vi "DetectorTest_MainV10.vi"() -> ()   [LabVIEW 2012]
uses:
  Detector IV/SMU Settings.ctl
  <vilib>/Utility/file.llb/Write To Spreadsheet File (string).vi
  <vilib>/Utility/file.llb/Read From Spreadsheet File (string).vi
  <vilib>/Utility/file.llb/Read From Spreadsheet File (DBL).vi
  <vilib>/Analysis/NI_AALBase.lvlib
panel:
  in  "Current Session":timestamp=timestamp(3388091786.578125 s since 1904-01-01)
  in  "new sesh":bool
  out "RecipeID":string="58"
  in  "Sweep Direction (Keysight)":i32(ring) items=["Up", "Down"]
  in  "Auto Adjust Compliance?":bool
  out "Auto Temp Counter":i32
  out "iteration":i32
  in  "Temp Data":T1={"Ambient Temperature"=20.38176242851337, "Chuck Set Temperature"=35.0} {"Chuck Set Temperature" format="%#.1g"; "Ambient Temperature" format="%#.1g"}
  in  "Wafer Info 3":T2={"Cell Name (Automatic)"="Open_Diode_1000", "Package"="", "Coating"="FOR_AIR", "Comment"="IV test for lot 371", "Flash Setup"="5500_99_03p5", "Hrs under test"=0.0}
  out "TempCounter":i32
  out "WaferCounter":i32
  in  "Profile Z":bool
  in  "Load Wafer":bool
  out "Raw Test Skipped":bool=TRUE
  out "device name w skip":string="Open_Diode_1000(skip)"
  in  "4-wire":bool
  out "Laser Counter":i32
  out "Output Power (mW)":dbl
  out "Counter":i32
  out "NameList":string[](array[string])
  in  "Wafer Info Flash 2":T3={"Cell Name"="5500_130_05", "Package"="", "Coating"="", "LRC?"=enum."J2", "Comment"="", "Hours Under Test"=0.0}
  in  "Parameters Flash 2":T4 {"Voc" format="%#_4g"; "Isc" format="%#_4g"; "FF" format="%#_4g"; "Imax" format="%#_4g"; "Vmax" format="%#_4g"; "Pmax" format="%#_4g"; "Itest" format="%#_4g"}
  in  "Wafer Info Flash":T3={"Cell Name"="Open_Diode_1000", "Package"="", "Coating"="", "LRC?"=enum."J2", "Comment"="", "Hours Under Test"=0.0}
  in  "Parameters Flash":T4={"Voc"=0.0, "Isc"=0.0, "FF"=0.0, "Vtest"=0.0, "Imax"=0.0, "Vmax"=0.0, "Pmax"=0.0, "Itest"=0.0, "Efficiency"=0.0, "Incident Power"=5.674, "Power Density (W/cm^2)"=0.6679328011361159, "Cell Area (cm²)"=849486.6535, "Number of AM1.5D Suns"=0.0, "Input Current (mA)"=40.0, "Equivalent 1 sun Jsc"=0.0} {"Voc" format="%#_4g"; "Isc" format="%#_4g"; "FF" format="%#_4g"; "Imax" format="%#_4g"; "Vmax" format="%#_4g"; "Pmax" format="%#_4g"; "Itest" format="%#_4g"}
  out "RawData file":path=path "C:/Users/Flash/Desktop/Data/Detector test data/SJC_ENG_371_4-GaAs/A-3719-2-A/Raw Data/A-3719-2-A_Open_Diode_1000_20180913075240.csv"
  out "Fine Cell Clusters":T5(array[cluster])=[{"Cell Name"="Open_Diode_1000", "X-coord"=46800.0, "Y-coord"=22950.0, "Area"=849486.6535, "Grid Shadowing"=0.0, "Xdim"=500.0, "Ydim"=500.0, "Mesa Area"=785398.1634}]
  out "Selected Data":cluster{dbl[], dbl[]}={[nan, nan, nan, nan, nan, nan, nan, nan, nan, nan, nan, nan, nan, nan, nan, nan, nan, nan, nan, nan, nan, nan, nan, nan, nan, nan, nan, nan, nan, nan, nan, nan, nan, nan, nan, nan, nan, nan, nan, nan, nan, nan, nan, nan, nan, nan, nan, nan, nan, nan, nan, nan, nan, nan, nan, nan, nan, nan, nan, nan, nan, nan, nan, nan, nan, nan, nan, nan, nan, nan, nan, nan, nan, nan, nan, nan, nan, nan, nan, nan, nan, nan, nan, nan], [nan, nan, nan, nan, nan, nan, nan, nan, nan, nan, nan, nan, nan, nan, nan, nan, nan, nan, nan, nan, nan, nan, nan, nan, nan, nan, nan, nan, nan, nan, nan, nan, nan, nan, nan, nan, nan, nan, nan, nan, nan, nan, nan, nan, nan, nan, nan, nan, nan, nan, nan, nan, nan, nan, nan, nan, nan, nan, nan, nan, nan, nan, nan, nan, nan, nan, nan, nan, nan, nan, nan, nan, nan, nan, nan, nan, nan, nan, nan, nan, nan, nan, nan, nan]}
  in  "Test Results 2":T6
  in  "Session Info 2":T7={"V set"=-1.0, "I compliance"=0.001, "J set"=0.01, "I set"=0.0, "V compliance"=1.0, "Laser Power (mW)"=0.0, "TestID"=0, "Session Time"=timestamp(0 s since 1904-01-01), "Operator"="Radek"} {"V compliance" format="%#_6f"; "I compliance" format="%#_6e"}
  in  "Die Info 2":T8={"Device Name"="", "ActiveArea_um2"=3848.451, "MesaArea_um2"=3848.451, "x"=0.0, "y"=0.0}
  in  "Wafer Info 2":T9
  in  "Test Results":T6={"I meas"=-1.83245e-12, "V meas"=6.01176, "Time"=timestamp(3619695820.3512325 s since 1904-01-01)}
  in  "Session Info":T7={"V set"=-6.0, "I compliance"=0.001, "J set"=0.01, "I set"=1.9634954079999997e-05, "V compliance"=6.0, "Laser Power (mW)"=0.0, "TestID"=1794, "Session Time"=timestamp(3619695160.866512 s since 1904-01-01), "Operator"="sswifter"} {"V compliance" format="%#_6f"; "I compliance" format="%#_6e"}
  in  "Die Info":T8={"Device Name"="Open_Diode_1000", "ActiveArea_um2"=849486.6535, "MesaArea_um2"=785398.1634, "x"=26800.0, "y"=72950.0}
  in  "Wafer Info":T9={"Wafer Name"="A-3719-2-A", "Scribe"="BJ325-089", "Mask"="PH001", "Lot"="SJC_ENG_371_4-GaAs"}
  in  "Name Array":string[](array[string])=["Wafer name", "Scribe", "Mask", "Lot", "Device name", "Active Area", "Mesa Area", "x", "y", "Imeas", "Vmeas", "Time", "Vset", "Icomp", "Jset", "Iset", "Vcomp", "Laser Power", "TestID", "SessionTime", "Operator", "Selected"]
  in  "TestID file":path=path "C:/Users/Flash/Documents/GitHub/labview/Detector IV/rawtest_log.csv"
  in  "update wafer":bool
  in  "Lot":string="SJC_ENG_382_4-GaAs"
  in  "Laser Current (mA)":dbl
  in  "Device Name":string="Open_Diode_3000"
  in  "Scribe":string="BP769-030XT"
  in  "MesaArea_um2":dbl=7068583.471
  out "Status":string="idle"
  out "error out":errorcluster
  in  "error in (no error)":errorcluster
  out "Manaul Plot 1":cluster{"V manual":dbl[], dbl[]}[](array[cluster])=[{"V manual"=[-0.1, -0.089741, -0.07949, -0.06923, -0.05897, -0.04872, -0.03846, -0.02821, -0.017951, -0.00769, 0.00256, 0.012819, 0.02308, 0.03333, 0.043589, 0.05385, 0.0641, 0.074359, 0.084619, 0.09487, 0.10513, 0.115379, 0.125639, 0.135899, 0.14615, 0.156409, 0.16667, 0.176919, 0.187179, 0.19744, 0.207691, 0.217949, 0.22821, 0.23846, 0.248719], [2.22891e-05, 1.84968e-05, 1.52529e-05, 1.24377e-05, 1.00378e-05, 7.9393e-06, 6.043e-06, 4.31347e-06, 2.71019e-06, 1.17492e-06, 3.32763e-07, 1.84722e-06, 3.41691e-06, 5.05009e-06, 6.8287e-06, 8.72018e-06, 1.07805e-05, 1.3036e-05, 1.55303e-05, 1.81749e-05, 2.11963e-05, 2.4467e-05, 2.80104e-05, 3.19022e-05, 3.6041e-05, 4.04887e-05, 4.53187e-05, 5.05479e-05, 5.60681e-05, 6.20483e-05, 6.8299e-05, 7.49314e-05, 8.20298e-05, 8.95166e-05, 9.72544e-05]}, {"V manual"=[-0.1, nan, nan, nan, nan, nan, nan, nan, nan, nan, nan, nan, nan, nan, nan, nan, nan, nan, nan, nan, nan, nan, nan, nan, nan, nan, nan, nan, nan, nan, nan, nan, nan, nan, nan, nan, nan, nan, nan, nan], [2.2117733333333333e-05, nan, nan, nan, nan, nan, nan, nan, nan, nan, nan, nan, nan, nan, nan, nan, nan, nan, nan, nan, nan, nan, nan, nan, nan, nan, nan, nan, nan, nan, nan, nan, nan, nan, nan, nan, nan, nan, nan, nan]}, {"V manual"=[0.23860433333333333, nan, nan, nan, nan, nan, nan, nan, nan, nan, nan, nan, nan, nan, nan, nan, nan, nan, nan, nan, nan, nan, nan, nan, nan, nan, nan, nan, nan, nan, nan, nan, nan, nan, nan, nan, nan, nan, nan, nan], [7.068583470999999e-05, nan, nan, nan, nan, nan, nan, nan, nan, nan, nan, nan, nan, nan, nan, nan, nan, nan, nan, nan, nan, nan, nan, nan, nan, nan, nan, nan, nan, nan, nan, nan, nan, nan, nan, nan, nan, nan, nan, nan]}]
  out "Manual Plot 0":cluster{"V manual":dbl[], "I manual":dbl[]}[](array[cluster])=[{"V manual"=[-0.1, -0.089741, -0.07949, -0.06923, -0.05897, -0.04872, -0.03846, -0.02821, -0.017951, -0.00769, 0.00256, 0.012819, 0.02308, 0.03333, 0.043589, 0.05385, 0.0641, 0.074359, 0.084619, 0.09487, 0.10513, 0.115379, 0.125639, 0.135899, 0.14615, 0.156409, 0.16667, 0.176919, 0.187179, 0.19744, 0.207691, 0.217949, 0.22821, 0.23846, 0.248719], "I manual"=[-2.22891e-05, -1.84968e-05, -1.52529e-05, -1.24377e-05, -1.00378e-05, -7.9393e-06, -6.043e-06, -4.31347e-06, -2.71019e-06, -1.17492e-06, 3.32763e-07, 1.84722e-06, 3.41691e-06, 5.05009e-06, 6.8287e-06, 8.72018e-06, 1.07805e-05, 1.3036e-05, 1.55303e-05, 1.81749e-05, 2.11963e-05, 2.4467e-05, 2.80104e-05, 3.19022e-05, 3.6041e-05, 4.04887e-05, 4.53187e-05, 5.05479e-05, 5.60681e-05, 6.20483e-05, 6.8299e-05, 7.49314e-05, 8.20298e-05, 8.95166e-05, 9.72544e-05]}, {"V manual"=[-0.1, nan, nan, nan, nan, nan, nan, nan, nan, nan, nan, nan, nan, nan, nan, nan, nan, nan, nan, nan, nan, nan, nan, nan, nan, nan, nan, nan, nan, nan, nan, nan, nan, nan, nan, nan, nan, nan, nan, nan], "I manual"=[-2.2117733333333333e-05, nan, nan, nan, nan, nan, nan, nan, nan, nan, nan, nan, nan, nan, nan, nan, nan, nan, nan, nan, nan, nan, nan, nan, nan, nan, nan, nan, nan, nan, nan, nan, nan, nan, nan, nan, nan, nan, nan, nan]}, {"V manual"=[0.23860433333333333, nan, nan, nan, nan, nan, nan, nan, nan, nan, nan, nan, nan, nan, nan, nan, nan, nan, nan, nan, nan, nan, nan, nan, nan, nan, nan, nan, nan, nan, nan, nan, nan, nan, nan, nan, nan, nan, nan, nan], "I manual"=[7.068583470999999e-05, nan, nan, nan, nan, nan, nan, nan, nan, nan, nan, nan, nan, nan, nan, nan, nan, nan, nan, nan, nan, nan, nan, nan, nan, nan, nan, nan, nan, nan, nan, nan, nan, nan, nan, nan, nan, nan, nan, nan]}]
  in  "Reset 1st die":bool
  in  "Sweep Settings":T10={"Channel"=enum."Channel A", "Vstart"=-0.1, "Vend"=0.3, "# of points"=40, "NPLC"=1.0, "I compliance"=0.0001, "Delay ms"=100.0}
  in  "Reset xy":bool
  out "current y":i32
  out "current x":i32=10000
  in  "sweep delay ms":dbl=100.0
  in  "I compliance sweep":dbl=0.0001
  in  "points":u16=80
  in  "V end":dbl=1.0
  in  "V start":dbl=-5.0
  in  "Repeat Vf":u32=3
  out "I set":dbl=7.068583470999999e-05
  in  "V compliance":dbl=0.5 format="%#_6f"
  in  "Vf delay ms":dbl=100.0
  in  "J set A/cm2":dbl=0.001
  in  "Repeat Id":u32=5
  in  "I compliance":dbl=0.001 format="%#_6e"
  in  "Id delay ms":dbl=500.0
  in  "V set":dbl=-0.1
  out "Vmeas Settings":T11={"Channel"=enum."Channel A", "Vset"=7.068583470999999e-05, "NPLC"=1.0, "I compliance"=0.3, "Repeat time"=1, "Delay ms"=100.0, "4-wire"=FALSE}
  out "Imeas Settings":T11={"Channel"=enum."Channel A", "Vset"=-0.1, "NPLC"=1.0, "I compliance"=0.001, "Repeat time"=5, "Delay ms"=500.0, "4-wire"=FALSE}
  out "Array of Cell Data Clusters":T12(array[cluster])=[{"Cell Name"="Open_Diode_3000", "X-coord"=0.0, "Y-coord"=0.0, "Area"=7258335.667, "Grid Shadowing"=0.0, "Ydim"=1500.0, "Xdim"=1500.0, "Meas Area"=7068583.471}, {"Cell Name"="Open_Diode_3000", "X-coord"=10000.0, "Y-coord"=0.0, "Area"=7258335.667, "Grid Shadowing"=0.0, "Ydim"=1500.0, "Xdim"=1500.0, "Meas Area"=7068583.471}, {"Cell Name"="Open_Diode_3000", "X-coord"=20000.0, "Y-coord"=0.0, "Area"=7258335.667, "Grid Shadowing"=0.0, "Ydim"=1500.0, "Xdim"=1500.0, "Meas Area"=7068583.471}, {"Cell Name"="Open_Diode_3000", "X-coord"=30000.0, "Y-coord"=0.0, "Area"=7258335.667, "Grid Shadowing"=0.0, "Ydim"=1500.0, "Xdim"=1500.0, "Meas Area"=7068583.471}, {"Cell Name"="Open_Diode_3000", "X-coord"=-10000.0, "Y-coord"=10000.0, "Area"=7258335.667, "Grid Shadowing"=0.0, "Ydim"=1500.0, "Xdim"=1500.0, "Meas Area"=7068583.471}, {"Cell Name"="Open_Diode_3000", "X-coord"=0.0, "Y-coord"=10000.0, "Area"=7258335.667, "Grid Shadowing"=0.0, "Ydim"=1500.0, "Xdim"=1500.0, "Meas Area"=7068583.471}, {"Cell Name"="Open_Diode_3000", "X-coord"=10000.0, "Y-coord"=10000.0, "Area"=7258335.667, "Grid Shadowing"=0.0, "Ydim"=1500.0, "Xdim"=1500.0, "Meas Area"=7068583.471}, {"Cell Name"="Open_Diode_3000", "X-coord"=40000.0, "Y-coord"=10000.0, "Area"=7258335.667, "Grid Shadowing"=0.0, "Ydim"=1500.0, "Xdim"=1500.0, "Meas Area"=7068583.471}, {"Cell Name"="Open_Diode_3000", "X-coord"=-20000.0, "Y-coord"=20000.0, "Area"=7258335.667, "Grid Shadowing"=0.0, "Ydim"=1500.0, "Xdim"=1500.0, "Meas Area"=7068583.471}, {"Cell Name"="Open_Diode_3000", "X-coord"=-10000.0, "Y-coord"=20000.0, "Area"=7258335.667, "Grid Shadowing"=0.0, "Ydim"=1500.0, "Xdim"=1500.0, "Meas Area"=7068583.471}, {"Cell Name"="Open_Diode_3000", "X-coord"=10000.0, "Y-coord"=20000.0, "Area"=7258335.667, "Grid Shadowing"=0.0, "Ydim"=1500.0, "Xdim"=1500.0, "Meas Area"=7068583.471}, {"Cell Name"="Open_Diode_3000", "X-coord"=20000.0, "Y-coord"=20000.0, "Area"=7258335.667, "Grid Shadowing"=0.0, "Ydim"=1500.0, "Xdim"=1500.0, "Meas Area"=7068583.471}, {"Cell Name"="Open_Diode_3000", "X-coord"=40000.0, "Y-coord"=20000.0, "Area"=7258335.667, "Grid Shadowing"=0.0, "Ydim"=1500.0, "Xdim"=1500.0, "Meas Area"=7068583.471}, {"Cell Name"="Open_Diode_3000", "X-coord"=50000.0, "Y-coord"=20000.0, "Area"=7258335.667, "Grid Shadowing"=0.0, "Ydim"=1500.0, "Xdim"=1500.0, "Meas Area"=7068583.471}, {"Cell Name"="Open_Diode_3000", "X-coord"=-20000.0, "Y-coord"=30000.0, "Area"=7258335.667, "Grid Shadowing"=0.0, "Ydim"=1500.0, "Xdim"=1500.0, "Meas Area"=7068583.471}, {"Cell Name"="Open_Diode_3000", "X-coord"=-10000.0, "Y-coord"=30000.0, "Area"=7258335.667, "Grid Shadowing"=0.0, "Ydim"=1500.0, "Xdim"=1500.0, "Meas Area"=7068583.471}, {"Cell Name"="Open_Diode_3000", "X-coord"=20000.0, "Y-coord"=30000.0, "Area"=7258335.667, "Grid Shadowing"=0.0, "Ydim"=1500.0, "Xdim"=1500.0, "Meas Area"=7068583.471}, {"Cell Name"="Open_Diode_3000", "X-coord"=30000.0, "Y-coord"=30000.0, "Area"=7258335.667, "Grid Shadowing"=0.0, "Ydim"=1500.0, "Xdim"=1500.0, "Meas Area"=7068583.471}, {"Cell Name"="Open_Diode_3000", "X-coord"=40000.0, "Y-coord"=30000.0, "Area"=7258335.667, "Grid Shadowing"=0.0, "Ydim"=1500.0, "Xdim"=1500.0, "Meas Area"=7068583.471}, {"Cell Name"="Open_Diode_3000", "X-coord"=50000.0, "Y-coord"=30000.0, "Area"=7258335.667, "Grid Shadowing"=0.0, "Ydim"=1500.0, "Xdim"=1500.0, "Meas Area"=7068583.471}, {"Cell Name"="Open_Diode_3000", "X-coord"=-20000.0, "Y-coord"=40000.0, "Area"=7258335.667, "Grid Shadowing"=0.0, "Ydim"=1500.0, "Xdim"=1500.0, "Meas Area"=7068583.471}, {"Cell Name"="Open_Diode_3000", "X-coord"=-10000.0, "Y-coord"=40000.0, "Area"=7258335.667, "Grid Shadowing"=0.0, "Ydim"=1500.0, "Xdim"=1500.0, "Meas Area"=7068583.471}, {"Cell Name"="Open_Diode_3000", "X-coord"=0.0, "Y-coord"=40000.0, "Area"=7258335.667, "Grid Shadowing"=0.0, "Ydim"=1500.0, "Xdim"=1500.0, "Meas Area"=7068583.471}, {"Cell Name"="Open_Diode_3000", "X-coord"=10000.0, "Y-coord"=40000.0, "Area"=7258335.667, "Grid Shadowing"=0.0, "Ydim"=1500.0, "Xdim"=1500.0, "Meas Area"=7068583.471}, {"Cell Name"="Open_Diode_3000", "X-coord"=40000.0, "Y-coord"=40000.0, "Area"=7258335.667, "Grid Shadowing"=0.0, "Ydim"=1500.0, "Xdim"=1500.0, "Meas Area"=7068583.471}, {"Cell Name"="Open_Diode_3000", "X-coord"=50000.0, "Y-coord"=40000.0, "Area"=7258335.667, "Grid Shadowing"=0.0, "Ydim"=1500.0, "Xdim"=1500.0, "Meas Area"=7068583.471}, {"Cell Name"="Open_Diode_3000", "X-coord"=-20000.0, "Y-coord"=50000.0, "Area"=7258335.667, "Grid Shadowing"=0.0, "Ydim"=1500.0, "Xdim"=1500.0, "Meas Area"=7068583.471}, {"Cell Name"="Open_Diode_3000", "X-coord"=-10000.0, "Y-coord"=50000.0, "Area"=7258335.667, "Grid Shadowing"=0.0, "Ydim"=1500.0, "Xdim"=1500.0, "Meas Area"=7068583.471}, {"Cell Name"="Open_Diode_3000", "X-coord"=10000.0, "Y-coord"=50000.0, "Area"=7258335.667, "Grid Shadowing"=0.0, "Ydim"=1500.0, "Xdim"=1500.0, "Meas Area"=7068583.471}, {"Cell Name"="Open_Diode_3000", "X-coord"=20000.0, "Y-coord"=50000.0, "Area"=7258335.667, "Grid Shadowing"=0.0, "Ydim"=1500.0, "Xdim"=1500.0, "Meas Area"=7068583.471}, {"Cell Name"="Open_Diode_3000", "X-coord"=40000.0, "Y-coord"=50000.0, "Area"=7258335.667, "Grid Shadowing"=0.0, "Ydim"=1500.0, "Xdim"=1500.0, "Meas Area"=7068583.471}, {"Cell Name"="Open_Diode_3000", "X-coord"=50000.0, "Y-coord"=50000.0, "Area"=7258335.667, "Grid Shadowing"=0.0, "Ydim"=1500.0, "Xdim"=1500.0, "Meas Area"=7068583.471}, {"Cell Name"="Open_Diode_3000", "X-coord"=-10000.0, "Y-coord"=60000.0, "Area"=7258335.667, "Grid Shadowing"=0.0, "Ydim"=1500.0, "Xdim"=1500.0, "Meas Area"=7068583.471}, {"Cell Name"="Open_Diode_3000", "X-coord"=20000.0, "Y-coord"=60000.0, "Area"=7258335.667, "Grid Shadowing"=0.0, "Ydim"=1500.0, "Xdim"=1500.0, "Meas Area"=7068583.471}, {"Cell Name"="Open_Diode_3000", "X-coord"=30000.0, "Y-coord"=60000.0, "Area"=7258335.667, "Grid Shadowing"=0.0, "Ydim"=1500.0, "Xdim"=1500.0, "Meas Area"=7068583.471}, {"Cell Name"="Open_Diode_3000", "X-coord"=40000.0, "Y-coord"=60000.0, "Area"=7258335.667, "Grid Shadowing"=0.0, "Ydim"=1500.0, "Xdim"=1500.0, "Meas Area"=7068583.471}, {"Cell Name"="Open_Diode_3000", "X-coord"=0.0, "Y-coord"=70000.0, "Area"=7258335.667, "Grid Shadowing"=0.0, "Ydim"=1500.0, "Xdim"=1500.0, "Meas Area"=7068583.471}, {"Cell Name"="Open_Diode_3000", "X-coord"=10000.0, "Y-coord"=70000.0, "Area"=7258335.667, "Grid Shadowing"=0.0, "Ydim"=1500.0, "Xdim"=1500.0, "Meas Area"=7068583.471}, {"Cell Name"="Open_Diode_3000", "X-coord"=20000.0, "Y-coord"=70000.0, "Area"=7258335.667, "Grid Shadowing"=0.0, "Ydim"=1500.0, "Xdim"=1500.0, "Meas Area"=7068583.471}, {"Cell Name"="Open_Diode_3000", "X-coord"=30000.0, "Y-coord"=70000.0, "Area"=7258335.667, "Grid Shadowing"=0.0, "Ydim"=1500.0, "Xdim"=1500.0, "Meas Area"=7068583.471}]
  in  "stop":bool
  in  "ActiveArea_um2":dbl=7258335.667
  in  "NPLC":dbl=1.0
  in  "Operator":string(combo)="tbilir"
  in  "Mask":string="PH001"
  in  "Wafer Name":string="A-3820-3-A"
  in  "Tab Control":T13(tab)
  in  "First Wafer Loaded?":bool
  in  "begin lot test":bool
  in  "Desired Wafer Name":string
  in  "Wafer List":i32(listbox)=-1
  in  "Add to wafer list":bool
  in  "Remove from wafer list":bool
  in  "Clear wafer list":bool
  in  "Generate Report":bool
  in  "Only Raw Test":bool
  in  "Clear Laser List":bool
  in  "Remove from Laser List":bool
  in  "Add to Laser":bool
  in  "Desired Current (mA)":dbl=40.0
  in  "Laser List":i32(listbox)=-1
  in  "Start auto":bool
  in  "Clear List":bool
  in  "Refresh Device":bool
  in  "Mask Name":string
  in  "Remove from List":bool
  in  "Add to list":bool
  in  "Available Device Name":string(combo)="Open_Diode_1000"
  in  "Test List":i32(listbox)=-1
  in  "Mask File all":path=path "C:/Users/Flash/Desktop/Mask Files/PH001 Detector GSG/PH001_Detector Aligner mask map file _ full top_open top 10_open top 5 diodes.csv"
  in  "Skip Raw Test?":bool
  in  "Test description":string="IV test for lot 371"
  in  "Clear temp list Auto":bool
  in  "Remove from Temp Auto":bool
  in  "Add to Temp Auto":bool
  in  "Auto Temp Set":dbl=25.0
  in  "Auto Temperature List":i32(listbox)=-1
  in  "Manual_Test":bool
  in  "Manual IV Plot settting":enum32{"Linear plot", "Log plot"}(radio)
  out "Vmeas manual":dbl=0.23860433333333333
  out "Imeas manual":dbl=-2.2117733333333333e-05
  out "Iarray manual":dbl[](array[numeric])=[-2.22891e-05, -1.84968e-05, -1.52529e-05, -1.24377e-05, -1.00378e-05, -7.9393e-06, -6.043e-06, -4.31347e-06, -2.71019e-06, -1.17492e-06, 3.32763e-07, 1.84722e-06, 3.41691e-06, 5.05009e-06, 6.8287e-06, 8.72018e-06, 1.07805e-05, 1.3036e-05, 1.55303e-05, 1.81749e-05, 2.11963e-05, 2.4467e-05, 2.80104e-05, 3.19022e-05, 3.6041e-05, 4.04887e-05, 4.53187e-05, 5.05479e-05, 5.60681e-05, 6.20483e-05, 6.8299e-05, 7.49314e-05, 8.20298e-05, 8.95166e-05, 9.72544e-05]
  out "Varray manual":dbl[](array[numeric])=[-0.1, -0.089741, -0.07949, -0.06923, -0.05897, -0.04872, -0.03846, -0.02821, -0.017951, -0.00769, 0.00256, 0.012819, 0.02308, 0.03333, 0.043589, 0.05385, 0.0641, 0.074359, 0.084619, 0.09487, 0.10513, 0.115379, 0.125639, 0.135899, 0.14615, 0.156409, 0.16667, 0.176919, 0.187179, 0.19744, 0.207691, 0.217949, 0.22821, 0.23846, 0.248719]
  out "y target":i32
  out "x target":i32=10000
  in  "Die Number":u16(ring)=1 items=["0", "1", "2", "3", "4", "5", "6", "7", "8", "9", "10", "11", "12", "13", "14", "15", "16", "17", "18", "19", "20", "21", "22", "23", "24", "25", "26", "27", "28", "29", "30", "31", "32", "33", "34", "35", "36", "37", "38", "39", "40", "41", "42", "43", "44", "45", "46", "47", "48", "49", "50", "51", "52", "53", "54", "55", "56", "57", "58", "59", "60", "61", "62", "63", "64", "65", "66", "67", "68", "69", "70", "71", "72", "73", "74", "75", "76", "77", "78", "79", "80", "81", "82", "83", "84", "85"]
  in  "load file":bool
  in  "Move to":bool
  in  "Mask File Manual":path=path "C:/Users/Flash/Desktop/Mask Files/PH001 Detector GSG/PH001_Detector Aligner mask map file _ full top_open top 10_open top 5 diodes_Open_Diode_3000.csv"
  out "Manual IV":cluster{"V manual":dbl[], "I manual":dbl[]}[](graph)=[{"V manual"=[-0.1, -0.089741, -0.07949, -0.06923, -0.05897, -0.04872, -0.03846, -0.02821, -0.017951, -0.00769, 0.00256, 0.012819, 0.02308, 0.03333, 0.043589, 0.05385, 0.0641, 0.074359, 0.084619, 0.09487, 0.10513, 0.115379, 0.125639, 0.135899, 0.14615, 0.156409, 0.16667, 0.176919, 0.187179, 0.19744, 0.207691, 0.217949, 0.22821, 0.23846, 0.248719], "I manual"=[-2.22891e-05, -1.84968e-05, -1.52529e-05, -1.24377e-05, -1.00378e-05, -7.9393e-06, -6.043e-06, -4.31347e-06, -2.71019e-06, -1.17492e-06, 3.32763e-07, 1.84722e-06, 3.41691e-06, 5.05009e-06, 6.8287e-06, 8.72018e-06, 1.07805e-05, 1.3036e-05, 1.55303e-05, 1.81749e-05, 2.11963e-05, 2.4467e-05, 2.80104e-05, 3.19022e-05, 3.6041e-05, 4.04887e-05, 4.53187e-05, 5.05479e-05, 5.60681e-05, 6.20483e-05, 6.8299e-05, 7.49314e-05, 8.20298e-05, 8.95166e-05, 9.72544e-05]}, {"V manual"=[-0.1, nan, nan, nan, nan, nan, nan, nan, nan, nan, nan, nan, nan, nan, nan, nan, nan, nan, nan, nan, nan, nan, nan, nan, nan, nan, nan, nan, nan, nan, nan, nan, nan, nan, nan, nan, nan, nan, nan, nan], "I manual"=[-2.2117733333333333e-05, nan, nan, nan, nan, nan, nan, nan, nan, nan, nan, nan, nan, nan, nan, nan, nan, nan, nan, nan, nan, nan, nan, nan, nan, nan, nan, nan, nan, nan, nan, nan, nan, nan, nan, nan, nan, nan, nan, nan]}, {"V manual"=[0.23860433333333333, nan, nan, nan, nan, nan, nan, nan, nan, nan, nan, nan, nan, nan, nan, nan, nan, nan, nan, nan, nan, nan, nan, nan, nan, nan, nan, nan, nan, nan, nan, nan, nan, nan, nan, nan, nan, nan, nan, nan], "I manual"=[7.068583470999999e-05, nan, nan, nan, nan, nan, nan, nan, nan, nan, nan, nan, nan, nan, nan, nan, nan, nan, nan, nan, nan, nan, nan, nan, nan, nan, nan, nan, nan, nan, nan, nan, nan, nan, nan, nan, nan, nan, nan, nan]}]
  in  "Measure 2 Point?":bool=TRUE
  in  "Manual Test Comments":string="IV test for lot 371"
  in  "Load raw":bool
  in  "Select":bool
  in  "Number Select":u16=10
  in  "Vmax":dbl=0.285
  in  "Vmin":dbl=0.05
  out "Test FileName":string="A-3719-2-A_Open_Diode_1000_20180913075240.csv"
  out "RawTest ID":u32=2029
  out "Progress":u8(slide)=99 scale=0.0..100.0
  out "Current Device":u32=84
  out "Total Device":u32=84
  out "V meas":dbl[](array[numeric])=[6.01142, 6.01054, 6.01089, 0.000137925, 6.01222, 6.01216, 6.01145, 6.01193, 6.0103, 6.01103, 6.01162, 6.01132, 6.01127, 6.01137, 6.01132, 6.01125, 6.01108, 6.01134, 6.01154, 6.01135, 6.01146, 6.01204, 6.01111, 6.01101, 6.01053, 6.01143, 6.01152, 6.01128, 6.00993, 6.00994, 6.01042, 3.58707, 6.01175, 6.01164, 6.01056, 6.01166, 6.01073, 6.01098, 6.01142, 6.01026, 6.01071, 6.01116, 6.01174, 6.01214, 6.01026, 6.01093, 5.99486, 6.01138, 6.01091, 6.01133, 6.01086, 6.01094, 6.01192, 6.01232, 6.01069, 6.01162, 6.01233, 6.01184, 6.0022, 5.17964, 6.01156, 6.01223, 6.01107, 6.0102, 6.0108, 6.01164, 5.75188, 5.06441, 6.01144, 6.01129, 6.01161, 6.01159, 6.01096, 5.61419, 5.16536, 6.01197, 6.01142, 6.01186, 6.01133, 6.01132, 6.01119, 6.01113, 5.83632, 6.01176]
  out "I meas":dbl[](array[numeric])=[-3.868033999999999e-11, -1.2052780000000002e-09, -6.028065999999999e-11, -0.0009999796, -3.0170019999999996e-11, -4.752688e-11, -4.8625459999999994e-11, -3.7159980000000005e-11, -1.7203160000000002e-07, -2.00883e-08, -7.974548e-11, -3.897576e-11, -3.555112e-11, -2.188194e-08, -5.2771619999999994e-11, -2.9935519999999994e-11, -3.295828e-11, -5.707007999999999e-08, -4.796104e-07, -2.002028e-08, -7.080146e-08, -4.18e-11, -2.108774e-11, -4.09959e-11, -4.424556e-11, -3.3264100000000003e-09, -2.0351338000000002e-10, -6.144901999999999e-09, -4.3002719999999993e-11, -3.898936e-09, -2.0389360000000002e-11, -2.049748e-08, -6.527374000000001e-10, -1.0336196000000001e-10, -2.697004e-11, -3.376518e-08, -6.171924e-11, -2.02069e-10, -1.200538e-09, -2.8179300000000003e-11, -6.537938e-10, -5.153115999999999e-11, -2.8508420000000003e-09, -7.534774e-07, -2.636916e-07, -1.446754e-09, -9.464432000000001e-11, -1.0602588000000001e-10, -4.217728e-11, -7.227086e-08, -3.990094e-11, -2.7389038000000002e-11, -1.90881e-07, -2.2892700000000004e-12, -4.745506e-08, -4.579318e-11, -4.5842860000000003e-11, -5.953868e-11, -3.758154e-11, -4.4363539999999995e-09, -7.143562e-11, -1.397812e-10, -7.11463e-11, -5.56664e-11, -2.6296820000000003e-08, -1.1582659999999999e-07, -2.317642e-11, -5.807276000000001e-11, -2.17813e-12, -5.7970201999999995e-11, -6.71486e-11, -8.667722000000001e-12, 3.2483739999999993e-12, -6.306573999999999e-11, -8.307524e-11, -2.4324079999999998e-12, -2.795726e-12, -2.185576e-12, -2.0225460000000002e-12, -2.122472e-12, -1.6340760000000001e-06, -2.5727129999999997e-06, -3.269066e-11, -1.83245e-12]
  in  "RawData Save Path":path=path "C:/Users/Flash/Desktop/Data/Detector test data"
  in  "StartRaw":bool
  out "Vforward hist":T14(graph)={"X Values"=[0.30074752875, 0.90196673625, 1.5031859437500001, 2.10440515125, 2.70562435875, 3.3068435662500004, 3.90806277375, 4.50928198125, 5.110501188750001, 5.7117203962500005], "Histogram: h(x)"=[1, 0, 0, 0, 0, 1, 0, 0, 3, 79]}
  out "Idark hist":T14(graph)={"X Values"=[-0.0009499806198375813, -0.0008499826595127439, -0.0007499846991879066, -0.0006499867388630691, -0.0005499887785382317, -0.0004499908182133943, -0.0003499928578885569, -0.0002499948975637195, -0.0001499969372388821, -4.99989769140447e-05], "Histogram: h(x)"=[1, 0, 0, 0, 0, 0, 0, 0, 0, 83]}
  in  "Mask File Raw":path=path "C:/Users/Flash/Desktop/Mask Files/PH001 Detector GSG/PH001_Detector Aligner mask map file _ full top_open top 10_open top 5 diodes_Open_Diode_3000.csv"
  out "Spec Plot":cluster{"V meas":dbl[], "I meas":dbl[]}[](graph)=[{"V meas"=[6.01142, 6.01054, 6.01089, 0.000137925, 6.01222, 6.01216, 6.01145, 6.01193, 6.0103, 6.01103, 6.01162, 6.01132, 6.01127, 6.01137, 6.01132, 6.01125, 6.01108, 6.01134, 6.01154, 6.01135, 6.01146, 6.01204, 6.01111, 6.01101, 6.01053, 6.01143, 6.01152, 6.01128, 6.00993, 6.00994, 6.01042, 3.58707, 6.01175, 6.01164, 6.01056, 6.01166, 6.01073, 6.01098, 6.01142, 6.01026, 6.01071, 6.01116, 6.01174, 6.01214, 6.01026, 6.01093, 5.99486, 6.01138, 6.01091, 6.01133, 6.01086, 6.01094, 6.01192, 6.01232, 6.01069, 6.01162, 6.01233, 6.01184, 6.0022, 5.17964, 6.01156, 6.01223, 6.01107, 6.0102, 6.0108, 6.01164, 5.75188, 5.06441, 6.01144, 6.01129, 6.01161, 6.01159, 6.01096, 5.61419, 5.16536, 6.01197, 6.01142, 6.01186, 6.01133, 6.01132, 6.01119, 6.01113, 5.83632, 6.01176], "I meas"=[-3.868033999999999e-11, -1.2052780000000002e-09, -6.028065999999999e-11, -0.0009999796, -3.0170019999999996e-11, -4.752688e-11, -4.8625459999999994e-11, -3.7159980000000005e-11, -1.7203160000000002e-07, -2.00883e-08, -7.974548e-11, -3.897576e-11, -3.555112e-11, -2.188194e-08, -5.2771619999999994e-11, -2.9935519999999994e-11, -3.295828e-11, -5.707007999999999e-08, -4.796104e-07, -2.002028e-08, -7.080146e-08, -4.18e-11, -2.108774e-11, -4.09959e-11, -4.424556e-11, -3.3264100000000003e-09, -2.0351338000000002e-10, -6.144901999999999e-09, -4.3002719999999993e-11, -3.898936e-09, -2.0389360000000002e-11, -2.049748e-08, -6.527374000000001e-10, -1.0336196000000001e-10, -2.697004e-11, -3.376518e-08, -6.171924e-11, -2.02069e-10, -1.200538e-09, -2.8179300000000003e-11, -6.537938e-10, -5.153115999999999e-11, -2.8508420000000003e-09, -7.534774e-07, -2.636916e-07, -1.446754e-09, -9.464432000000001e-11, -1.0602588000000001e-10, -4.217728e-11, -7.227086e-08, -3.990094e-11, -2.7389038000000002e-11, -1.90881e-07, -2.2892700000000004e-12, -4.745506e-08, -4.579318e-11, -4.5842860000000003e-11, -5.953868e-11, -3.758154e-11, -4.4363539999999995e-09, -7.143562e-11, -1.397812e-10, -7.11463e-11, -5.56664e-11, -2.6296820000000003e-08, -1.1582659999999999e-07, -2.317642e-11, -5.807276000000001e-11, -2.17813e-12, -5.7970201999999995e-11, -6.71486e-11, -8.667722000000001e-12, 3.2483739999999993e-12, -6.306573999999999e-11, -8.307524e-11, -2.4324079999999998e-12, -2.795726e-12, -2.185576e-12, -2.0225460000000002e-12, -2.122472e-12, -1.6340760000000001e-06, -2.5727129999999997e-06, -3.269066e-11, -1.83245e-12]}, {"V meas"=[3.58707, nan, nan, nan, nan, nan, nan, nan, nan, nan, nan, nan, nan, nan, nan, nan, nan, nan, nan, nan, nan, nan, nan, nan, nan, nan, nan, nan, nan, nan, nan, nan, nan, nan, nan, nan, nan, nan, nan, nan, nan, nan, nan, nan, nan, nan, nan, nan, nan, nan, nan, nan, nan, nan, nan, nan, nan, nan, nan, nan, nan, nan, nan, nan, nan, nan, nan, nan, nan, nan, nan, nan, nan, nan, nan, nan, nan, nan, nan, nan, nan, nan, nan, nan], "I meas"=[-2.049748e-08, nan, nan, nan, nan, nan, nan, nan, nan, nan, nan, nan, nan, nan, nan, nan, nan, nan, nan, nan, nan, nan, nan, nan, nan, nan, nan, nan, nan, nan, nan, nan, nan, nan, nan, nan, nan, nan, nan, nan, nan, nan, nan, nan, nan, nan, nan, nan, nan, nan, nan, nan, nan, nan, nan, nan, nan, nan, nan, nan, nan, nan, nan, nan, nan, nan, nan, nan, nan, nan, nan, nan, nan, nan, nan, nan, nan, nan, nan, nan, nan, nan, nan, nan]}]
  in  "Explore Data":bool
  out "no file":bool
  in  "Comments":string="IV test for lot 371"
  in  "FineTest save path":path=path "C:/Users/Flash/Desktop/Data/Detector test data"
  out "I fine":dbl[](array[numeric])=[-2.70504e-08, -2.32087e-08, -1.94015e-08, -1.62001e-08, -1.3396e-08, -1.06144e-08, -8.14274e-09, -5.83125e-09, -3.66964e-09, -2.05099e-09, -1.05505e-09, -6.56038e-10, -4.43558e-10, -3.24538e-10, -2.3071e-10, -1.84326e-10, -1.50747e-10, -1.31042e-10, -1.1589e-10, -1.0217e-10, -9.29752e-11, -8.22993e-11, -7.74358e-11, -6.84813e-11, -6.19634e-11, -5.51294e-11, -4.86827e-11, -4.15262e-11, -3.40749e-11, -2.82174e-11, -2.14966e-11, -1.33787e-11, -7.37435e-12, -5.50663e-12, 4.69868e-12, 1.38179e-11, 4.52471e-11, 2.99241e-10, 1.96981e-09, 2.81104e-08]
  out "V fine":dbl[](array[numeric])=[-6.0, -5.82051, -5.64103, -5.46154, -5.28205, -5.10256, -4.92308, -4.74359, -4.5641, -4.38461, -4.20513, -4.02564, -3.84615, -3.66667, -3.48718, -3.30769, -3.1282, -2.94872, -2.76923, -2.58974, -2.41026, -2.23077, -2.05128, -1.87179, -1.69231, -1.51282, -1.33333, -1.15384, -0.974358, -0.79487, -0.615383, -0.435896, -0.256409, -0.0769218, 0.102565, 0.282053, 0.46154, 0.641027, 0.820514, 1.0]
  out "Current Device":u32=1
  out "Total Device":u32=1
  out "IV fine log":cluster{dbl[], dbl[]}[](graph)=[{[-6.0, -5.82051, -5.64103, -5.46154, -5.28205, -5.10256, -4.92308, -4.74359, -4.5641, -4.38461, -4.20513, -4.02564, -3.84615, -3.66667, -3.48718, -3.30769, -3.1282, -2.94872, -2.76923, -2.58974, -2.41026, -2.23077, -2.05128, -1.87179, -1.69231, -1.51282, -1.33333, -1.15384, -0.974358, -0.79487, -0.615383, -0.435896, -0.256409, -0.0769218, 0.102565, 0.282053, 0.46154, 0.641027, 0.820514, 1.0], [2.70504e-08, 2.32087e-08, 1.94015e-08, 1.62001e-08, 1.3396e-08, 1.06144e-08, 8.14274e-09, 5.83125e-09, 3.66964e-09, 2.05099e-09, 1.05505e-09, 6.56038e-10, 4.43558e-10, 3.24538e-10, 2.3071e-10, 1.84326e-10, 1.50747e-10, 1.31042e-10, 1.1589e-10, 1.0217e-10, 9.29752e-11, 8.22993e-11, 7.74358e-11, 6.84813e-11, 6.19634e-11, 5.51294e-11, 4.86827e-11, 4.15262e-11, 3.40749e-11, 2.82174e-11, 2.14966e-11, 1.33787e-11, 7.37435e-12, 5.50663e-12, 4.69868e-12, 1.38179e-11, 4.52471e-11, 2.99241e-10, 1.96981e-09, 2.81104e-08]}]
  out "Progress 2":u8(slide)=100 scale=0.0..100.0
  in  "StartFine":bool
  out "IV fine linear":cluster{dbl[], dbl[]}[](graph)=[{[-6.0, -5.82051, -5.64103, -5.46154, -5.28205, -5.10256, -4.92308, -4.74359, -4.5641, -4.38461, -4.20513, -4.02564, -3.84615, -3.66667, -3.48718, -3.30769, -3.1282, -2.94872, -2.76923, -2.58974, -2.41026, -2.23077, -2.05128, -1.87179, -1.69231, -1.51282, -1.33333, -1.15384, -0.974358, -0.79487, -0.615383, -0.435896, -0.256409, -0.0769218, 0.102565, 0.282053, 0.46154, 0.641027, 0.820514, 1.0], [-2.70504e-08, -2.32087e-08, -1.94015e-08, -1.62001e-08, -1.3396e-08, -1.06144e-08, -8.14274e-09, -5.83125e-09, -3.66964e-09, -2.05099e-09, -1.05505e-09, -6.56038e-10, -4.43558e-10, -3.24538e-10, -2.3071e-10, -1.84326e-10, -1.50747e-10, -1.31042e-10, -1.1589e-10, -1.0217e-10, -9.29752e-11, -8.22993e-11, -7.74358e-11, -6.84813e-11, -6.19634e-11, -5.51294e-11, -4.86827e-11, -4.15262e-11, -3.40749e-11, -2.82174e-11, -2.14966e-11, -1.33787e-11, -7.37435e-12, -5.50663e-12, 4.69868e-12, 1.38179e-11, 4.52471e-11, 2.99241e-10, 1.96981e-09, 2.81104e-08]}]
  in  "Mask File Fine":path=path "C:/Users/Flash/Desktop/Data/Detector test data/SJC_ENG_371_4-GaAs/A-3719-2-A/Raw Data/PH001_Detector Aligner mask map file _ full top_open top 10_open top 5 diodes_Open_Diode_1000_A-3719-2-A_091318_080341.5AM.csv"
  out "Y":dbl
  out "X":dbl
  in  "move prober 2":bool
  in  "load file for temp series":bool
  in  "Mask File Temperature":path=path "C:/Users/Flash/Desktop/Data/Detector test data/PH001 Detector Aligner mask map file _ full top_open top 10_open top 5 diodes_Open_Diode_5_300_A-3605-1-A_052518_113739.0AM.csv"
  out "IV temp linear":cluster{dbl[], dbl[]}[](graph)
  in  "Start temp":bool
  out "IV temp log":cluster{dbl[], dbl[]}[](graph)
  out "V fine temp":dbl[](array[numeric])=[-1.5, -1.45128, -1.40256, -1.35385, -1.30513, -1.25641, -1.20769, -1.15897, -1.11026, -1.06154, -1.01282, -0.964102, -0.915384, -0.866666, -0.817948, -0.76923, -0.720512, -0.671794, -0.623076, -0.574358, -0.52564, -0.476923, -0.428205, -0.379487, -0.330769, -0.282051, -0.233333, -0.184615, -0.135897, -0.087179, -0.038461, 0.0102569, 0.0589749, 0.107693, 0.156411, 0.205129, 0.253847, 0.302565, 0.351283, 0.400001]
  out "I fine temp":dbl[](array[numeric])=[-1.28772e-07, -1.20805e-07, -1.15592e-07, -1.10987e-07, -1.06412e-07, -1.02022e-07, -4.62038e-08, -9.34188e-08, -8.97462e-08, -8.60003e-08, -8.23237e-08, -7.87101e-08, -7.52945e-08, -7.18306e-08, -6.85145e-08, -6.5287e-08, -6.2088e-08, -5.90038e-08, -5.59938e-08, -5.29941e-08, -5.00661e-08, -4.71812e-08, -4.43421e-08, -4.15389e-08, -3.87298e-08, -3.5945e-08, -3.31511e-08, -3.027e-08, -2.71168e-08, -2.30654e-08, -1.54139e-08, 7.82768e-09, 2.30625e-07, 5.07951e-07, 2.21662e-06, 9.15235e-06, 3.37902e-05, 9.47719e-05, 0.000202989, 0.000357986]
  in  "Temperature Series save path":path=path "C:/Users/Flash/Desktop/Data/Detector test data"
  in  "Comments Temp":string
  in  "Single Device Temperature List":i32(listbox)=-1
  in  "Desired Temperature":dbl=25.0
  in  "Add to Temp":bool
  in  "Remove from Temp":bool
  in  "Clear temp list":bool
  in  "Desired Device":u16(ring)=50 items=["0", "1", "2", "3", "4", "5", "6", "7", "8", "9"]
  in  "Channel Keysight":dbl
  in  "Keysight SMU":refnum<visa-resource-name>="GPIB0::23::INSTR"
  in  "update temp":bool
  out "Current Temp":string="0\r"
  in  "Temp Setpoint":string="25"
  in  "Temptronics VISA":refnum<visa-resource-name>="GPIB0::9::INSTR"
  in  "Prober GPIB":string="0:1"
  in  "Keithley SMU":refnum<visa-resource-name>="GPIB0::26::INSTR"
  in  "Channel":enum32{"Channel A", "Channel B"}(ring)
  out "Calibration":cluster{"Y":dbl[], "Y":dbl[]}[](graph)=[{"Y"=[0.1, 0.2, 0.3, 0.4, 0.5, 0.6, 0.7, 0.8, 0.9, 1.0, 1.1, 1.2, 1.3, 1.4, 1.5, 1.6, 1.7, 1.8, 1.9, 2.0, 2.1, 2.2, 2.3, 2.4, 2.5, 2.6, 2.7, 2.8, 2.9, 3.0, 3.1, 3.2, 3.3, 3.4, 3.5, 3.6, 3.7, 3.8, 3.9, 4.0, 4.1, 4.2, 4.3, 4.4, 4.5, 4.6, 4.7, 4.8, 4.9, 5.0, 5.1, 5.2, 5.3, 5.4, 5.5, 5.6, 5.7, 5.8, 5.9, 6.0, 6.1, 6.2, 6.3, 6.4, 6.5, 6.6, 6.7, 6.8, 6.9, 7.0, 7.1, 7.2, 7.3, 7.4, 7.5, 7.6, 7.7, 7.8, 7.9, 8.0, 8.1, 8.2, 8.3, 8.4, 8.5, 8.6, 8.7, 8.8, 8.9, 9.0, 9.1, 9.2, 9.3, 9.4, 9.5, 9.6, 9.7, 9.8, 9.9, 10.0, 10.1, 10.2, 10.3, 10.4, 10.5, 10.6, 10.7, 10.8, 10.9, 11.0, 11.1, 11.2, 11.3, 11.4, 11.5, 11.6, 11.7, 11.8, 11.9, 12.0, 12.1, 12.2, 12.3, 12.4, 12.5, 12.6, 12.7, 12.8, 12.9, 13.0, 13.1, 13.2, 13.3, 13.4, 13.5, 13.6, 13.7, 13.8, 13.9, 14.0, 14.1, 14.2, 14.3, 14.4, 14.5, 14.6, 14.7, 14.8, 14.9, 15.0, 15.1, 15.2, 15.3, 15.4, 15.5, 15.6, 15.7, 15.8, 15.9, 16.0, 16.1, 16.2, 16.3, 16.4, 16.5, 16.6, 16.7, 16.8, 16.9, 17.0, 17.1, 17.2, 17.3, 17.4, 17.5, 17.6, 17.7, 17.8, 17.9, 18.0, 18.1, 18.2, 18.3, 18.4, 18.5, 18.6, 18.7, 18.8, 18.9, 19.0, 19.1, 19.2, 19.3, 19.4, 19.5, 19.6, 19.7, 19.8, 19.9, 20.0, 20.1, 20.2, 20.3, 20.4, 20.5, 20.6, 20.7, 20.8, 20.9, 21.0, 21.1, 21.2, 21.3, 21.4, 21.5, 21.6, 21.7, 21.8, 21.9, 22.0, 22.1, 22.2, 22.3, 22.4, 22.5, 22.6, 22.7, 22.8, 22.9, 23.0, 23.1, 23.2, 23.3, 23.4, 23.5, 23.6, 23.7, 23.8, 23.9, 24.0, 24.1, 24.2, 24.3, 24.4, 24.5, 24.6, 24.7, 24.8, 24.9, 25.0, 25.1, 25.2, 25.3, 25.4, 25.5, 25.6, 25.7, 25.8, 25.9, 26.0, 26.1, 26.2, 26.3, 26.4, 26.5, 26.6, 26.7, 26.8, 26.9, 27.0, 27.1, 27.2, 27.3, 27.4, 27.5, 27.6, 27.7, 27.8, 27.9, 28.0, 28.1, 28.2, 28.3, 28.4, 28.5, 28.6, 28.7, 28.8, 28.9, 29.0, 29.1, 29.2, 29.3, 29.4, 29.5, 29.6, 29.7, 29.8, 29.9, 30.0, 30.1, 30.2, 30.3, 30.4, 30.5, 30.6, 30.7, 30.8, 30.9, 31.0, 31.1, 31.2, 31.3, 31.4, 31.5, 31.6, 31.7, 31.8, 31.9, 32.0, 32.1, 32.2, 32.3, 32.4, 32.5, 32.6, 32.7, 32.8, 32.9, 33.0, 33.1, 33.2, 33.3, 33.4, 33.5, 33.6, 33.7, 33.8, 33.9, 34.0, 34.1, 34.2, 34.3, 34.4, 34.5, 34.6, 34.7, 34.8, 34.9, 35.0, 35.1, 35.2, 35.3, 35.4, 35.5, 35.6, 35.7, 35.8, 35.9, 36.0, 36.1, 36.2, 36.3, 36.4, 36.5, 36.6, 36.7, 36.8, 36.9, 37.0, 37.1, 37.2, 37.3, 37.4, 37.5, 37.6, 37.7, 37.8, 37.9, 38.0, 38.1, 38.2, 38.3, 38.4, 38.5, 38.6, 38.7, 38.8, 38.9, 39.0, 39.1, 39.2, 39.3, 39.4, 39.5, 39.6, 39.7, 39.8, 39.9, 40.0], "Y"=[0.0, 0.0, 0.0, 0.0, 0.0, 0.0, 0.0, 0.0, 0.0, 0.0, 0.0, 0.0, 0.0, 0.0, 0.0, 0.0, 0.0, 0.001, 0.001, 0.001, 0.001, 0.001, 0.001, 0.001, 0.001, 0.001, 0.001, 0.001, 0.001, 0.001, 0.001, 0.001, 0.001, 0.002, 0.002, 0.002, 0.002, 0.002, 0.002, 0.002, 0.002, 0.002, 0.002, 0.003, 0.003, 0.003, 0.003, 0.003, 0.003, 0.004, 0.004, 0.004, 0.004, 0.004, 0.005, 0.005, 0.005, 0.005, 0.006, 0.006, 0.006, 0.007, 0.007, 0.007, 0.008, 0.008, 0.008, 0.009, 0.009, 0.01, 0.01, 0.011, 0.011, 0.012, 0.012, 0.013, 0.013, 0.014, 0.015, 0.016, 0.017, 0.019, 0.023, 0.037, 0.058, 0.075, 0.091, 0.109, 0.127, 0.149, 0.168, 0.185, 0.202, 0.22, 0.243, 0.261, 0.279, 0.297, 0.314, 0.332, 0.354, 0.372, 0.391, 0.409, 0.427, 0.449, 0.466, 0.485, 0.503, 0.522, 0.544, 0.561, 0.579, 0.597, 0.615, 0.633, 0.658, 0.674, 0.692, 0.71, 0.728, 0.751, 0.768, 0.787, 0.807, 0.824, 0.845, 0.862, 0.88, 0.899, 0.918, 0.933, 0.957, 0.976, 0.993, 1.012, 1.029, 1.051, 1.07, 1.089, 1.103, 1.124, 1.145, 1.165, 1.183, 1.202, 1.217, 1.239, 1.256, 1.276, 1.294, 1.315, 1.333, 1.356, 1.376, 1.389, 1.405, 1.43, 1.45, 1.467, 1.485, 1.508, 1.524, 1.546, 1.56, 1.579, 1.598, 1.614, 1.631, 1.656, 1.679, 1.695, 1.715, 1.731, 1.75, 1.769, 1.791, 1.801, 1.824, 1.84, 1.865, 1.881, 1.897, 1.912, 1.93, 1.953, 1.974, 1.993, 2.006, 2.028, 2.052, 2.073, 2.087, 2.105, 2.125, 2.146, 2.164, 2.186, 2.203, 2.213, 2.243, 2.258, 2.276, 2.296, 2.311, 2.328, 2.35, 2.366, 2.389, 2.412, 2.426, 2.45, 2.459, 2.476, 2.502, 2.522, 2.53, 2.561, 2.571, 2.593, 2.609, 2.626, 2.652, 2.666, 2.691, 2.704, 2.729, 2.74, 2.764, 2.782, 2.807, 2.817, 2.837, 2.854, 2.869, 2.886, 2.908, 2.937, 2.947, 2.979, 2.988, 3.002, 3.033, 3.043, 3.064, 3.075, 3.1, 3.111, 3.145, 3.156, 3.181, 3.196, 3.212, 3.232, 3.246, 3.273, 3.289, 3.299, 3.327, 3.35, 3.371, 3.374, 3.4, 3.418, 3.45, 3.462, 3.483, 3.499, 3.516, 3.531, 3.55, 3.564, 3.592, 3.608, 3.629, 3.662, 3.674, 3.693, 3.717, 3.727, 3.752, 3.772, 3.78, 3.804, 3.82, 3.838, 3.87, 3.871, 3.889, 3.91, 3.938, 3.945, 3.97, 3.981, 4.008, 4.023, 4.048, 4.058, 4.076, 4.113, 4.131, 4.144, 4.172, 4.183, 4.199, 4.227, 4.24, 4.258, 4.285, 4.301, 4.32, 4.316, 4.347, 4.38, 4.395, 4.4, 4.426, 4.449, 4.458, 4.471, 4.488, 4.507, 4.529, 4.555, 4.571, 4.584, 4.624, 4.629, 4.654, 4.684, 4.686, 4.715, 4.731, 4.733, 4.756, 4.781, 4.791, 4.815, 4.82, 4.847, 4.864, 4.89, 4.907, 4.923, 4.935, 4.976, 4.983, 5.002, 5.022, 5.05, 5.065, 5.074, 5.082, 5.1, 5.123, 5.154, 5.154, 5.187, 5.22, 5.239, 5.253, 5.261, 5.278, 5.285, 5.316, 5.333, 5.363, 5.375, 5.388, 5.405, 5.426, 5.432, 5.455, 5.493, 5.508, 5.516, 5.539, 5.54, 5.569, 5.584, 5.594, 5.623, 5.639, 5.678, 5.667, 5.689, 5.724, 5.742, 5.738, 5.771, 5.806, 5.814, 5.826, 5.847, 5.852, 5.877, 5.906, 5.912, 5.934, 5.958]}]
  out "Laser Error":errorcluster caption="error out" {"code" format="%.0x"}
  in  "Load Calibration File":path=path "C:/Users/Flash/Desktop/Laser Calibration Files/Calib7_23_18.csv"
  in  "TL4000 In":refnum<visa-resource-name>="USB0::0x1313::0x804F::M00445403::INSTR" caption="resource name"
  in  "Enable Laser":bool=TRUE
  out "Raw Test Filename":path=path "C:/Users/Flash/Desktop/Data/Detector test data/SJC_ENG_371_4-GaAs/A-3719-2-A/Raw Data/A-3719-2-A_Open_Diode_1000_20180913075240.csv"
  out "new raw data save path":path=path "C:/Users/Flash/Desktop/Data/Detector test data/SJC_ENG_371_4-GaAs/A-3719-2-A/Raw Data"
  out "Error Out":errorcluster
  in  "Wait after load":u32
  in  "Keysight":bool
  out "Temp Controller Found":bool
  out "Keithley SMU Found":bool
  out "Keysight SMU Found":bool=TRUE
  out "Thorlabs Laser Found":bool=TRUE
  out "EG Prober Found":bool=TRUE
  out "Test Type":string="Auto Test"
  in  "Update viewer":bool
  in  "Logview":i32(listbox)=-1
  in  "Add Comments":string
  in  "Save Comment":bool
  out "Last Measurement":T15={"result string"="9_13_2018", "time string"="11:39 AM", "Wafer Name"="A-3719-2-A", "Operator"="sswifter", "Test description"="IV test for lot 371", "Test Type"="Auto Test"}
  in  "Measurement Log Path":path=path "C:/Users/Flash/Desktop/Data/Detector test data/MeasurementLog.csv"
  # "0 is for dark IV!"
  # "Sweep Settings"
  # "Forward Voltage"
  # "Dark/Light Current"
  # "Check settings before click start!"
  # "Make sure current x and y are same as prober before click Start!"
  # "TEC Control"
  # "TL4000 Settings"
  # "Keithley"
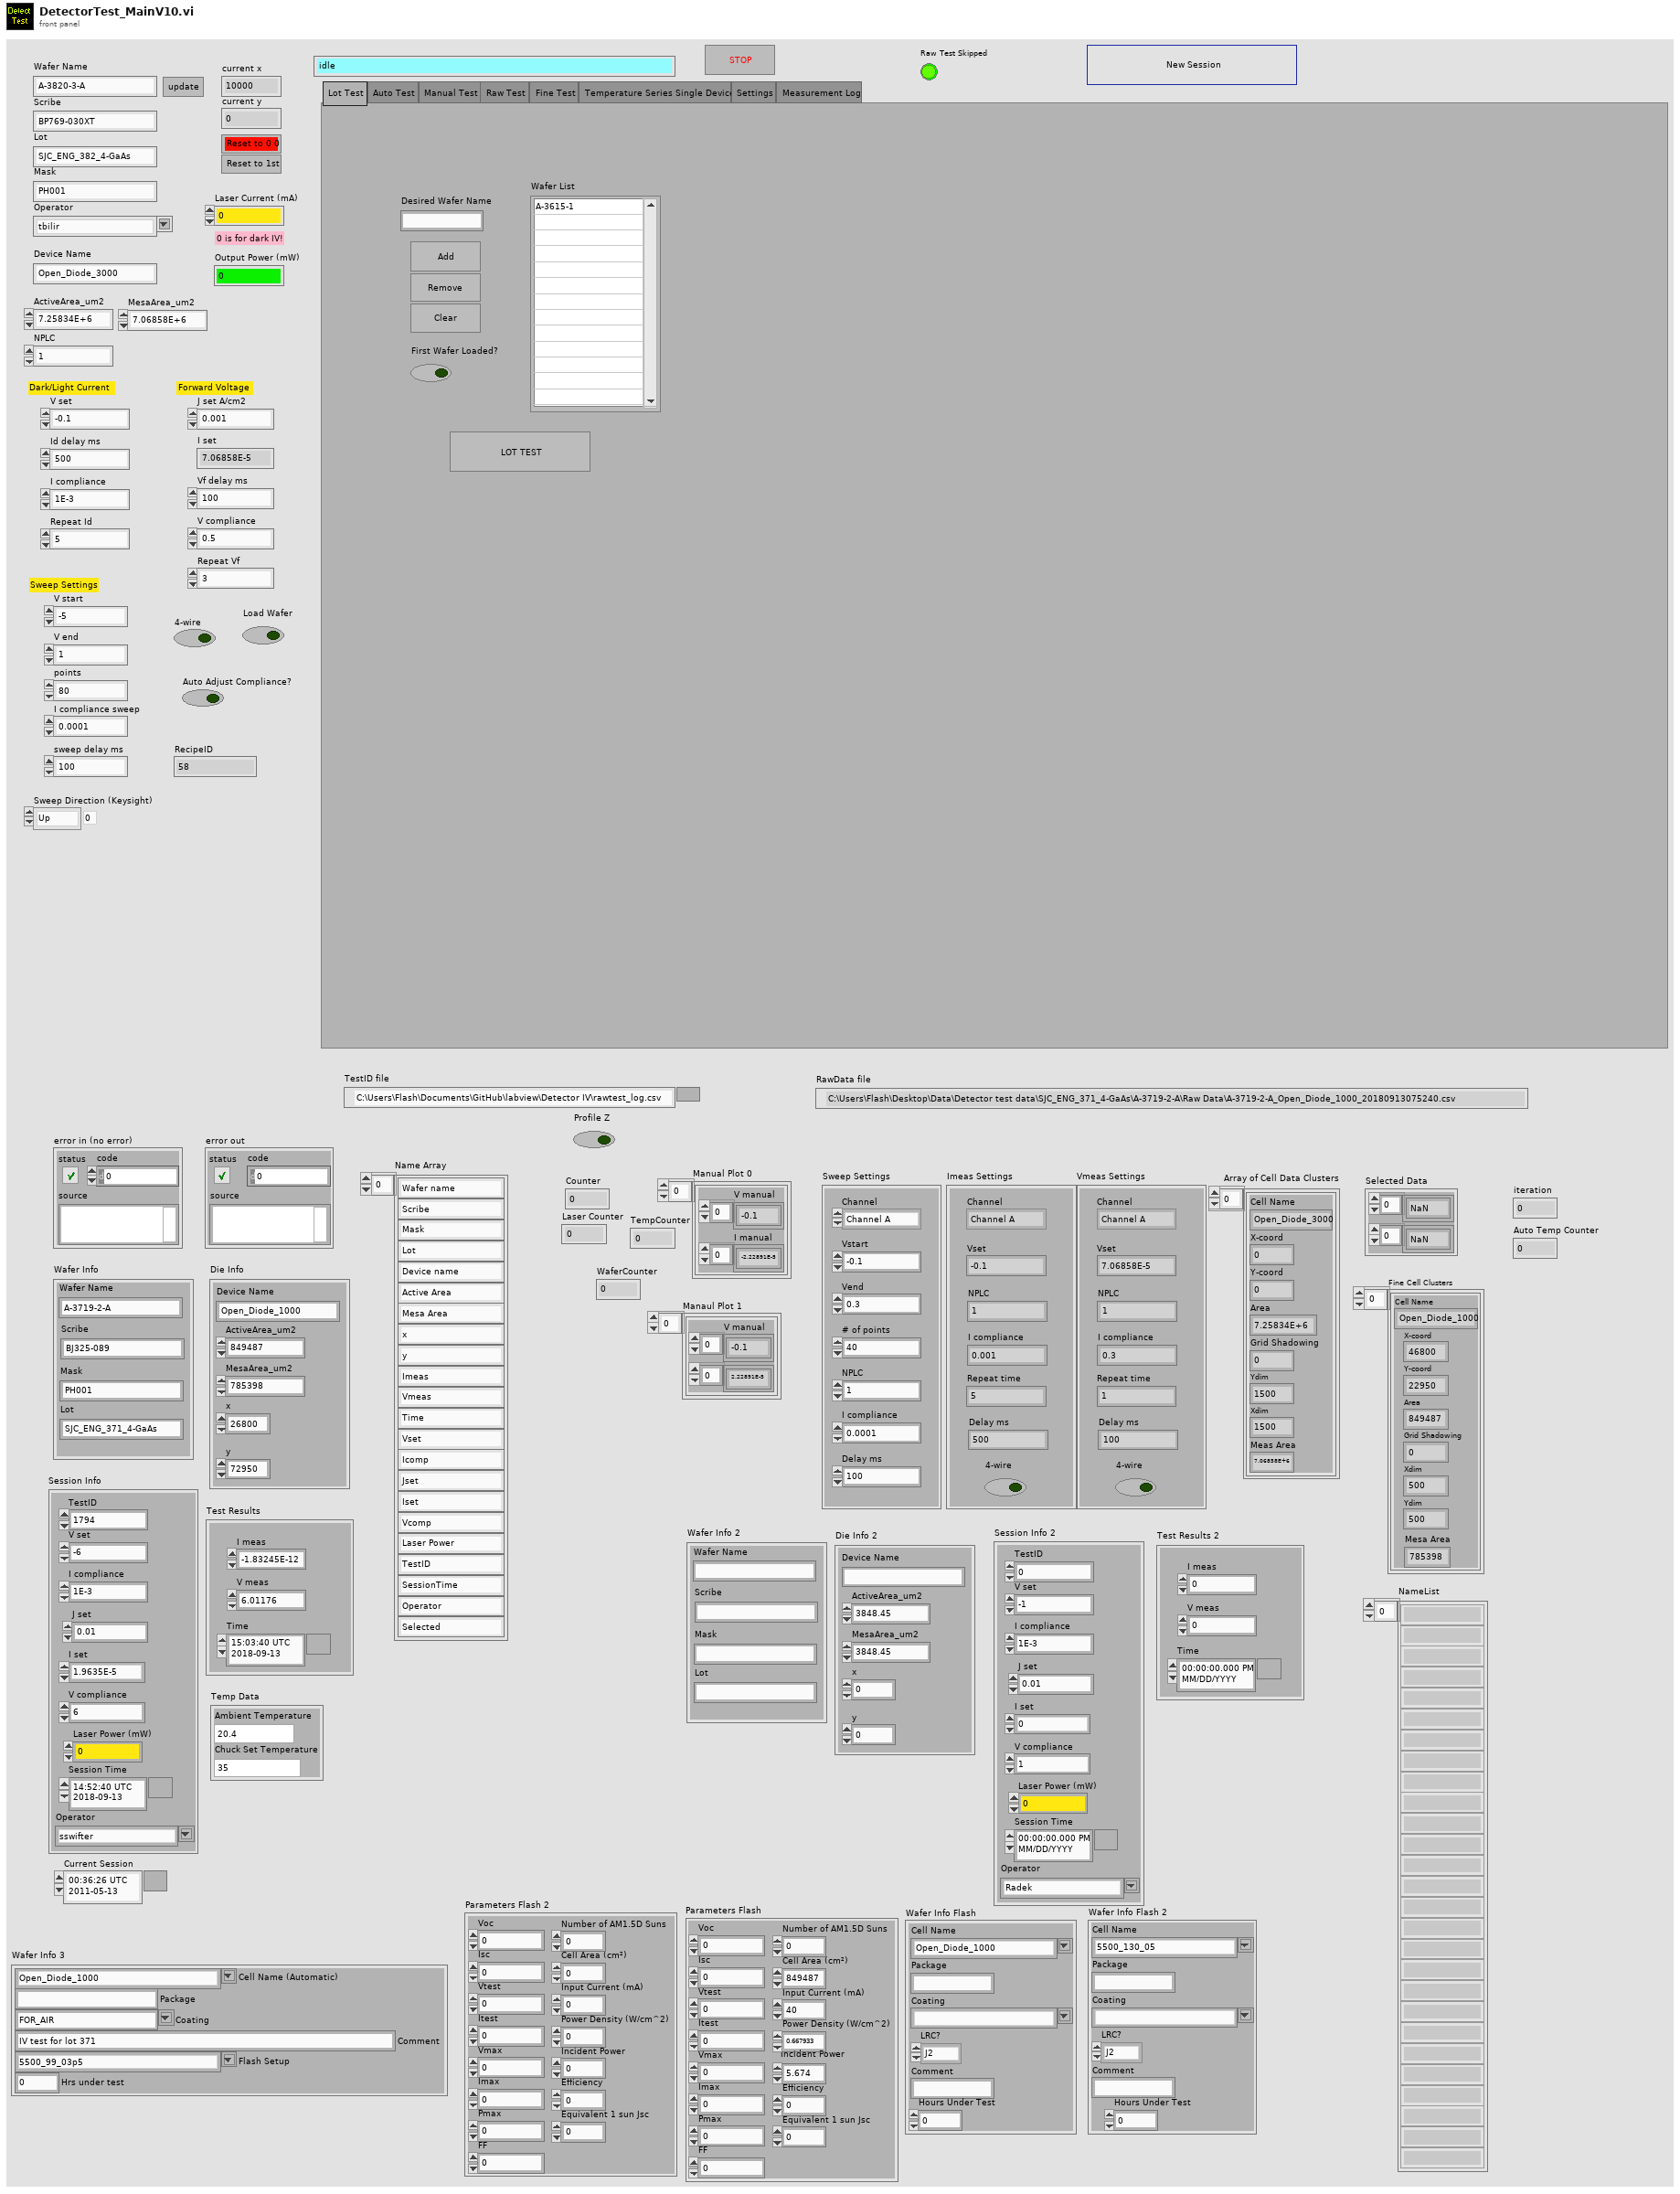
[diagram p1: front panel]
types:
  T1 = cluster{"Ambient Temperature":dbl, "Chuck Set Temperature":dbl}
  T2 = cluster{"Cell Name (Automatic)":string, "Package":string, "Coating":string, "Comment":string, "Flash Setup":string, "Hrs under test":dbl}
  T3 = cluster{"Cell Name":string, "Package":string, "Coating":string, "LRC?":enum16{"J1", "J2", "LRC"}, "Comment":string, "Hours Under Test":dbl}
  T4 = cluster{"Voc":dbl, "Isc":dbl, "FF":dbl, "Vtest":dbl, "Imax":dbl, "Vmax":dbl, "Pmax":dbl, "Itest":dbl, "Efficiency":dbl, "Incident Power":dbl, "Power Density (W/cm^2)":dbl, "Cell Area (cm²)":dbl, "Number of AM1.5D Suns":dbl, "Input Current (mA)":dbl, "Equivalent 1 sun Jsc":dbl}
  T5 = cluster{"Cell Name":string, "X-coord":dbl, "Y-coord":dbl, "Area":dbl, "Grid Shadowing":dbl, "Xdim":dbl, "Ydim":dbl, "Mesa Area":dbl}[]
  T6 = cluster{"I meas":dbl, "V meas":dbl, "Time":timestamp}
  T7 = cluster{"V set":dbl, "I compliance":dbl, "J set":dbl, "I set":dbl, "V compliance":dbl, "Laser Power (mW)":dbl, "TestID":u32, "Session Time":timestamp, "Operator":string}
  T8 = cluster{"Device Name":string, "ActiveArea_um2":dbl, "MesaArea_um2":dbl, "x":dbl, "y":dbl}
  T9 = cluster{"Wafer Name":string, "Scribe":string, "Mask":string, "Lot":string}
  T10 = cluster{"Channel":enum32{"Channel A", "Channel B"}, "Vstart":dbl, "Vend":dbl, "# of points":u16, "NPLC":dbl, "I compliance":dbl, "Delay ms":dbl}
  T11 = typedef "SMU Settings.ctl" = cluster{"Channel":enum32{"Channel A", "Channel B"}, "Vset":dbl, "NPLC":dbl, "I compliance":dbl, "Repeat time":u16, "Delay ms":dbl, "4-wire":bool}
  T12 = cluster{"Cell Name":string, "X-coord":dbl, "Y-coord":dbl, "Area":dbl, "Grid Shadowing":dbl, "Ydim":dbl, "Xdim":dbl, "Meas Area":dbl}[]
  T13 = enum32{"Lot Test", "Auto Test", "Manual Test", "Raw Test", "Fine Test", "Temperature Series Single Device", "Settings", "Measurement Log"}
  T14 = cluster{"X Values":dbl[], "Histogram: h(x)":i32[]}
  T15 = cluster{"result string":string, "time string":string, "Wafer Name":string, "Operator":string, "Test description":string, "Test Type":string}
  T16 = enum32{"Lot Test", "Auto Test", "Manual Test", "Raw Test", "Fine Test", "Temperature Series Single Device", "Settings"}
  T17 = cluster{"Cell Name":string, "X-coord":dbl, "Y-coord":dbl, "Area":dbl, "Grid Shadowing":dbl, "Ydim":dbl, "Xdim":dbl, "Meas Area":dbl}
  T18 = cluster{"Varray manual":dbl[], "Iarray manual":dbl[]}[]
  T19 = cluster{"WaferName":string, "Scribe":string, "Structure":string, "Lot":string, "Mask":string}
  T20 = cluster{"V set":dbl, "I compliance":dbl, "J set":dbl, "I set":dbl, "V compliance":dbl, "Laser Power (mW)":dbl, "TestID":u32, "Operator":string}
  T21 = cluster{"Device Name":string, "ActiveArea_um2":dbl, "MesaArea_um2":dbl}
  T22 = cluster{"Cell Name":string, "X-coord":dbl, "Y-coord":dbl, "Area":dbl, "Grid Shadowing":dbl, "Xdim":dbl, "Ydim":dbl, "Mesa Area":dbl}
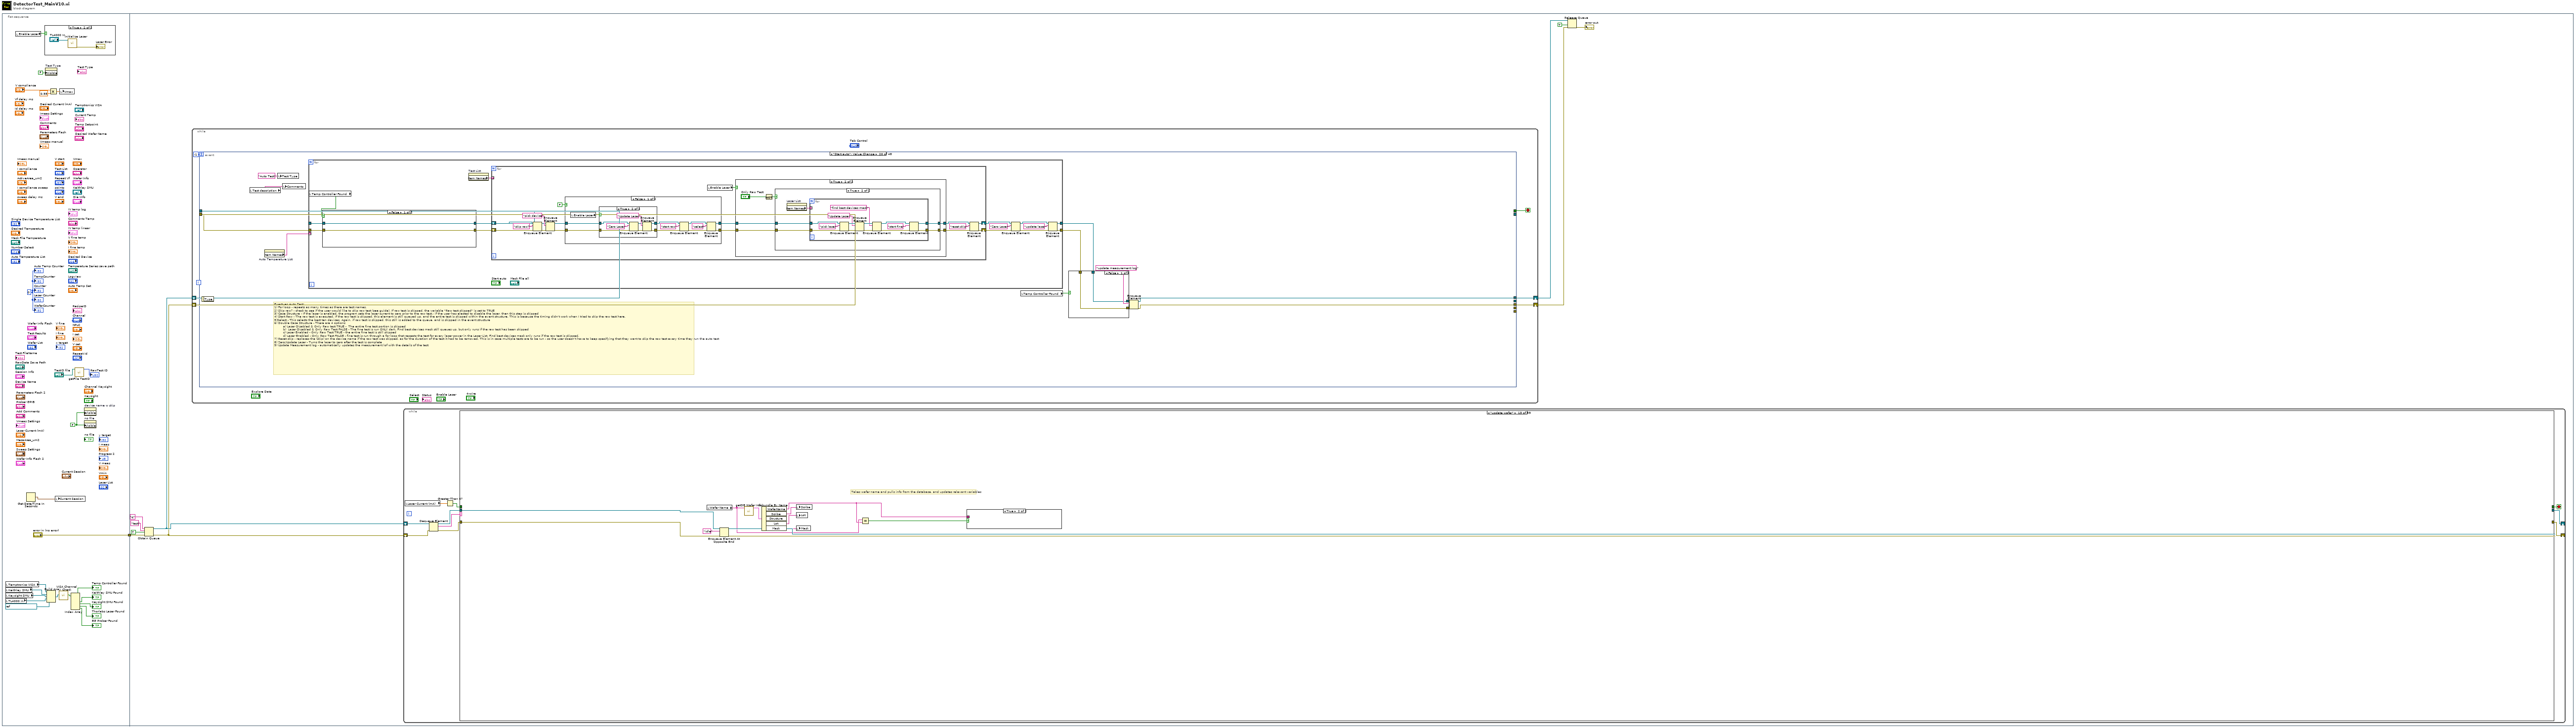
[diagram p0: block diagram]
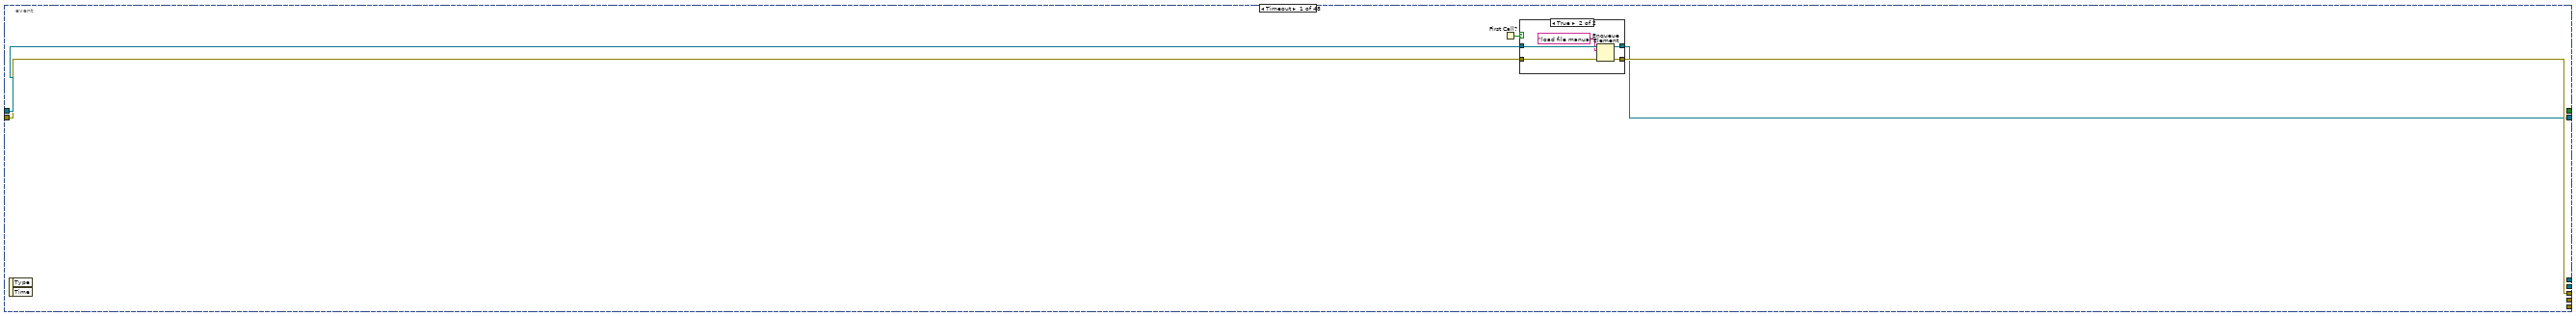
[diagram p3: hidden frame]
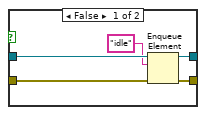
[diagram p4: hidden frame]
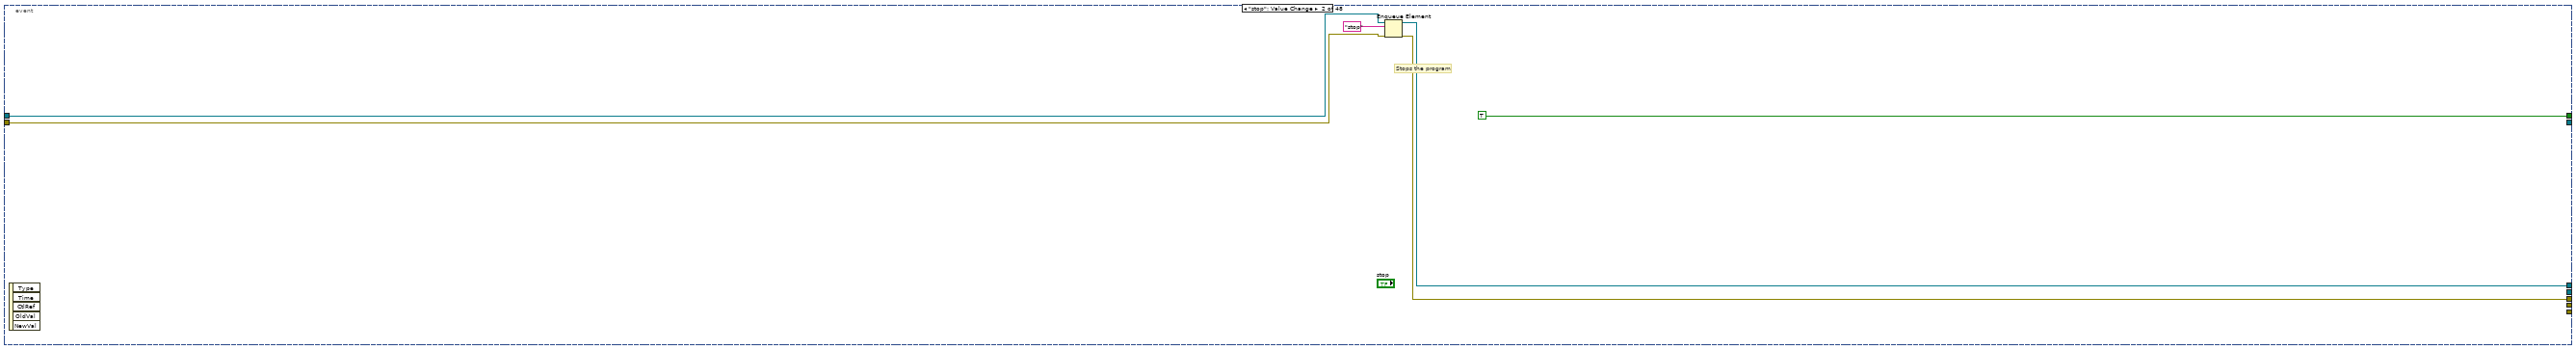
[diagram p5: hidden frame]
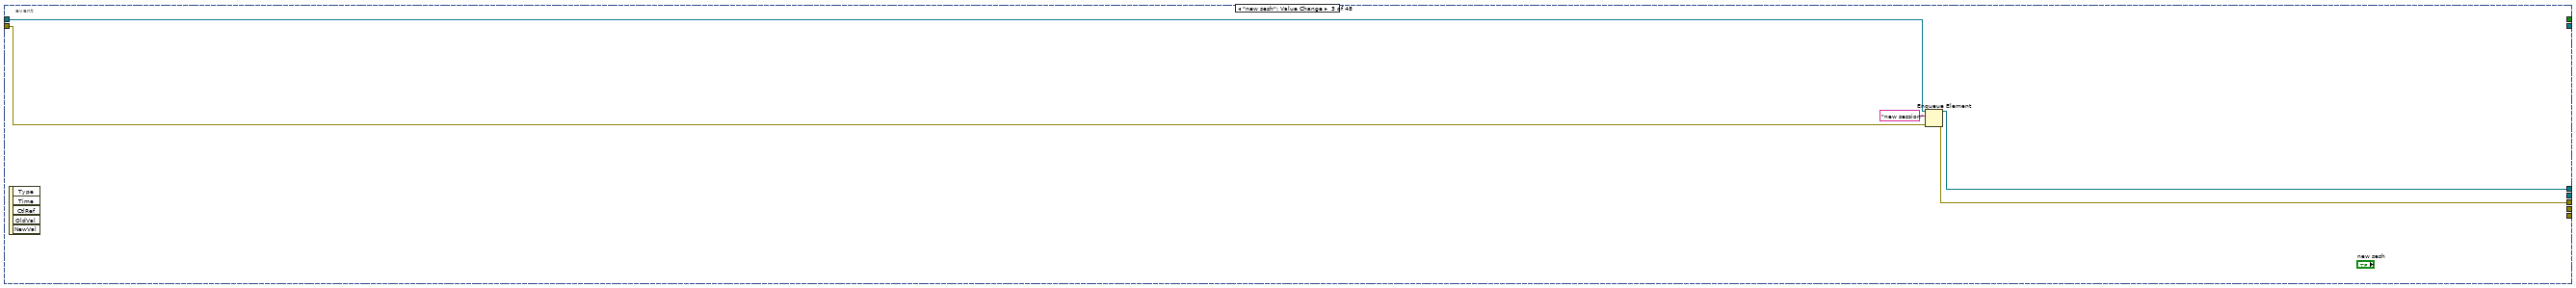
[diagram p6: hidden frame]
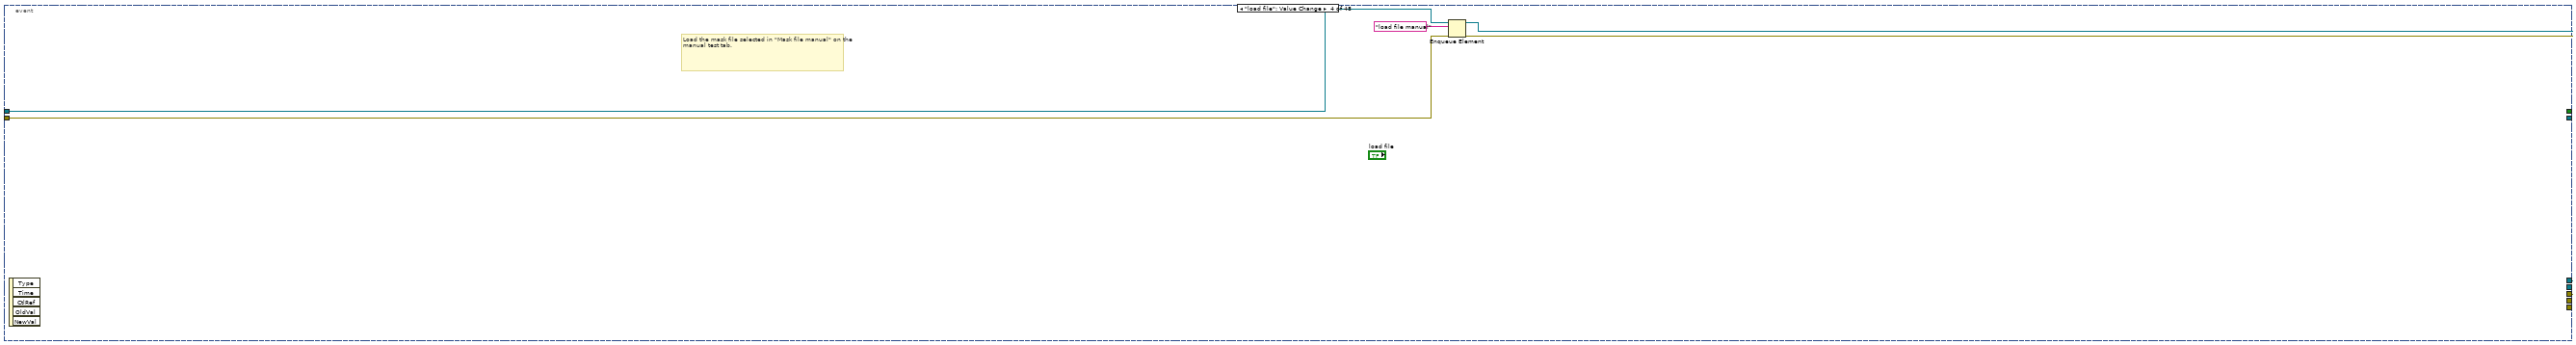
[diagram p7: hidden frame]
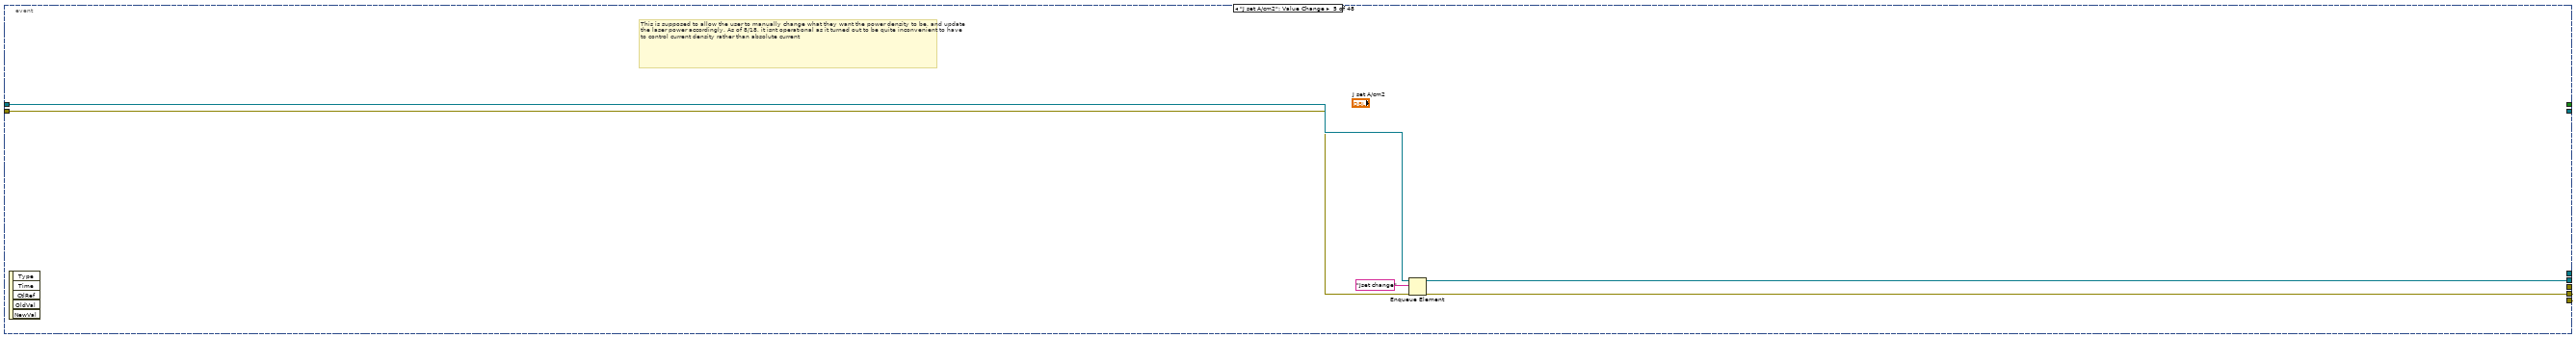
[diagram p8: hidden frame]
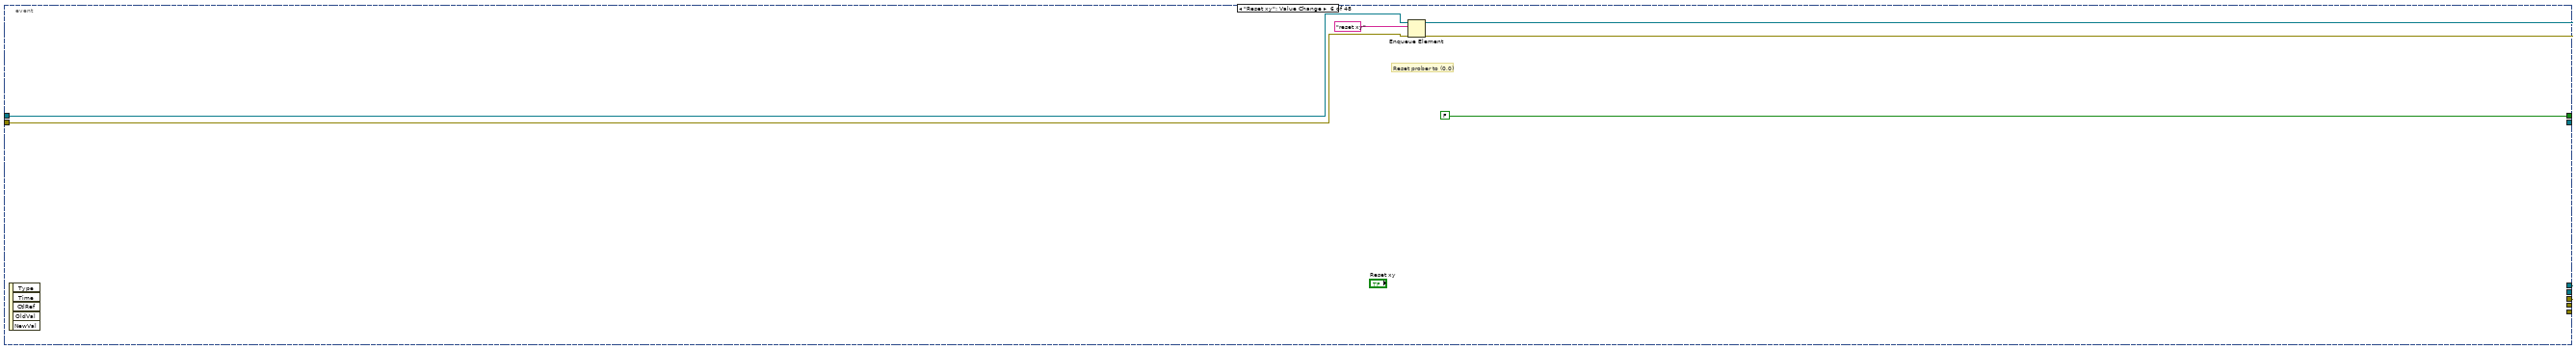
[diagram p9: hidden frame]
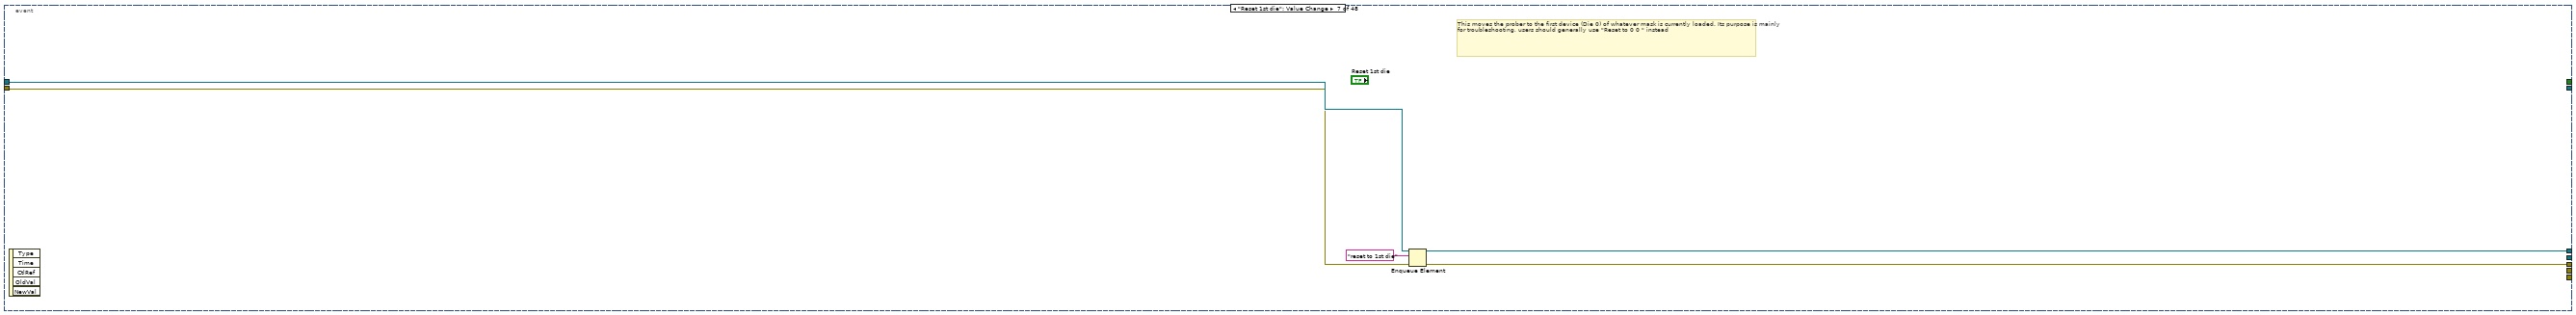
[diagram p10: hidden frame]
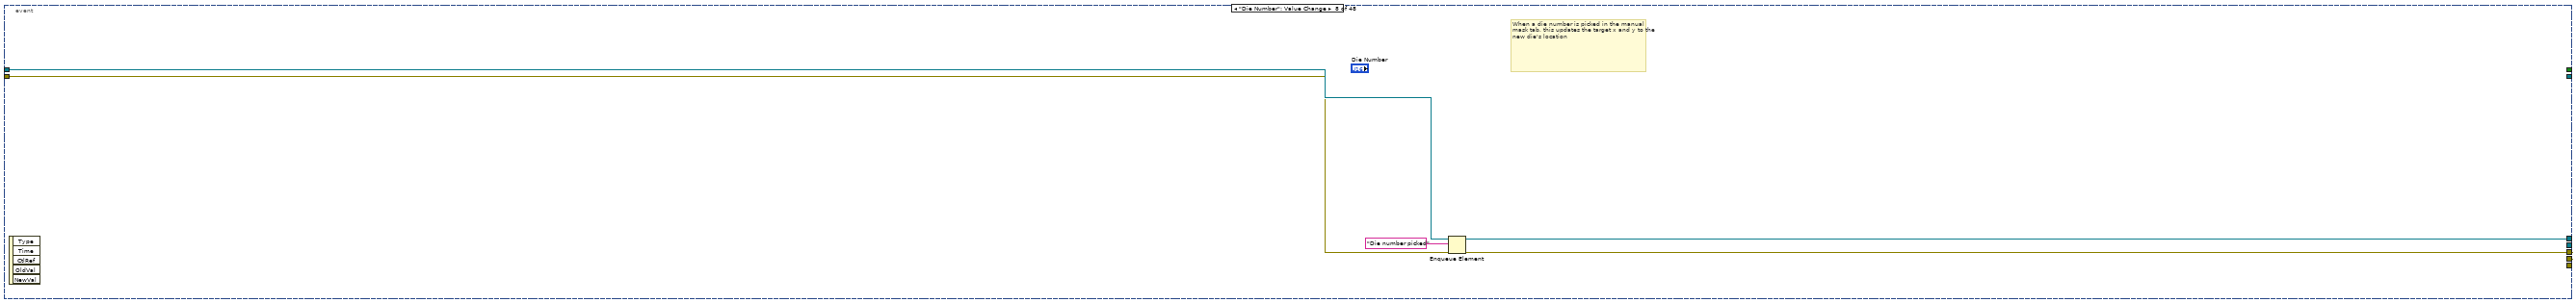
[diagram p11: hidden frame]
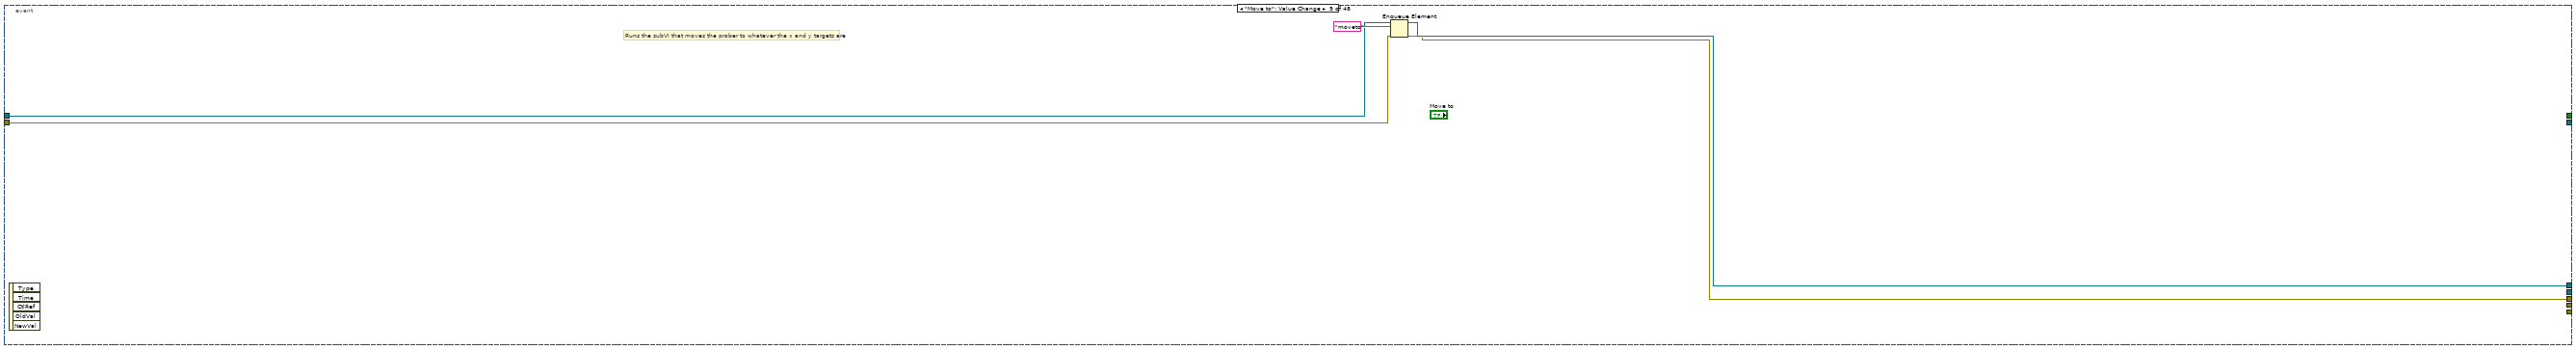
[diagram p12: hidden frame]
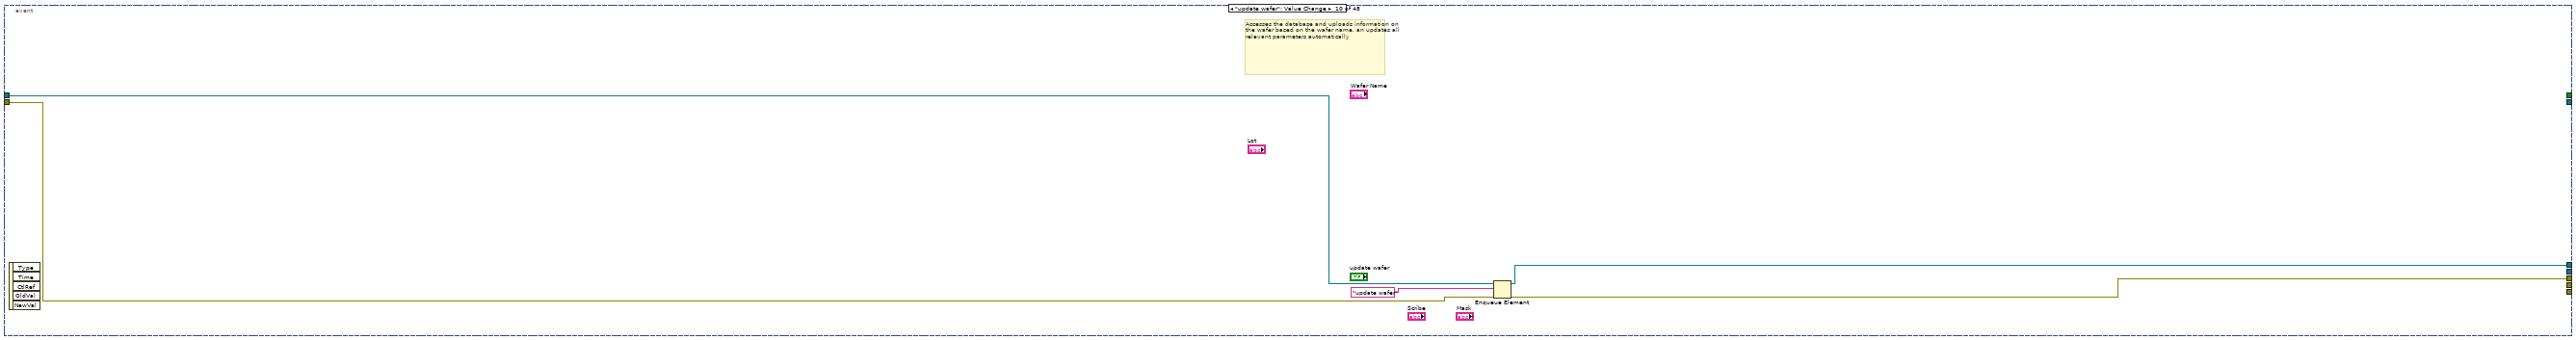
[diagram p13: hidden frame]
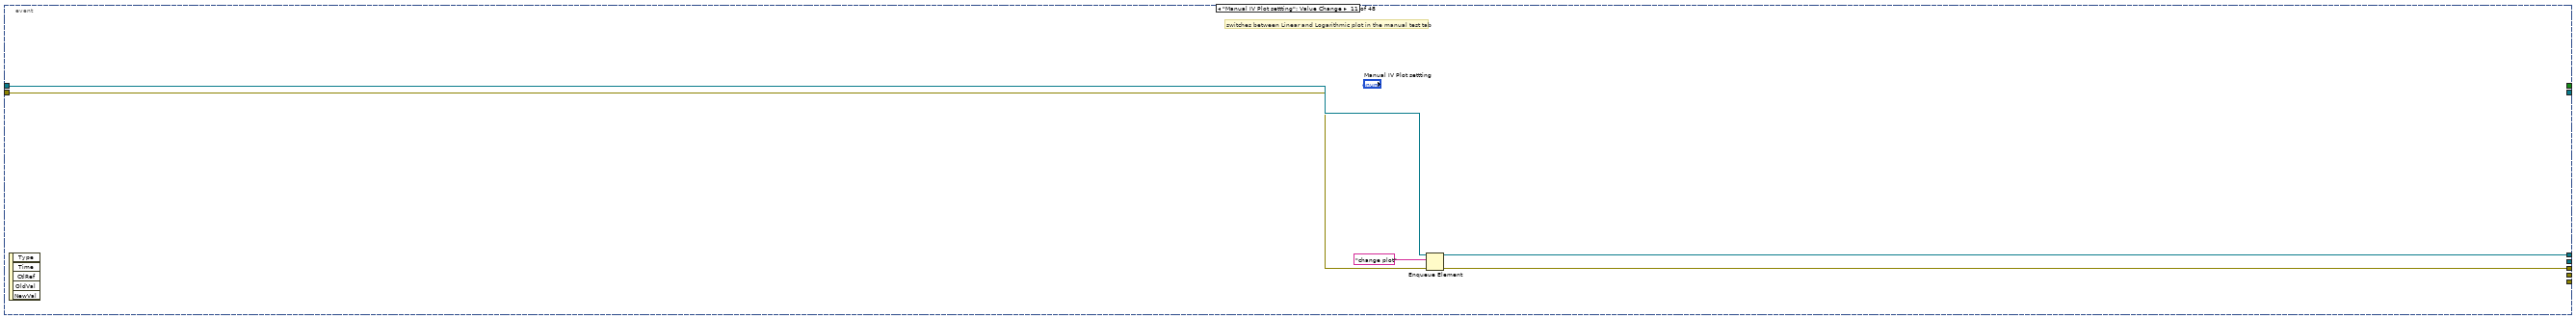
[diagram p14: hidden frame]
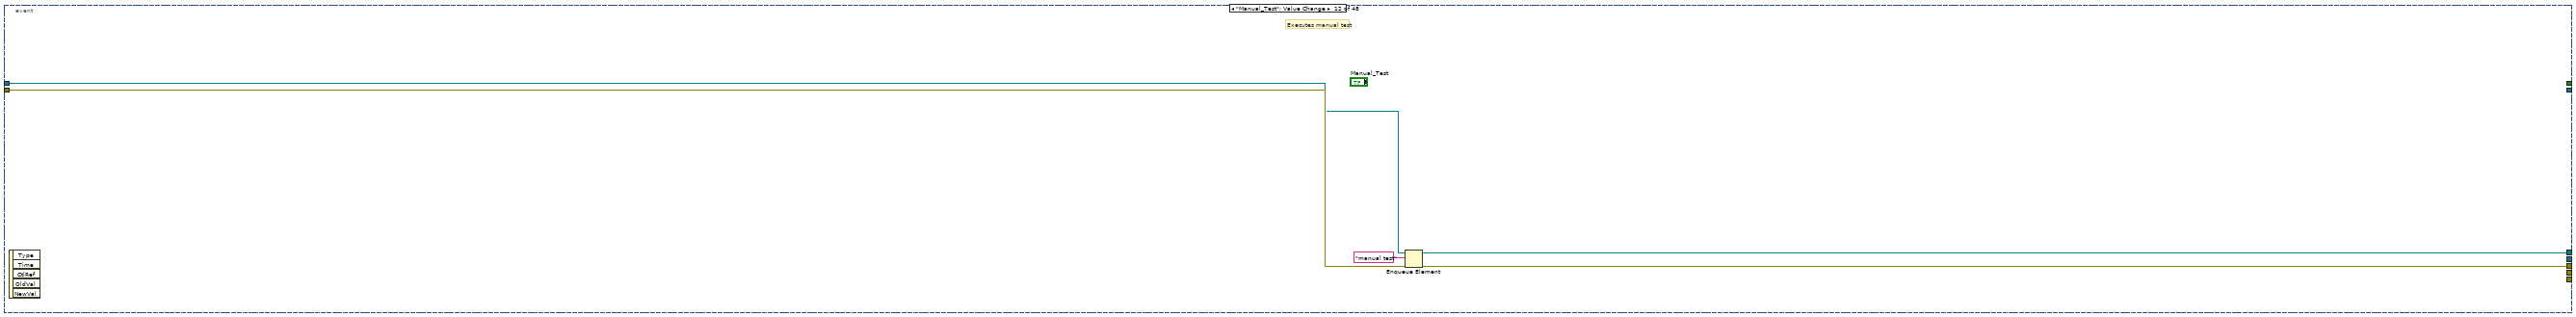
[diagram p15: hidden frame]
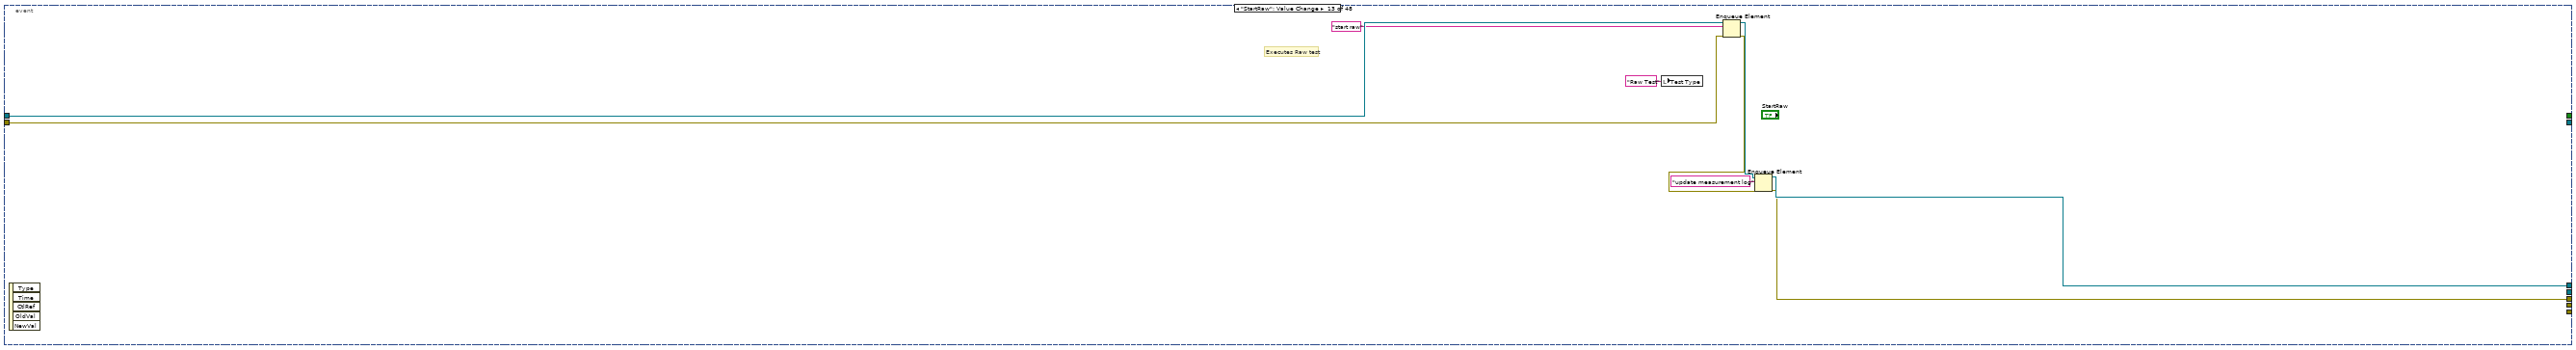
[diagram p16: hidden frame]
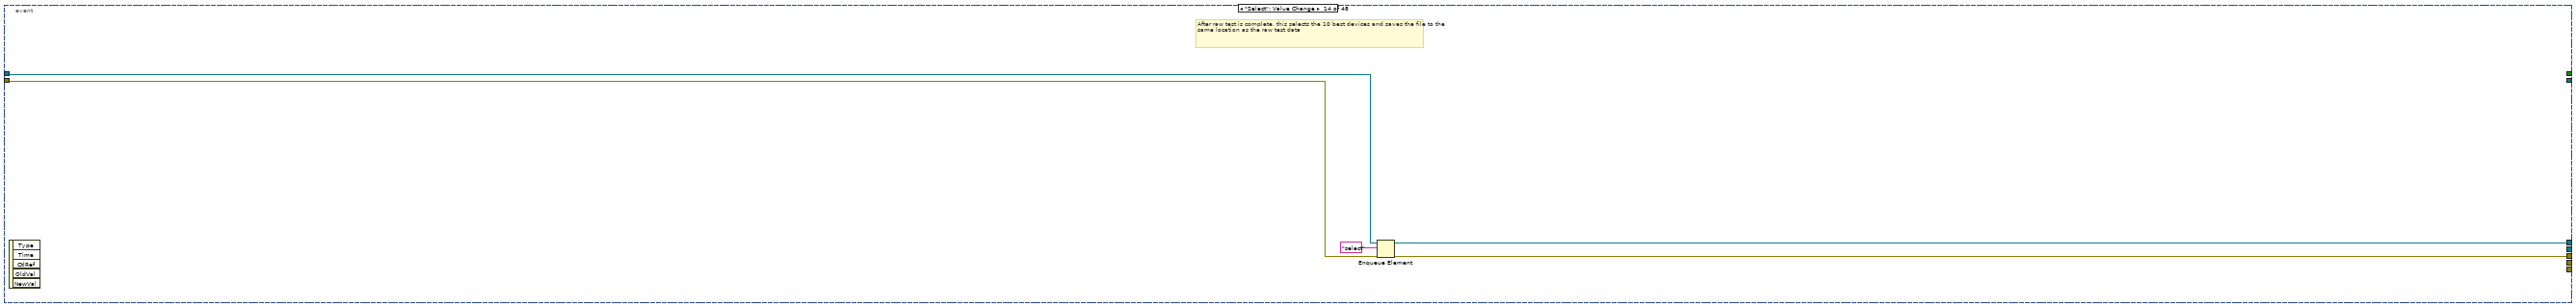
[diagram p17: hidden frame]
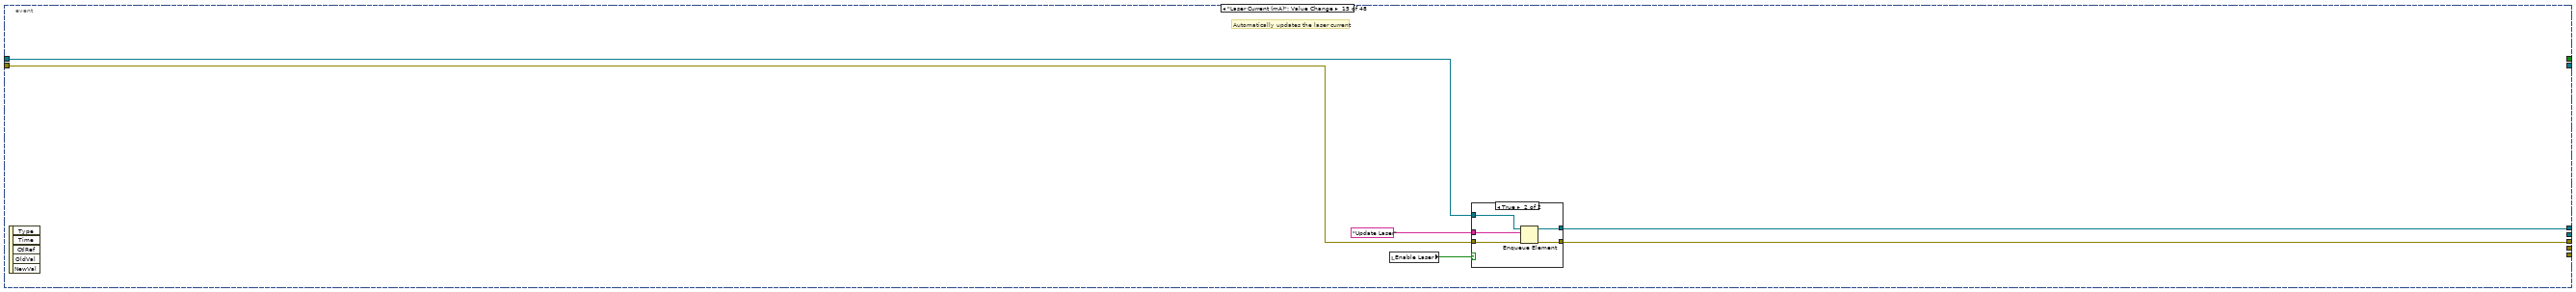
[diagram p18: hidden frame]
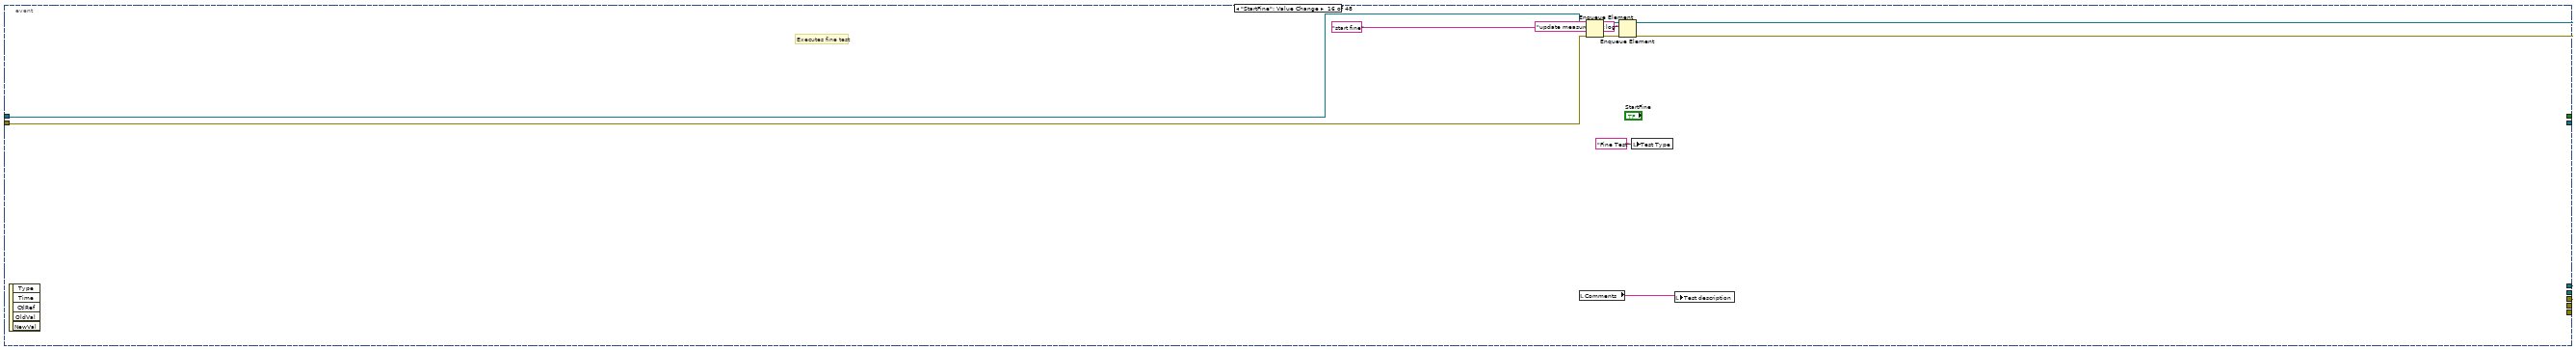
[diagram p20: hidden frame]
diagram:
  n1 = flat-sequence {
    tunnel: ["error in (no error)"] -> w1
    tunnel: w1 -> [w33]
    frame #0 {
      w18 = FALSE ("Visible")
      w16 = u32 0 ("Counter")
      n2 = local read "Temptronics VISA"() -> (w14:refnum<visa-resource-name>)
      n3 = local read "Keithley SMU"() -> (w13:refnum<visa-resource-name>)
      n4 = local read "Keysight SMU"() -> (w12:refnum<visa-resource-name>)
      n5 = local read "TL4000 In"() -> (w11:refnum<visa-resource-name>)
      n6 = local read "Enable Laser"() -> (w17:bool)
      n7 = Get Date/Time In Seconds() -> (seconds since 1Jan1904=w2:timestamp)
      n8 = case shown="True" w17 {
        frame False {
        }
        frame True {
          n9 = call "Initialize Laser.vi"("VISA Refnum in"="TL4000 In") -> ("error out"=→"Laser Error":errorcluster)  [unwired: 10 in]
        }
      }
      n10 = property on="Test Type" class="Str"("Visible"=FALSE) -> ()  [unwired: 2 in, 2 out]
      n11 = Build Array(w14, w13, w12, w11, refnum<visa-resource-name> "GPIB0::1::INSTR" ("Temptronics VISA")) -> (w9:refnum<visa-resource-name>[])
      n12 = Multiply(x="V compliance", y=0.95) -> (x*y=w20:dbl)
      n13 = local write "Current Session"(w2) -> ()
      n14 = call "VISA Channel Check.vi"("VISA Channel Array"=w9) -> ("Array"=w8:bool[])  [unwired: 10 in]
      n15 = local write "Vmax"(w20) -> ()
      n16 = Index Array(array=w8) -> (element #1=→"Temp Controller Found":bool, element #2=→"Keithley SMU Found":bool, element #3=→"Keysight SMU Found":bool, element #4=→"Thorlabs Laser Found":bool, element #5=→"EG Prober Found":bool)  [unwired: 5 in]
      n17 = call "getFile TestID.vi"("Path"="TestID file") -> ("TestID"=→"RawTest ID":u32)  [unwired: 9 in, 1 out]
      n18 = property on="device name w skip" class="Str"("Visible"=w18) -> ()  [unwired: 2 in, 2 out]
      n19 = property on="no file" class="Bool (strict)"("Visible"=w18) -> ()  [unwired: 2 in, 2 out]
      "Counter" <- w16
      "Laser Counter" <- w16
      "WaferCounter" <- w16
      "TempCounter" <- w16
      "Auto Temp Counter" <- w16
    }
    frame #1 {
      n20 = Obtain Queue(name (unnamed)="q", element data type="test" ("name (unnamed)"), create if not found? (T)=TRUE, error in (no error)=w33) -> (queue out=w35:refnum<queue>, error out=w34:errorcluster)  [unwired: 1 in, 1 out]
      n21 = while {
        shift-right: [w40] -> w36
        shift-left: w35 -> [w41]
        shift-right: [w38] -> w27
        shift-left: w34 -> [w39]
        stop <- w42 stop-if-true
        n22 = event shown="[19] \"Start auto\": Value Change" {
          selector: _ -> [_ _ _ _ _ _ _ _ _ _ _ _ _ _ _ _ _ _ _ _ _ _ _ _ _ _ _ _ _ _ _ _ _ _ _ _ _ _ _ _ _ _ _ _ _ _ _ _]
          dyn-events: _ -> [_ _ _ _ _ _ _ _ _ _ _ _ _ _ _ _ _ _ _ _ _ _ _ _ _ _ _ _ _ _ _ _ _ _ _ _ _ _ _ _ _ _ _ _ _ _ _ _]
          timeout: -1 -> [_ _ _ _ _ _ _ _ _ _ _ _ _ _ _ _ _ _ _ _ _ _ _ _ _ _ _ _ _ _ _ _ _ _ _ _ _ _ _ _ _ _ _ _ _ _ _ _]
          tunnel: [_ TRUE _ _ _ FALSE _ _ _ _ _ _ _ _ _ _ _ _ _ _ _ _ _ _ _ _ _ _ _ _ _ _ _ _ _ _ _ _ _ _ _ _ _ _ _ _ _ _] -> w42
          tunnel: w41 -> [w46 w58 w67 w73 w78 w84 w89 w94 w98 w104 w109 w112 w123 w128 w133 w151 w156 w161 w166 w179 w302 w308 w313 w319 w322 w476 w481 w486 w491 w495 w500 w506 w515 w521 w526 w531 w536 w550 w555 w559 w564 w569 w575 w579 w584 w590 w598 w602]
          tunnel: [_ w62 w65 w72 _ w83 w88 w93 w96 w102 w108 w111 w118 w126 w132 w145 w154 w159 w164 w177 w301 w306 w311 w317 w325 w474 w479 w484 w489 w493 w498 w504 w510 w519 w524 w530 w534 w545 w554 w556 w561 w568 w572 w577 w582 w588 w594 w600] -> w40
          tunnel: w39 -> [w45 w61 w66 w71 w77 w81 w87 w92 w97 w103 w107 w113 w122 w127 w131 w150 w155 w160 w165 w178 w304 w307 w312 w318 w321 w475 w480 w485 w490 w494 w501 w505 w514 w520 w525 w529 w535 w549 w553 w558 w563 w567 w574 w578 w583 w589 w597 w601]
          tunnel: [w44 w60 w64 w70 _ w82 w86 _ w95 w101 w106 w110 w117 w125 w130 w144 w153 w158 w163 w176 w303 w305 w310 w316 w324 w473 w478 w483 w488 w492 w499 w503 w509 w518 w523 w528 w533 w543 w552 w557 w562 w566 w571 w576 w581 w587 w592 w599] -> w38
          tunnel: [_ _ _ _ w76 _ _ _ _ _ _ _ _ _ _ _ _ _ _ _ _ _ _ _ _ _ _ _ _ _ _ _ _ _ _ _ _ _ _ _ _ _ _ _ _ _ _ _] -> _
          tunnel: [_ _ _ _ w75 _ _ _ _ _ _ _ _ _ _ _ _ _ _ _ _ _ _ _ _ _ _ _ _ _ _ _ _ _ _ _ _ _ _ _ _ _ _ _ _ _ _ _] -> _
          tunnel: [w43 _ _ _ _ _ _ _ _ _ _ _ _ _ _ _ _ _ _ _ _ _ _ _ _ _ _ _ _ _ _ _ _ _ _ _ _ _ _ _ _ _ _ _ _ _ _ _] -> _
          tunnel: [_ _ _ _ _ _ _ w91 _ _ _ _ _ _ _ _ _ _ _ _ _ _ _ _ _ _ _ _ _ _ _ _ _ _ _ _ _ _ _ _ _ _ _ _ _ _ _ _] -> _
          event Timeout {
            n23 = event-data() -> ()  [unwired: 1 in, 2 out]
            n24 = First Call?() -> (First Call?: T/F=w47:bool)
            n25 = case shown="True" w47 {
              tunnel: w45 -> [w50 w56]
              tunnel: w46 -> [w52 w57]
              tunnel: [w49 w55] -> w44
              tunnel: [w51 w54] -> w43
              frame False {
                n26 = Enqueue Element(queue=w52, element="idle", error in (no error)=w50) -> (queue out=w51:refnum<queue>, error out=w49:errorcluster)  [unwired: 1 in, 1 out]
              }
              frame True {
                n27 = Enqueue Element(queue=w57, element="load file manual", error in (no error)=w56) -> (queue out=w54:refnum<queue>, error out=w55:errorcluster)  [unwired: 1 in, 1 out]
              }
            }
          }
          event "stop": Value Change {
            # "Stops the program"
            n28 = event-data() -> ()  [unwired: 1 in, 5 out]
            n29 = Enqueue Element(queue=w58, element="stop", error in (no error)=w61) -> (queue out=w62:refnum<queue>, error out=w60:errorcluster)  [unwired: 1 in, 1 out]
          }
          event "new sesh": Value Change {
            n30 = event-data() -> ()  [unwired: 1 in, 5 out]
            n31 = Enqueue Element(queue=w67, element="new session", error in (no error)=w66) -> (queue out=w65:refnum<queue>, error out=w64:errorcluster)  [unwired: 1 in, 1 out]
          }
          event "load file": Value Change {
            # "Load the mask file selected in \"Mask file manual\" on the manual test tab."
            n32 = event-data() -> ()  [unwired: 1 in, 5 out]
            n33 = Enqueue Element(queue=w73, element="load file manual", error in (no error)=w71) -> (queue out=w72:refnum<queue>, error out=w70:errorcluster)  [unwired: 1 in, 1 out]
          }
          event "J set A/cm2": Value Change {
            # "This is supposed to allow the user to manually change what they want the power density to be, and update the laser power accordingly. As of 8/18, it isnt operational as it turned out to be quite inconvenient to have to control current density rather than absolute current"
            n34 = event-data() -> ()  [unwired: 1 in, 5 out]
            n35 = Enqueue Element(queue=w78, element="Jset change", error in (no error)=w77) -> (queue out=w76:refnum<queue>, error out=w75:errorcluster)  [unwired: 1 in, 1 out]
          }
          event "Reset xy": Value Change {
            # "Reset prober to (0,0)"
            n36 = event-data() -> ()  [unwired: 1 in, 5 out]
            n37 = Enqueue Element(queue=w84, element="reset xy", error in (no error)=w81) -> (queue out=w83:refnum<queue>, error out=w82:errorcluster)  [unwired: 1 in, 1 out]
          }
          event "Reset 1st die": Value Change {
            # "This moves the prober to the first device (Die 0) of whatever mask is currently loaded. Its purpose is mainly for troubleshooting, users should generally use \"Reset to 0 0 \" instead"
            n38 = event-data() -> ()  [unwired: 1 in, 5 out]
            n39 = Enqueue Element(queue=w89, element="reset to 1st die", error in (no error)=w87) -> (queue out=w88:refnum<queue>, error out=w86:errorcluster)  [unwired: 1 in, 1 out]
          }
          event "Die Number": Value Change {
            # "When a die number is picked in the manual mask tab, this updates the target x and y to the new die's location"
            n40 = event-data() -> ()  [unwired: 1 in, 5 out]
            n41 = Enqueue Element(queue=w94, element="Die number picked", error in (no error)=w92) -> (queue out=w93:refnum<queue>, error out=w91:errorcluster)  [unwired: 1 in, 1 out]
          }
          event "Move to": Value Change {
            # "Runs the subVI that moves the prober to whatever the x and y targets are"
            n42 = event-data() -> ()  [unwired: 1 in, 5 out]
            n43 = Enqueue Element(queue=w98, element="moveto", error in (no error)=w97) -> (queue out=w96:refnum<queue>, error out=w95:errorcluster)  [unwired: 1 in, 1 out]
          }
          event "update wafer": Value Change {
            # "Accesses the database and uploads information on the wafer based on the wafer name, an updates all relevant parameters automatically"
            n44 = event-data() -> ()  [unwired: 1 in, 5 out]
            n45 = Enqueue Element(queue=w104, element="update wafer", error in (no error)=w103) -> (queue out=w102:refnum<queue>, error out=w101:errorcluster)  [unwired: 1 in, 1 out]
          }
          event "Manual IV Plot settting": Value Change {
            # "switches between Linear and Logarithmic plot in the manual test tab"
            n46 = event-data() -> ()  [unwired: 1 in, 5 out]
            n47 = Enqueue Element(queue=w109, element="change plot", error in (no error)=w107) -> (queue out=w108:refnum<queue>, error out=w106:errorcluster)  [unwired: 1 in, 1 out]
          }
          event "Manual_Test": Value Change {
            # "Executes manual test"
            n48 = event-data() -> ()  [unwired: 1 in, 5 out]
            n49 = Enqueue Element(queue=w112, element="manual test", error in (no error)=w113) -> (queue out=w111:refnum<queue>, error out=w110:errorcluster)  [unwired: 1 in, 1 out]
          }
          event "StartRaw": Value Change {
            # "Executes Raw test"
            n50 = event-data() -> ()  [unwired: 1 in, 5 out]
            n51 = local write "Test Type"("Raw Test" ("Test Type")) -> ()
            n52 = Enqueue Element(queue=w123, element="start raw", error in (no error)=w122) -> (queue out=w119:refnum<queue>, error out=w116:errorcluster)  [unwired: 1 in, 1 out]
            n53 = Enqueue Element(queue=w119, element="update measurement log", error in (no error)=w116) -> (queue out=w118:refnum<queue>, error out=w117:errorcluster)  [unwired: 1 in, 1 out]
          }
          event "Select": Value Change {
            # "After raw test is complete, this selects the 10 best devices and saves the file to the same location as the raw test data"
            n54 = event-data() -> ()  [unwired: 1 in, 5 out]
            n55 = Enqueue Element(queue=w128, element="select", error in (no error)=w127) -> (queue out=w126:refnum<queue>, error out=w125:errorcluster)  [unwired: 1 in, 1 out]
          }
          event "Laser Current (mA)": Value Change {
            # "Automatically updates the laser current"
            n56 = event-data() -> ()  [unwired: 1 in, 5 out]
            n57 = local read "Enable Laser"() -> (w129:bool)
            n58 = case shown="True" w129 {
              tunnel: "Update Laser" ("element") -> [_ w141]
              tunnel: w133 -> [w136 w140]
              tunnel: [w136 w139] -> w132
              tunnel: w131 -> [w135 w138]
              tunnel: [w135 w137] -> w130
              frame False {
              }
              frame True {
                n59 = Enqueue Element(queue=w140, element=w141, error in (no error)=w138) -> (queue out=w139:refnum<queue>, error out=w137:errorcluster)  [unwired: 1 in, 1 out]
              }
            }
          }
          event "StartFine": Value Change {
            # "Executes fine test"
            n60 = event-data() -> ()  [unwired: 1 in, 5 out]
            n61 = local read "Comments"() -> (w142:string)
            n62 = Enqueue Element(queue=w151, element="start fine", error in (no error)=w150) -> (queue out=w147:refnum<queue>, error out=w146:errorcluster)  [unwired: 1 in, 1 out]
            n63 = Enqueue Element(queue=w147, element="update measurement log", error in (no error)=w146) -> (queue out=w145:refnum<queue>, error out=w144:errorcluster)  [unwired: 1 in, 1 out]
            n64 = local write "Test Type"("Fine Test" ("Test Type")) -> ()
            n65 = local write "Test description"(w142) -> ()
          }
          event "Mask File Raw": Value Change {
            # "When raw mask is updated, it asks if you want to update the manual test mask as well"
            n66 = event-data() -> ()  [unwired: 1 in, 5 out]
            n67 = Enqueue Element(queue=w156, element="raw mask updated", error in (no error)=w155) -> (queue out=w154:refnum<queue>, error out=w153:errorcluster)  [unwired: 1 in, 1 out]
          }
          event "Mask File Manual": Value Change {
            # "When manual mask is updated, it asks if the user would want to update the raw test as well"
            n68 = event-data() -> ()  [unwired: 1 in, 5 out]
            n69 = Enqueue Element(queue=w161, element="mask manual update", error in (no error)=w160) -> (queue out=w159:refnum<queue>, error out=w158:errorcluster)  [unwired: 1 in, 1 out]
          }
          event "Load raw": Value Change {
            # "Gives the user the option to pick a raw data file, and then displays that on the graphical display on the raw test tab"
            n70 = event-data() -> ()  [unwired: 1 in, 5 out]
            n71 = Enqueue Element(queue=w166, element="load raw data", error in (no error)=w165) -> (queue out=w164:refnum<queue>, error out=w163:errorcluster)  [unwired: 1 in, 1 out]
          }
          event "Start auto": Value Change {
            # "Exectues Auto Test:\n1) For loop - repeats as many times as there are test names.\n2) Skip raw? - check to see if the user would like to skip raw test (see guide). If raw test is skipped, the variable \"Raw test skipped\" is set to TRUE\n3) Case Structure - If the laser is enabled, the program sets the laser current to zero prior to the raw test.; if the user has elected to disable the laser, then this step is skipped\n4) Start Raw - The raw test is executed. If the raw test is skipped, this element is still queued up, and the entire test is skipped within the event structure. This is because the timing didn't work when I tried to skip the raw test here.\n5)Select - This selects the best ten devices. Again, if raw test is skipped, this still is added to the queue, and is skipped in the event structure\n6) Double Case Structure - There are 4 options\n         a) Laser Disabled & Only Raw test TRUE -  The entire fine test portion is skipped\n         b)  Laser Disabled & Only Raw Test FALSE - The fine test is run ONLY dark. Find best devices mask still queues up, but only runs if the raw test has been skipped\n         c) Laser Enabled - Only Raw Test TRUE - the entire fine test is still skipped\n         d) Laser Enabled - Only Raw Test FALSE - fine test is run through a for loop that repeats the test for every laser power in the Laser List. Find best devices mask only runs if the raw test is skipped.\n7) Reset skip - replaces the (skip) on the device name if the raw test was skipped, as for the duration of the test it had to be removed. This is in case multiple tests are to be run - so the user doesn't have to keep specifying that they want to skip the raw test every time they run the auto test\n8) Zero/Update Laser - Turns the laser to zero after the test is complete\n9) Update Measurement log - automatically updates the measurement lof with the details of the test"
            n72 = event-data() -> ()  [unwired: 1 in, 1 out]
            n73 = local read "Test description"() -> (w174:string)
            n74 = property on="Auto Temperature List" class="LstBox (strict)"() -> ("Item Names"=w172:string[])  [unwired: 2 in, 2 out]
            n75 = local write "Test Type"("Auto Test" ("Test Type")) -> ()
            n76 = local write "Comments"(w174) -> ()
            n77 = for {
              tunnel: w179 -> [w194]
              tunnel: w178 -> [w193]
              tunnel: [w197] -> w171
              tunnel: [w196] -> w169
              tunnel: w172 -> [_] mode=indexing
              n78 = local read "Temp Controller Found"() -> (w190:bool)
              n79 = case shown="False" w190 {
                tunnel: w194 -> [w205 w216]
                tunnel: w193 -> [w204 w215]
                tunnel: [w205 w214] -> w192
                tunnel: [w204 w213] -> w191
                frame False {
                }
                frame True {
                  n80 = Enqueue Element(queue=w216, element="select temperature", error in (no error)=w215) -> (queue out=w210:refnum<queue>, error out=w208:errorcluster)  [unwired: 1 in, 1 out]
                  n81 = Enqueue Element(queue=w210, element="update temperature", error in (no error)=w208) -> (queue out=w209:refnum<queue>, error out=w207:errorcluster)  [unwired: 1 in, 1 out]
                  n82 = Enqueue Element(queue=w209, element="wait for temperature", error in (no error)=w207) -> (queue out=w214:refnum<queue>, error out=w213:errorcluster)  [unwired: 1 in, 1 out]
                }
              }
              n83 = property on="Test List" class="LstBox (strict)"() -> ("Item Names"=w203:string[])  [unwired: 2 in, 2 out]
              n84 = for {
                shift-right: [w217] -> w200
                shift-left: w191 -> [w225]
                shift-right: [w220] -> w201
                shift-left: w192 -> [w226]
                tunnel: w203 -> [_] mode=indexing
                n85 = Enqueue Element(queue=w226, element="skip raw?", error in (no error)=w225) -> (queue out=w224:refnum<queue>, error out=w223:errorcluster)  [unwired: 1 in, 1 out]
                n86 = Enqueue Element(queue=w224, element="pick device", error in (no error)=w223) -> (queue out=w232:refnum<queue>, error out=w231:errorcluster)  [unwired: 1 in, 1 out]
                n87 = case shown="False" FALSE {
                  tunnel: w232 -> [w285 w298]
                  tunnel: w231 -> [w284 w299]
                  tunnel: [w282 w298] -> w230
                  tunnel: [w281 w299] -> w229
                  frame False {
                    n88 = local read "Enable Laser"() -> (w283:bool)
                    n89 = case shown="True" w283 {
                      tunnel: [w289 w297] -> w287
                      tunnel: [w288 w296] -> w286
                      tunnel: w285 -> [w289 w294]
                      tunnel: w284 -> [w288 w292]
                      frame False {
                      }
                      frame True {
                        n90 = Enqueue Element(queue=w294, element="Zero Laser", error in (no error)=w292) -> (queue out=w293:refnum<queue>, error out=w291:errorcluster)  [unwired: 1 in, 1 out]
                        n91 = Enqueue Element(queue=w293, element="Update Laser", error in (no error)=w291) -> (queue out=w297:refnum<queue>, error out=w296:errorcluster)  [unwired: 1 in, 1 out]
                      }
                    }
                    n92 = Enqueue Element(queue=w287, element="start raw", error in (no error)=w286) -> (queue out=w278:refnum<queue>, error out=w277:errorcluster)  [unwired: 1 in, 1 out]
                    n93 = Enqueue Element(queue=w278, element="select", error in (no error)=w277) -> (queue out=w282:refnum<queue>, error out=w281:errorcluster)  [unwired: 1 in, 1 out]
                  }
                  frame True {
                  }
                }
                n94 = local read "Enable Laser"() -> (w227:bool)
                n95 = case shown="True" w227 {
                  tunnel: [w239 w255] -> w221
                  tunnel: [w238 w254] -> w218
                  tunnel: w230 -> [w237 w253]
                  tunnel: w229 -> [w236 w252]
                  frame False {
                    n96 = local read "Only Raw Test"() -> (w234:bool)
                    n97 = Not(x=w234) -> (.not. x?=w235:bool)
                    n98 = case shown="False" w235 {
                      tunnel: [w241 w249] -> w239
                      tunnel: [w240 w248] -> w238
                      tunnel: w237 -> [w241 w247]
                      tunnel: w236 -> [w240 w245]
                      frame False {
                      }
                      frame True {
                        n99 = Enqueue Element(queue=w247, element="find best devices mask", error in (no error)=w245) -> (queue out=w246:refnum<queue>, error out=w244:errorcluster)  [unwired: 1 in, 1 out]
                        n100 = Enqueue Element(queue=w246, element="start fine", error in (no error)=w244) -> (queue out=w249:refnum<queue>, error out=w248:errorcluster)  [unwired: 1 in, 1 out]
                      }
                    }
                  }
                  frame True {
                    n101 = Not(x="Only Raw Test") -> (.not. x?=w250:bool)
                    n102 = case shown="True" w250 {
                      tunnel: [w257 w262] -> w255
                      tunnel: [w256 w261] -> w254
                      tunnel: w253 -> [w257 w260]
                      tunnel: w252 -> [w256 w259]
                      frame False {
                      }
                      frame True {
                        n103 = property on="Laser List" class="LstBox (strict)"() -> ("Item Names"=w258:string[])  [unwired: 2 in, 2 out]
                        n104 = for {
                          tunnel: [w276] -> w262
                          tunnel: [w275] -> w261
                          tunnel: w260 -> [w271]
                          tunnel: w259 -> [w274]
                          tunnel: w258 -> [_] mode=indexing
                          n105 = Enqueue Element(queue=w271, element="pick laser", error in (no error)=w274) -> (queue out=w270:refnum<queue>, error out=w272:errorcluster)  [unwired: 1 in, 1 out]
                          n106 = Enqueue Element(queue=w270, element="Update Laser", error in (no error)=w272) -> (queue out=w265:refnum<queue>, error out=w268:errorcluster)  [unwired: 1 in, 1 out]
                          n107 = Enqueue Element(queue=w265, element="find best devices mask", error in (no error)=w268) -> (queue out=w266:refnum<queue>, error out=w267:errorcluster)  [unwired: 1 in, 1 out]
                          n108 = Enqueue Element(queue=w266, element="start fine", error in (no error)=w267) -> (queue out=w276:refnum<queue>, error out=w275:errorcluster)  [unwired: 1 in, 1 out]
                        }
                      }
                    }
                  }
                }
                n109 = Enqueue Element(queue=w221, element="reset skip", error in (no error)=w218) -> (queue out=w220:refnum<queue>, error out=w217:errorcluster)  [unwired: 1 in, 1 out]
              }
              n110 = Enqueue Element(queue=w201, element="Zero Laser", error in (no error)=w200) -> (queue out=w199:refnum<queue>, error out=w198:errorcluster)  [unwired: 1 in, 1 out]
              n111 = Enqueue Element(queue=w199, element="update laser", error in (no error)=w198) -> (queue out=w197:refnum<queue>, error out=w196:errorcluster)  [unwired: 1 in, 1 out]
            }
            n112 = local read "Temp Controller Found"() -> (w167:bool)
            n113 = case shown="False" w167 {
              tunnel: w171 -> [w181 w189]
              tunnel: [w181 w187] -> w170
              tunnel: w169 -> [w180 w186]
              tunnel: [w180 w184] -> w168
              frame False {
              }
              frame True {
                n114 = Enqueue Element(queue=w189, element="temp to 25", error in (no error)=w186) -> (queue out=w188:refnum<queue>, error out=w185:errorcluster)  [unwired: 1 in, 1 out]
                n115 = Enqueue Element(queue=w188, element="update temperature", error in (no error)=w185) -> (queue out=w187:refnum<queue>, error out=w184:errorcluster)  [unwired: 1 in, 1 out]
              }
            }
            n116 = Enqueue Element(queue=w170, element="update measurement log", error in (no error)=w168) -> (queue out=w177:refnum<queue>, error out=w176:errorcluster)  [unwired: 1 in, 1 out]
          }
          event "Generate Report": Value Change {
            n117 = event-data() -> ()  [unwired: 1 in, 5 out]
            n118 = Enqueue Element(queue=w302, element="generate prelim report", error in (no error)=w304) -> (queue out=w301:refnum<queue>, error out=w303:errorcluster)  [unwired: 1 in, 1 out]
          }
          event "Add to Temp Auto": Value Change {
            n119 = event-data() -> ()  [unwired: 1 in, 5 out]
            n120 = Enqueue Element(queue=w308, element="add temp auto", error in (no error)=w307) -> (queue out=w306:refnum<queue>, error out=w305:errorcluster)  [unwired: 1 in, 1 out]
          }
          event "Remove from Temp Auto": Value Change {
            n121 = event-data() -> ()  [unwired: 1 in, 5 out]
            n122 = Enqueue Element(queue=w313, element="remove temp auto", error in (no error)=w312) -> (queue out=w311:refnum<queue>, error out=w310:errorcluster)  [unwired: 1 in, 1 out]
          }
          event "Clear temp list Auto": Value Change {
            n123 = event-data() -> ()  [unwired: 1 in, 5 out]
            n124 = Enqueue Element(queue=w319, element="clear temp auto", error in (no error)=w318) -> (queue out=w317:refnum<queue>, error out=w316:errorcluster)  [unwired: 1 in, 1 out]
          }
          event "begin lot test": Value Change {
            n125 = event-data() -> ()  [unwired: 1 in, 5 out]
            n126 = local write "Test Type"("Lot Test" ("Test Type")) -> ()
            n127 = property on="Wafer List" class="LstBox (strict)"() -> ("Item Names"=w323:string[])  [unwired: 2 in, 2 out]
            n128 = for {
              tunnel: w323 -> [_] mode=indexing
              shift-right: [w333] -> w325
              shift-left: w322 -> [w352]
              shift-right: [w332] -> w324
              shift-left: w321 -> [w351]
              i -> [w350]
              n129 = Equal?(x=w350, y=0) -> (x = y?=w348:bool)
              n130 = And(x="First Wafer Loaded?", y=w348) -> (x .and. y?=w346:bool)
              n131 = case shown="False" w346 {
                tunnel: w352 -> [w459 w471]
                tunnel: w351 -> [w458 w470]
                tunnel: [w457 w471] -> w345
                tunnel: [w456 w470] -> w340
                frame False {
                  n132 = Enqueue Element(queue=w459, element="load wafer", error in (no error)=w458) -> (queue out=w464:refnum<queue>, error out=w463:errorcluster)  [unwired: 1 in, 1 out]
                  n133 = Enqueue Element(queue=w464, element="wait", error in (no error)=w463) -> (queue out=w462:refnum<queue>, error out=w461:errorcluster)  [unwired: 1 in, 1 out]
                  n134 = Enqueue Element(queue=w462, element="profile z", error in (no error)=w461) -> (queue out=w467:refnum<queue>, error out=w466:errorcluster)  [unwired: 1 in, 1 out]
                  n135 = Enqueue Element(queue=w467, element="auto align", error in (no error)=w466) -> (queue out=w457:refnum<queue>, error out=w456:errorcluster)  [unwired: 1 in, 1 out]
                }
                frame True {
                }
              }
              n136 = Enqueue Element(queue=w345, element="desired wafer to current wafer", error in (no error)=w340) -> (queue out=w344:refnum<queue>, error out=w341:errorcluster)  [unwired: 1 in, 1 out]
              n137 = Enqueue Element(queue=w344, element="update wafer", error in (no error)=w341) -> (queue out=w343:refnum<queue>, error out=w342:errorcluster)  [unwired: 1 in, 1 out]
              n138 = property on="Auto Temperature List" class="LstBox (strict)"() -> ("Item Names"=w326:string[])  [unwired: 2 in, 2 out]
              n139 = for {
                tunnel: [w365] -> w336
                tunnel: [w364] -> w329
                tunnel: w343 -> [w363]
                tunnel: w342 -> [w362]
                tunnel: w326 -> [_] mode=indexing
                n140 = Enqueue Element(queue=w363, element="select temperature", error in (no error)=w362) -> (queue out=w361:refnum<queue>, error out=w360:errorcluster)  [unwired: 1 in, 1 out]
                n141 = Enqueue Element(queue=w361, element="update temperature", error in (no error)=w360) -> (queue out=w359:refnum<queue>, error out=w358:errorcluster)  [unwired: 1 in, 1 out]
                n142 = property on="Test List" class="LstBox (strict)"() -> ("Item Names"=w371:string[])  [unwired: 2 in, 2 out]
                n143 = Enqueue Element(queue=w359, element="wait for temperature", error in (no error)=w358) -> (queue out=w357:refnum<queue>, error out=w356:errorcluster)  [unwired: 1 in, 1 out]
                n144 = for {
                  shift-right: [w376] -> w366
                  shift-left: w356 -> [w381]
                  shift-right: [w377] -> w367
                  shift-left: w357 -> [w382]
                  tunnel: w371 -> [_] mode=indexing
                  # "Executes Lot Test\n1) First Wafer Loaded? - If the first wafer in the lot is already on the chuck, the user selects this and the loading wafer steps are skipped for the first iteration of the the for loop.\n2) Load wafer - loads the wafer from the cassette to the chuck\n3)wait - waits ten seconds  - if the profile command comes while the cwafer is still being loaded the probe station gives an error\n4) Profile z and autoalign - completes the rest of the loading procedure\n5) desired wafer to current wafer - changes wafer name to the next on on the \"Wafer List\"\n6) update wafer - update wafer info\n7) Runs auto test (see auto test tab)"
                  n145 = Enqueue Element(queue=w382, element="skip raw?", error in (no error)=w381) -> (queue out=w380:refnum<queue>, error out=w379:errorcluster)  [unwired: 1 in, 1 out]
                  n146 = Enqueue Element(queue=w380, element="pick device", error in (no error)=w379) -> (queue out=w388:refnum<queue>, error out=w387:errorcluster)  [unwired: 1 in, 1 out]
                  n147 = case shown="False" FALSE {
                    tunnel: w388 -> [w441 w454]
                    tunnel: w387 -> [w440 w455]
                    tunnel: [w438 w454] -> w386
                    tunnel: [w437 w455] -> w385
                    frame False {
                      n148 = local read "Enable Laser"() -> (w439:bool)
                      n149 = case shown="True" w439 {
                        tunnel: [w445 w453] -> w443
                        tunnel: [w444 w452] -> w442
                        tunnel: w441 -> [w445 w450]
                        tunnel: w440 -> [w444 w448]
                        frame False {
                        }
                        frame True {
                          n150 = Enqueue Element(queue=w450, element="Zero Laser", error in (no error)=w448) -> (queue out=w449:refnum<queue>, error out=w447:errorcluster)  [unwired: 1 in, 1 out]
                          n151 = Enqueue Element(queue=w449, element="Update Laser", error in (no error)=w447) -> (queue out=w453:refnum<queue>, error out=w452:errorcluster)  [unwired: 1 in, 1 out]
                        }
                      }
                      n152 = Enqueue Element(queue=w443, element="start raw", error in (no error)=w442) -> (queue out=w434:refnum<queue>, error out=w433:errorcluster)  [unwired: 1 in, 1 out]
                      n153 = Enqueue Element(queue=w434, element="select", error in (no error)=w433) -> (queue out=w438:refnum<queue>, error out=w437:errorcluster)  [unwired: 1 in, 1 out]
                    }
                    frame True {
                    }
                  }
                  n154 = local read "Enable Laser"() -> (w383:bool)
                  n155 = case shown="True" w383 {
                    tunnel: [w395 w411] -> w374
                    tunnel: [w394 w410] -> w375
                    tunnel: w386 -> [w393 w409]
                    tunnel: w385 -> [w392 w408]
                    frame False {
                      n156 = local read "Only Raw Test"() -> (w390:bool)
                      n157 = Not(x=w390) -> (.not. x?=w391:bool)
                      n158 = case shown="False" w391 {
                        tunnel: [w397 w405] -> w395
                        tunnel: [w396 w404] -> w394
                        tunnel: w393 -> [w397 w403]
                        tunnel: w392 -> [w396 w401]
                        frame False {
                        }
                        frame True {
                          n159 = Enqueue Element(queue=w403, element="find best devices mask", error in (no error)=w401) -> (queue out=w402:refnum<queue>, error out=w400:errorcluster)  [unwired: 1 in, 1 out]
                          n160 = Enqueue Element(queue=w402, element="start fine", error in (no error)=w400) -> (queue out=w405:refnum<queue>, error out=w404:errorcluster)  [unwired: 1 in, 1 out]
                        }
                      }
                    }
                    frame True {
                      n161 = local read "Only Raw Test"() -> (w406:bool)
                      n162 = Not(x=w406) -> (.not. x?=w407:bool)
                      n163 = case shown="True" w407 {
                        tunnel: [w413 w418] -> w411
                        tunnel: [w412 w417] -> w410
                        tunnel: w409 -> [w413 w416]
                        tunnel: w408 -> [w412 w415]
                        frame False {
                        }
                        frame True {
                          n164 = property on="Laser List" class="LstBox (strict)"() -> ("Item Names"=w414:string[])  [unwired: 2 in, 2 out]
                          n165 = for {
                            tunnel: [w432] -> w418
                            tunnel: [w431] -> w417
                            tunnel: w416 -> [w427]
                            tunnel: w415 -> [w430]
                            tunnel: w414 -> [_] mode=indexing
                            n166 = Enqueue Element(queue=w427, element="pick laser", error in (no error)=w430) -> (queue out=w426:refnum<queue>, error out=w428:errorcluster)  [unwired: 1 in, 1 out]
                            n167 = Enqueue Element(queue=w426, element="Update Laser", error in (no error)=w428) -> (queue out=w421:refnum<queue>, error out=w424:errorcluster)  [unwired: 1 in, 1 out]
                            n168 = Enqueue Element(queue=w421, element="find best devices mask", error in (no error)=w424) -> (queue out=w422:refnum<queue>, error out=w423:errorcluster)  [unwired: 1 in, 1 out]
                            n169 = Enqueue Element(queue=w422, element="start fine", error in (no error)=w423) -> (queue out=w432:refnum<queue>, error out=w431:errorcluster)  [unwired: 1 in, 1 out]
                          }
                        }
                      }
                    }
                  }
                  n170 = Enqueue Element(queue=w374, element="reset skip", error in (no error)=w375) -> (queue out=w377:refnum<queue>, error out=w376:errorcluster)  [unwired: 1 in, 1 out]
                }
                n171 = Enqueue Element(queue=w367, element="Zero Laser", error in (no error)=w366) -> (queue out=w370:refnum<queue>, error out=w369:errorcluster)  [unwired: 1 in, 1 out]
                n172 = Enqueue Element(queue=w370, element="update laser", error in (no error)=w369) -> (queue out=w365:refnum<queue>, error out=w364:errorcluster)  [unwired: 1 in, 1 out]
              }
              n173 = Enqueue Element(queue=w336, element="temp to 25", error in (no error)=w329) -> (queue out=w335:refnum<queue>, error out=w330:errorcluster)  [unwired: 1 in, 1 out]
              n174 = Enqueue Element(queue=w335, element="update temperature", error in (no error)=w330) -> (queue out=w334:refnum<queue>, error out=w331:errorcluster)  [unwired: 1 in, 1 out]
              n175 = Enqueue Element(queue=w334, element="update measurement log", error in (no error)=w331) -> (queue out=w333:refnum<queue>, error out=w332:errorcluster)  [unwired: 1 in, 1 out]
            }
          }
          event "update temp": Value Change {
            # "Gives the VISA commands to update chuck temperature"
            n176 = event-data() -> ()  [unwired: 1 in, 5 out]
            n177 = Enqueue Element(queue=w476, element="update temperature", error in (no error)=w475) -> (queue out=w474:refnum<queue>, error out=w473:errorcluster)  [unwired: 1 in, 1 out]
          }
          event "Add to Temp": Value Change {
            # "adds value from desired temperature to temperature list"
            n178 = event-data() -> ()  [unwired: 1 in, 5 out]
            n179 = Enqueue Element(queue=w481, element="add to temp list", error in (no error)=w480) -> (queue out=w479:refnum<queue>, error out=w478:errorcluster)  [unwired: 1 in, 1 out]
          }
          event "Remove from Temp": Value Change {
            # "removes highlighted value from temperature list"
            n180 = event-data() -> ()  [unwired: 1 in, 5 out]
            n181 = Enqueue Element(queue=w486, element="remove from temp list", error in (no error)=w485) -> (queue out=w484:refnum<queue>, error out=w483:errorcluster)  [unwired: 1 in, 1 out]
          }
          event "Clear temp list": Value Change {
            # "removes all values from temperature list"
            n182 = event-data() -> ()  [unwired: 1 in, 5 out]
            n183 = Enqueue Element(queue=w491, element="clear temp list", error in (no error)=w490) -> (queue out=w489:refnum<queue>, error out=w488:errorcluster)  [unwired: 1 in, 1 out]
          }
          event "load file for temp series": Value Change {
            # "works the same as loading manual mask file, but this is just in the temperature series tab"
            n184 = event-data() -> ()  [unwired: 1 in, 5 out]
            n185 = Enqueue Element(queue=w495, element="load file for temp", error in (no error)=w494) -> (queue out=w493:refnum<queue>, error out=w492:errorcluster)  [unwired: 1 in, 1 out]
          }
          event "move prober 2": Value Change {
            # "does the same as \"moveto\" from a different button"
            n186 = event-data() -> ()  [unwired: 1 in, 5 out]
            n187 = Enqueue Element(queue=w500, element="moveto", error in (no error)=w501) -> (queue out=w498:refnum<queue>, error out=w499:errorcluster)  [unwired: 1 in, 1 out]
          }
          event "Desired Device": Value Change {
            # "Does the same as \"Die number changed\" but from the temperature series tab"
            n188 = event-data() -> ()  [unwired: 1 in, 5 out]
            n189 = Enqueue Element(queue=w506, element="desired device change", error in (no error)=w505) -> (queue out=w504:refnum<queue>, error out=w503:errorcluster)  [unwired: 1 in, 1 out]
          }
          event "Start temp": Value Change {
            # "Begins Temperature Series\n1) Selects Temperature - updates current temprature from temp list\n2) Update temperature - writes current temperature to Temptronic TEC\n3) Wait fr temperature - waits until the temperature has settled on the correct value\n4) begin temperature series - runs a few fine tests with different tempreatures (in progress)"
            n190 = event-data() -> ()  [unwired: 1 in, 5 out]
            n191 = local read "Comments Temp"() -> (w507:string)
            n192 = local write "Test Type"("Temperature Test" ("Test Type")) -> ()
            n193 = local write "Comments"(w507) -> ()
            n194 = Enqueue Element(queue=w515, element="begin temperature series", error in (no error)=w514) -> (queue out=w512:refnum<queue>, error out=w511:errorcluster)  [unwired: 1 in, 1 out]
            n195 = Enqueue Element(queue=w512, element="update measurement log", error in (no error)=w511) -> (queue out=w510:refnum<queue>, error out=w509:errorcluster)  [unwired: 1 in, 1 out]
          }
          event "Refresh Device": Value Change {
            # "This is supposed to populate the device mane list from the given mask file. As of 8/5/18 it isn't working properly"
            n196 = event-data() -> ()  [unwired: 1 in, 5 out]
            n197 = Enqueue Element(queue=w521, element="refresh device names", error in (no error)=w520) -> (queue out=w519:refnum<queue>, error out=w518:errorcluster)  [unwired: 1 in, 1 out]
          }
          event "Add to list": Value Change {
            # "Adds device name value to test list"
            n198 = event-data() -> ()  [unwired: 1 in, 5 out]
            n199 = Enqueue Element(queue=w526, element="add to list", error in (no error)=w525) -> (queue out=w524:refnum<queue>, error out=w523:errorcluster)  [unwired: 1 in, 1 out]
          }
          event "Remove from List": Value Change {
            # "removes highlighted walue from test list"
            n200 = event-data() -> ()  [unwired: 1 in, 5 out]
            n201 = Enqueue Element(queue=w531, element="remove from list", error in (no error)=w529) -> (queue out=w530:refnum<queue>, error out=w528:errorcluster)  [unwired: 1 in, 1 out]
          }
          event "Clear List": Value Change {
            # "removes all entries from test list"
            n202 = event-data() -> ()  [unwired: 1 in, 5 out]
            n203 = Enqueue Element(queue=w536, element="clear list", error in (no error)=w535) -> (queue out=w534:refnum<queue>, error out=w533:errorcluster)  [unwired: 1 in, 1 out]
          }
          event "Load Wafer": Value Change {
            # "Loads wafer and performs profilng and auto alignment procedures"
            n204 = event-data() -> ()  [unwired: 1 in, 5 out]
            n205 = Enqueue Element(queue=w550, element="load wafer", error in (no error)=w549) -> (queue out=w541:refnum<queue>, error out=w540:errorcluster)  [unwired: 1 in, 1 out]
            n206 = Enqueue Element(queue=w541, element="wait", error in (no error)=w540) -> (queue out=w539:refnum<queue>, error out=w538:errorcluster)  [unwired: 1 in, 1 out]
            n207 = Enqueue Element(queue=w539, element="profile z", error in (no error)=w538) -> (queue out=w546:refnum<queue>, error out=w544:errorcluster)  [unwired: 1 in, 1 out]
            n208 = Enqueue Element(queue=w546, element="auto align", error in (no error)=w544) -> (queue out=w545:refnum<queue>, error out=w543:errorcluster)  [unwired: 1 in, 1 out]
          }
          event "Profile Z": Value Change {
            # "Performs just the z profile"
            n209 = event-data() -> ()  [unwired: 1 in, 5 out]
            n210 = Enqueue Element(queue=w555, element="profile z", error in (no error)=w553) -> (queue out=w554:refnum<queue>, error out=w552:errorcluster)  [unwired: 1 in, 1 out]
          }
          event "Add to Laser": Value Change {
            # "adds desired laser value to laser list"
            n211 = event-data() -> ()  [unwired: 1 in, 5 out]
            n212 = Enqueue Element(queue=w559, element="add to laser list", error in (no error)=w558) -> (queue out=w556:refnum<queue>, error out=w557:errorcluster)  [unwired: 1 in, 1 out]
          }
          event "Remove from Laser List": Value Change {
            # "removes highlighted value from laser list"
            n213 = event-data() -> ()  [unwired: 1 in, 5 out]
            n214 = Enqueue Element(queue=w564, element="remove from laser list", error in (no error)=w563) -> (queue out=w561:refnum<queue>, error out=w562:errorcluster)  [unwired: 1 in, 1 out]
          }
          event "Clear Laser List": Value Change {
            # "removes all entries from laser list"
            n215 = event-data() -> ()  [unwired: 1 in, 5 out]
            n216 = Enqueue Element(queue=w569, element="clear laser list", error in (no error)=w567) -> (queue out=w568:refnum<queue>, error out=w566:errorcluster)  [unwired: 1 in, 1 out]
          }
          event "Add to wafer list": Value Change {
            # "Adds desired value to wafer list"
            n217 = event-data() -> ()  [unwired: 1 in, 5 out]
            n218 = Enqueue Element(queue=w575, element="add to wafer list", error in (no error)=w574) -> (queue out=w572:refnum<queue>, error out=w571:errorcluster)  [unwired: 1 in, 1 out]
          }
          event "Remove from wafer list": Value Change {
            # "removes highlighted value from wafer list"
            n219 = event-data() -> ()  [unwired: 1 in, 5 out]
            n220 = Enqueue Element(queue=w579, element="remove from wafer list", error in (no error)=w578) -> (queue out=w577:refnum<queue>, error out=w576:errorcluster)  [unwired: 1 in, 1 out]
          }
          event "Clear wafer list": Value Change {
            # "removes all values from wafer list"
            n221 = event-data() -> ()  [unwired: 1 in, 5 out]
            n222 = Enqueue Element(queue=w584, element="clear wafer list", error in (no error)=w583) -> (queue out=w582:refnum<queue>, error out=w581:errorcluster)  [unwired: 1 in, 1 out]
          }
          event "Update viewer": Value Change {
            # "Updates the measurement log viewer from the csv file in case of manual changes to the log"
            n223 = event-data() -> ()  [unwired: 1 in, 5 out]
            n224 = Enqueue Element(queue=w590, element="update viewer", error in (no error)=w589) -> (queue out=w588:refnum<queue>, error out=w587:errorcluster)  [unwired: 1 in, 1 out]
          }
          event "Save Comment": Value Change {
            # "Saves the comment to the highlighted entry in the measurement log, and updates the viewer to match the csv file. I still havent gotten the measurement log to close automatically however"
            n225 = event-data() -> ()  [unwired: 1 in, 5 out]
            n226 = Enqueue Element(queue=w598, element="save comment", error in (no error)=w597) -> (queue out=w595:refnum<queue>, error out=w593:errorcluster)  [unwired: 1 in, 1 out]
            n227 = Enqueue Element(queue=w595, element="update viewer", error in (no error)=w593) -> (queue out=w594:refnum<queue>, error out=w592:errorcluster)  [unwired: 1 in, 1 out]
          }
          event "Explore Data": Value Change {
            n228 = event-data() -> ()  [unwired: 1 in, 5 out]
            n229 = Enqueue Element(queue=w602, element="explore data", error in (no error)=w601) -> (queue out=w600:refnum<queue>, error out=w599:errorcluster)  [unwired: 1 in, 1 out]
          }
        }
      }
      n230 = while {
        shift-right: [w611] -> _
        shift-left: w35 -> [w608]
        shift-right: [w610] -> _
        shift-left: w34 -> [w607]
        stop <- w613 stop-if-true
        n231 = local read "Laser Current (mA)"() -> (w605:dbl)
        n232 = Dequeue Element(queue=w608, error in (no error)=w607) -> (queue out=w606:refnum<queue>, element=w612:string, error out=w609:errorcluster)  [unwired: 1 in, 1 out]
        n233 = Greater Than 0?(x=w605) -> (x > 0?=w604:bool)
        n234 = case shown="\"update wafer\"" w612 {
          tunnel: [_ TRUE _ _ _ _ _ _ _ _ _ _ _ _ _ _ _ _ _ _ _ _ _ _ _ _ _ _ _ _ _ _ _ _ _ _ _ _ _ _ _ _ _ _ _ _ _ _ _ _ _ _ _ _ _ _ _ _ _] -> w613
          tunnel: w609 -> [w615 w617 w621 w817 w861 w871 w881 w911 w934 w944 w975 w1177 w1183 w1192 w1204 w1210 w1222 w1258 w1301 w1338 w1570 w1572 w1607 w1615 w1625 w1630 w1681 w1693 w1704 w1726 w1748 w1750 w1755 w1761 w1767 w1777 w1782 w1785 w1789 w1804 w1822 w1837 w1847 w1849 w1857 w1862 w1867 w1870 w1873 w1892 w1906 w1930 w1934 w1965 w2241 w2246 w2249 w2251 w2256]
          tunnel: [w615 w617 w622 w817 w862 w868 w878 w914 w935 w947 w974 w1177 w1187 w1192 w1204 w1209 w1224 w1258 w1303 w1340 w1570 w1572 w1607 w1617 w1627 w1630 w1681 w1690 w1707 w1726 w1748 w1750 w1755 w1763 w1770 w1777 w1782 w1785 w1788 w1804 w1822 w1837 w1847 w1849 w1857 w1862 w1867 w1870 w1873 w1892 w1906 w1930 w1933 w1965 w2241 w2246 w2249 w2251 w2256] -> w610
          tunnel: w606 -> [w614 w616 w624 w818 w864 w870 w880 w912 w937 w949 w972 w1178 w1189 w1193 w1205 w1208 w1223 w1259 w1302 w1337 w1571 w1573 w1608 w1616 w1626 w1631 w1682 w1694 w1706 w1727 w1749 w1751 w1756 w1762 w1769 w1778 w1783 w1786 w1791 w1805 w1823 w1838 w1848 w1850 w1858 w1863 w1868 w1871 w1874 w1893 w1907 w1931 w1936 w1966 w2242 w2247 w2250 w2252 w2257]
          tunnel: [w614 w616 w623 w818 w863 w869 w879 w913 w936 w948 w973 w1178 w1188 w1193 w1205 w1207 w1225 w1259 w1304 w1339 w1571 w1573 w1608 w1618 w1628 w1631 w1682 w1695 w1708 w1727 w1749 w1751 w1756 w1764 w1771 w1778 w1783 w1786 w1790 w1805 w1823 w1838 w1848 w1850 w1858 w1863 w1868 w1871 w1874 w1893 w1907 w1931 w1935 w1966 w2242 w2247 w2250 w2252 w2257] -> w611
          tunnel: w604 -> [_ _ _ _ _ _ _ _ _ _ _ _ _ _ _ _ _ _ _ w1341 _ _ _ _ _ _ _ _ _ _ _ _ _ _ _ _ _ _ _ _ _ _ _ _ _ _ _ _ _ _ _ _ _ _ _ _ _ _ _]
          frame "False", Default {
          }
          frame "stop" {
            # "Ends the for loop that contains the event structure, effectively ending the program"
          }
          frame "start raw" {
            # "Raw Test:\n(If Raw Test Skipped is TRUE, the entire raw test is not run. This only happens as part of the auto or lot tests)\n1) Loads mask file and updates info\n2) Finds/Creates directory for new Raw test file and creates file\n3) Runs raw test and updates graph after every measurement is taken\n4) Resets the prober to 0 0"
            n235 = local read "Raw Test Skipped"() -> (w620:bool)
            n236 = Not(x=w620) -> (.not. x?=w619:bool)
            n237 = case shown="True" w619 {
              frame False {
              }
              frame True {
                n238 = flat-sequence {
                  tunnel: [w638] -> w628
                  tunnel: w628 -> [w674]
                  tunnel: [w674] -> w627
                  tunnel: [w667] -> w626
                  tunnel: w627 -> [w676]
                  tunnel: w626 -> [w675]
                  frame #0 {
                    n239 = local read "Wafer Name"() -> (w636:string)
                    n240 = local read "RawTest ID"() -> (w641:u32)
                    n241 = local read "Scribe"() -> (w635:string)
                    n242 = local read "Mask"() -> (w634:string)
                    n243 = local read "Lot"() -> (w633:string)
                    n244 = local write "Status"("Prepare raw test" ("Status")) -> ()
                    n245 = Bundle By Name(cluster="Wafer Info 2", "Wafer Name"=w636, "Scribe"=w635, "Mask"=w634, "Lot"=w633) -> (w637:T9)
                    n246 = local write "Tab Control"(T16."Raw Test" ("Tab Control")) -> ()
                    n247 = Increment(x=w641) -> (x+1=w640:u32)
                    n248 = call "Device Files v1.vi"("Rows"=1200, "Mask file path"="Mask File Raw") -> ("size(s)"=w638:i32, "Array of Cell Clusters"=→"Array of Cell Data Clusters":T5)  [unwired: 6 in, 2 out]
                    "Total Device" <- w638
                    n249 = local write "Wafer Info"(w637) -> ()
                    n250 = local write "RawTest ID"(w640) -> ()
                    n251 = Initialize Array(nan ("element"), w638) -> (w631:dbl[])
                    n252 = local write "V meas"(w631) -> ()
                    n253 = local write "I meas"(w631) -> ()
                    n254 = Bundle(w631, w631) -> (→"Selected Data":cluster{dbl[], dbl[]})  [unwired: 1 in]
                    "Progress" <- u8 0 ("Progress")
                  }
                  frame #1 {
                    n255 = local read "Array of Cell Data Clusters"() -> (w673:T12)
                    n256 = local read "RawData Save Path"() -> (w649:path)
                    n257 = local read "Lot"() -> (w655:string)
                    n258 = Build Path(base path=w649, name or relative path=w655) -> (appended path=w654:path)
                    n259 = Index Array(array=w673, index=0) -> (element=w671:T17)
                    n260 = call "CreateDirectory.vi"("Path to be created"=w654) -> ()  [unwired: 10 in, 1 out]
                    n261 = local read "Wafer Name"() -> (w653:string)
                    n262 = Unbundle By Name(w671) -> ("Cell Name"=w670:string)
                    n263 = Build Path(base path=w654, name or relative path=w653) -> (appended path=w652:path)
                    n264 = call "get RawTest filename.vi"("Device Name"=w670, "Wafer Name"=w653) -> ("current time"=w664:timestamp, "FileName"=w669:string)  [unwired: 8 in]
                    n265 = call "CreateDirectory.vi"("Path to be created"=w652) -> ()  [unwired: 10 in, 1 out]
                    n266 = local write "Test FileName"(w669) -> ()
                    n267 = local read "Laser Current (mA)"() -> (w658:dbl)
                    n268 = local read "V compliance"() -> (w659:dbl)
                    n269 = local read "I compliance"() -> (w662:dbl)
                    n270 = local read "J set A/cm2"() -> (w661:dbl)
                    n271 = local read "RawTest ID"() -> (w657:u32)
                    n272 = local read "Operator"() -> (w656:string)
                    n273 = local read "V set"() -> (w663:dbl)
                    n274 = local read "I set"() -> (w660:dbl)
                    n275 = Bundle By Name(cluster="Session Info 2", "V set"=w663, "I compliance"=w662, "J set"=w661, "I set"=w660, "V compliance"=w659, "Laser Power (mW)"=w658, "TestID"=w657, "Session Time"=w664, "Operator"=w656) -> (w665:T7)
                    n276 = Build Path(base path=w652, name or relative path="Raw Data") -> (appended path=w650:path)
                    "new raw data save path" <- w650
                    n277 = local write "Session Info"(w665) -> ()
                    n278 = call "CreateDirectory.vi"("Path to be created"=w650) -> ("Output"=w647:path)  [unwired: 10 in]
                    n279 = Build Path(base path=w647, name or relative path=w669) -> (appended path=w648:path)
                    "Raw Test Filename" <- w648
                    n280 = call "writeFile RawTestHead.vi"("Name Array"="Name Array", "Path"=w648) -> ("Path out"=w667:path)  [unwired: 9 in]
                    "RawData file" <- w667
                  }
                  frame #2 {
                    n281 = for {
                      N: w676 -> [w689]
                      tunnel: w675 -> [w677]
                      i -> [w678]
                      n282 = Divide(x=w678, y=w689) -> (x/y=w687:dbl)
                      n283 = flat-sequence {
                        tunnel: [w723] -> w698
                        tunnel: [w722] -> w697
                        tunnel: w678 -> [w716]
                        tunnel: [w718] -> w693
                        tunnel: [w717] -> w692
                        tunnel: [w700] -> w691
                        tunnel: [w699] -> w690
                        tunnel: w698 -> [w724]
                        tunnel: w697 -> [w732]
                        tunnel: [w731] -> w696
                        tunnel: [w730] -> w695
                        tunnel: w693 -> [w728]
                        tunnel: w692 -> [w727]
                        tunnel: w691 -> [w726]
                        tunnel: w690 -> [w725]
                        tunnel: w696 -> [w735]
                        tunnel: w695 -> [w734]
                        tunnel: [w737] -> w694
                        tunnel: w694 -> [w761]
                        tunnel: [w761] -> w680
                        tunnel: [w762] -> w679
                        tunnel: w680 -> [w794]
                        tunnel: w679 -> [w793]
                        tunnel: w678 -> [w800]
                        tunnel: w677 -> [w791]
                        frame #0 {
                          n284 = Increment(x=w716) -> (x+1=→"Current Device":i32)
                          n285 = local read "Array of Cell Data Clusters"() -> (w720:T12)
                          n286 = local read "Laser Current (mA)"() -> (w712:dbl)
                          n287 = Index Array(array=w720, index=w716) -> (element=w713:T17)
                          n288 = local read "Device Name"() -> (w703:string)
                          n289 = Unbundle By Name(w713) -> ("X-coord"=w700:dbl, "Y-coord"=w699:dbl, "Area"=w701:dbl, "Meas Area"=w702:dbl, "Cell Name"=w706:string)
                          n290 = call "get Area.vi"("Laser"=w712, "Cell Data Cluster"=w713) -> ("Area"=w710:dbl)  [unwired: 9 in]
                          n291 = local read "J set A/cm2"() -> (w708:dbl)
                          n292 = local write "ActiveArea_um2"(w701) -> ()
                          n293 = local write "MesaArea_um2"(w702) -> ()
                          n294 = local write "Device Name"(w706) -> ()
                          n295 = Divide(x=w710, y=100000000.0) -> (x/y=w709:dbl)
                          n296 = Bundle By Name(cluster="Die Info 2", "Device Name"=w703, "ActiveArea_um2"=w701, "MesaArea_um2"=w702, "x"=w700, "y"=w699) -> (w704:T8)
                          n297 = Multiply(x=w708, y=w709) -> (x*y=w707:dbl)
                          n298 = local read "Prober GPIB"() -> (w714:string)
                          n299 = local read "current y"() -> (w719:i32)
                          n300 = local read "current x"() -> (w721:i32)
                          n301 = local write "Die Info"(w704) -> ()
                          n302 = local write "I set"(w707) -> ()
                          n303 = Subtract(x=w699, y=w719) -> (x-y=w717:dbl)
                          n304 = Subtract(x=w700, y=w721) -> (x-y=w718:dbl)
                          n305 = call "EG2001 Move Z Down.vi"("GPIB Address"=w714) -> ("Error Out"=w722:errorcluster, "GPIB Address Out"=w723:string)  [unwired: 9 in]
                        }
                        frame #1 {
                          n306 = local write "current x"(w726) -> ()
                          n307 = local write "current y"(w725) -> ()
                          n308 = call "EG2001 Move Machine Step X-Y.vi"("Flip X Coordinates?"=FALSE, "Y"=w727, "Steps/Microns"=enum32{"Steps", "Microns"}."Microns", "X"=w728, "error in (no error)"=w732, "GPIB Address"=w724) -> ("Error Out"=w730:errorcluster, "GPIB Address Out"=w731:string)  [unwired: 4 in]
                        }
                        frame #2 {
                          n309 = call "EG2001 Move Z Up.vi"("error in (no error)"=w734, "GPIB Address"=w735) -> ()  [unwired: 10 out]
                        }
                        frame #3 {
                          n310 = local read "Keysight"() -> (w736:bool)
                          n311 = case shown="False" w736 {
                            tunnel: [w738 w759] -> w737
                            frame False {
                              n312 = local read "Channel Keysight"() -> (w748:dbl)
                              n313 = local read "Imeas Settings"() -> (w742:T11)
                              n314 = local read "I compliance"() -> (w746:dbl)
                              n315 = local read "Id delay ms"() -> (w744:dbl)
                              n316 = local read "Repeat Id"() -> (w745:u32)
                              n317 = local read "4-wire"() -> (w741:bool)
                              n318 = local read "NPLC"() -> (w747:dbl)
                              n319 = local read "V set"() -> (w743:dbl)
                              n320 = local read "Keysight SMU"() -> (w739:refnum<visa-resource-name>)
                              n321 = Bundle By Name(cluster=w742, "Channel"=w748, "Vset"=w743, "NPLC"=w747, "I compliance"=w746, "Repeat time"=w745, "Delay ms"=w744, "4-wire"=w741) -> (w740:T11)
                              n322 = call "Agilent B2900 Measure I at Vset.vi"("Imeas Settings"=w740, "VISA resource name"=w739) -> ("Avg I"=w738:dbl)  [unwired: 9 in]
                              n323 = local write "Imeas Settings"(w740) -> ()
                            }
                            frame True {
                              n324 = local read "Imeas Settings"() -> (w751:T11)
                              n325 = local read "I compliance"() -> (w755:dbl)
                              n326 = local read "Id delay ms"() -> (w753:dbl)
                              n327 = local read "Repeat Id"() -> (w754:u32)
                              n328 = local read "Channel"() -> (w757:enum32{"Channel A", "Channel B"})
                              n329 = local read "4-wire"() -> (w750:bool)
                              n330 = local read "NPLC"() -> (w756:dbl)
                              n331 = local read "V set"() -> (w752:dbl)
                              n332 = local read "Keithley SMU"() -> (w758:refnum<visa-resource-name>)
                              n333 = Bundle By Name(cluster=w751, "Channel"=w757, "Vset"=w752, "NPLC"=w756, "I compliance"=w755, "Repeat time"=w754, "Delay ms"=w753, "4-wire"=w750) -> (w749:T11)
                              n334 = local write "Imeas Settings"(w749) -> ()
                              n335 = call "K2602 setVmeasI.vi"("Settings"=w749, "SMU"=w758) -> ("Iavg"=w759:dbl)  [unwired: 6 in, 3 out]
                            }
                          }
                        }
                        frame #4 {
                          n336 = local read "Keysight"() -> (w760:bool)
                          n337 = case shown="False" w760 {
                            tunnel: [w763 w778] -> w762
                            frame False {
                              n338 = local read "Vmeas Settings"() -> (w773:T11)
                              n339 = local read "V compliance"() -> (w771:dbl)
                              n340 = local read "Vf delay ms"() -> (w769:dbl)
                              n341 = local read "Repeat Vf"() -> (w770:u32)
                              n342 = local read "Channel"() -> (w772:enum32{"Channel A", "Channel B"})
                              n343 = local read "4-wire"() -> (w766:bool)
                              n344 = local read "NPLC"() -> (w768:dbl)
                              n345 = local read "I set"() -> (w767:dbl)
                              n346 = local read "Keysight SMU"() -> (w764:refnum<visa-resource-name>)
                              n347 = Bundle By Name(cluster=w773, "Channel"=w772, "Vset"=w767, "NPLC"=w768, "I compliance"=w771, "Repeat time"=w770, "Delay ms"=w769, "4-wire"=w766) -> (w765:T11)
                              n348 = call "Agilent B2900 Measure V at Iset.vi"("Imeas Settings"=w765, "VISA resource name"=w764) -> ("Avg V"=w763:dbl)  [unwired: 9 in]
                              n349 = local write "Vmeas Settings"(w765) -> ()
                            }
                            frame True {
                              n350 = local read "Channel Keysight"() -> (w782:dbl)
                              n351 = local read "Vmeas Settings"() -> (w783:T11)
                              n352 = local read "V compliance"() -> (w781:dbl)
                              n353 = local read "Vf delay ms"() -> (w779:dbl)
                              n354 = local read "Repeat Vf"() -> (w780:u32)
                              n355 = local read "4-wire"() -> (w775:bool)
                              n356 = local read "NPLC"() -> (w777:dbl)
                              n357 = local read "I set"() -> (w776:dbl)
                              n358 = Bundle By Name(cluster=w783, "Channel"=w782, "Vset"=w776, "NPLC"=w777, "I compliance"=w781, "Repeat time"=w780, "Delay ms"=w779, "4-wire"=w775) -> (w774:T11)
                              n359 = local write "Vmeas Settings"(w774) -> ()
                              n360 = call "K2602 setImeasV.vi"("Settings"=w774) -> ("Vavg"=w778:dbl)  [unwired: 7 in, 3 out]
                            }
                          }
                        }
                        frame #5 {
                          n361 = local read "I meas"() -> (w802:dbl[])
                          n362 = local read "V meas"() -> (w801:dbl[])
                          n363 = Replace Array Subset(array=w802, new element=w794, index=w800) -> (w797:dbl[])
                          n364 = Get Date/Time In Seconds() -> (seconds since 1Jan1904=w792:timestamp)
                          n365 = local read "Session Info"() -> (w787:T7)
                          n366 = local read "Wafer Info"() -> (w789:T9)
                          n367 = local read "Die Info"() -> (w788:T8)
                          n368 = local write "I meas"(w797) -> ()
                          n369 = Bundle By Name(cluster="Test Results 2", "I meas"=w794, "V meas"=w793, "Time"=w792) -> (w790:T6)
                          n370 = Replace Array Subset(array=w801, new element=w793, index=w800) -> (w796:dbl[])
                          n371 = local read "Selected Data"() -> (w785:cluster{dbl[], dbl[]})
                          n372 = local write "V meas"(w796) -> ()
                          n373 = call <vilib>:"Histogram.vi"("X"=w796) -> ("Histogram Graph"=→"Vforward hist":T14)  [unwired: 7 in, 3 out]
                          n374 = Bundle("V meas"=w796, "I meas"=w797) -> (w786:cluster{"V meas":dbl[], "I meas":dbl[]})  [unwired: 1 in]
                          n375 = call "writeFile RawTestData.vi"("Test Results"=w790, "Session Info"=w787, "Die Info"=w788, "Wafer Info"=w789, "Path"=w791) -> ()  [unwired: 6 in, 1 out]
                          n376 = local write "Test Results"(w790) -> ()
                          n377 = call <vilib>:"Histogram.vi"("X"=w797) -> ("Histogram Graph"=→"Idark hist":T14)  [unwired: 7 in, 3 out]
                          n378 = Build Array(w786, w785) -> (→"Spec Plot":cluster{"V meas":dbl[], "I meas":dbl[]}[])
                        }
                      }
                      n379 = Increment(x=w678) -> (x+1=w681:i32)
                      n380 = Multiply(x=w687, y=100.0) -> (x*y=w685:dbl)
                      n381 = To Unsigned Byte Integer(number=w685) -> (unsigned 8bit integer=w688:u8)
                      n382 = Number To Decimal String(number=w681) -> (decimal integer string=w683:string)  [unwired: 1 in]
                      n383 = local write "Progress"(w688) -> ()
                      n384 = Concatenate Strings("Raw Test for die number:" ("string"), w683) -> (w684:string)
                      n385 = local write "Status"(w684) -> ()
                    }
                  }
                  frame #3 {
                    w807 = -1
                    n386 = local read "Prober GPIB"() -> (w814:string)
                    n387 = local read "RawTest ID"() -> (w804:u32)
                    n388 = local read "TestID file"() -> (w803:path)
                    n389 = local read "current y"() -> (w808:i32)
                    n390 = local read "current x"() -> (w809:i32)
                    n391 = Multiply(x=w807, y=w808) -> (x*y=w805:i32)
                    n392 = Multiply(x=w807, y=w809) -> (x*y=w806:i32)
                    n393 = call "writeFile TestID.vi"("TestID"=w804, "Path"=w803) -> ()  [unwired: 10 in]
                    n394 = call "EG2001 Move Z Down.vi"("GPIB Address"=w814) -> ("Error Out"=w813:errorcluster, "GPIB Address Out"=w812:string)  [unwired: 9 in]
                    n395 = call "EG2001 Move Machine Step X-Y.vi"("Flip X Coordinates?"=FALSE, "Y"=w805, "Steps/Microns"=enum32{"Steps", "Microns"}."Microns", "X"=w806, "error in (no error)"=w813, "GPIB Address"=w812) -> ()  [unwired: 4 in, 2 out]
                  }
                  frame #4 {
                    w815 = 0
                    n396 = local write "current y"(w815) -> ()
                    n397 = local write "current x"(w815) -> ()
                  }
                }
              }
            }
            n398 = Enqueue Element At Opposite End(queue=w624, element="idle", error in (no error)=w621) -> (queue out=w623:refnum<queue>, error out=w622:errorcluster)  [unwired: 1 in, 1 out]
          }
          frame "find best devices mask" {
            # "If raw test is skipped - this searches through the saving structure (see guide) by lot, wafer name, and device name to find previous raw test measurements. When the file is found, it updates the fine mask file. If no file is found, a dialogue box alets the user of that"
            n399 = local read "Raw Test Skipped"() -> (w816:bool)
            n400 = case shown="True" w816 {
              frame False {
              }
              frame True {
                w832 = path "C:/Users/Flash/Desktop/Data/Detector test data" ("path")
                n401 = List Folder(path=w832) -> (folder names=w831:string[])  [unwired: 3 in, 3 out]
                n402 = for {
                  tunnel: w831 -> [w841] mode=indexing
                  tunnel: [w840] -> w833
                  tunnel: [w839] -> w823
                  stop <- w839 stop-if-true
                  n403 = local read "Lot"() -> (w840:string)
                  n404 = Equal?(x=w841, y=w840) -> (x = y?=w839:bool)
                }
                n405 = Build Path(base path=w832, name or relative path=w833) -> (appended path=w828:path)
                n406 = List Folder(path=w828) -> (folder names=w830:string[])  [unwired: 3 in, 3 out]
                n407 = for {
                  tunnel: w830 -> [w838] mode=indexing
                  tunnel: [w837] -> w829
                  tunnel: [w836] -> w825
                  stop <- w836 stop-if-true
                  n408 = local read "Wafer Name"() -> (w837:string)
                  n409 = Equal?(x=w838, y=w837) -> (x = y?=w836:bool)
                }
                n410 = Build Path(base path=w828, name or relative path=w829) -> (appended path=w821:path)
                n411 = Build Path(base path=w821, name or relative path="Raw Data") -> (appended path=w820:path)
                n412 = List Folder(path=w820) -> (filenames=w827:string[])  [unwired: 3 in, 3 out]
                n413 = for {
                  tunnel: w827 -> [w852] mode=indexing
                  tunnel: [w852] -> w834
                  tunnel: [w845] -> w826
                  stop <- w845 stop-if-true
                  w851 = "" ("y")
                  n414 = local read "Device Name"() -> (w844:string)
                  n415 = local read "Wafer Name"() -> (w855:string)
                  n416 = Concatenate Strings(w844, "_" ("string")) -> (w842:string)
                  n417 = Match Pattern(string=w852, regular expression="mask") -> (after substring=w850:string)  [unwired: 1 in, 3 out]
                  n418 = Match Pattern(string=w852, regular expression=w842) -> (after substring=w856:string)  [unwired: 1 in, 3 out]
                  n419 = Match Pattern(string=w852, regular expression=w855) -> (after substring=w854:string)  [unwired: 1 in, 3 out]
                  n420 = Not Equal?(x=w856, y=w851) -> (x != y?=w857:bool)
                  n421 = Not Equal?(x=w851, y=w854) -> (x != y?=w848:bool)
                  n422 = Not Equal?(x=w851, y=w850) -> (x != y?=w849:bool)
                  n423 = And(x=w857, y=w848) -> (x .and. y?=w846:bool)
                  n424 = And(x=w848, y=w849) -> (x .and. y?=w847:bool)
                  n425 = And(x=w846, y=w847) -> (x .and. y?=w845:bool)
                }
                n426 = Or(x=w826, y=w825) -> (x .or. y?=w824:bool)
                n427 = Build Path(base path=w820, name or relative path=w834) -> (appended path=w835:path)
                n428 = Or(x=w824, y=w823) -> (x .or. y?=w822:bool)
                n429 = local write "Mask File Fine"(w835) -> ()
                n430 = case shown="False" w822 {
                  frame False {
                    n431 = local write "no file"(TRUE ("no file")) -> ()
                    n432 = One Button Dialog(message="There is no file from which to run the fine test") -> ()  [unwired: 1 in, 1 out]
                  }
                  frame True {
                  }
                }
              }
            }
          }
          frame "reset xy" {
            # "Pretty Obvious"
            n433 = local read "Prober GPIB"() -> (w860:string)
            n434 = Enqueue Element At Opposite End(queue=w864, element="idle", error in (no error)=w861) -> (queue out=w863:refnum<queue>, error out=w862:errorcluster)  [unwired: 1 in, 1 out]
            n435 = call "EG2001 Move First.vi"("GPIB Address"=w860) -> ()  [unwired: 9 in, 2 out]
            "current x" <- u32 0 ("current x")
            "current y" <- u32 0 ("current y")
          }
          frame "reset to 1st die" {
            # "Moves prober to first die"
            n436 = Enqueue Element At Opposite End(queue=w870, element="idle", error in (no error)=w871) -> (queue out=w869:refnum<queue>, error out=w868:errorcluster)  [unwired: 1 in, 1 out]
            n437 = local read "Array of Cell Data Clusters"() -> (w877:T12)
            n438 = Index Array(array=w877, index=0) -> (element=w875:T17)
            n439 = Unbundle By Name(w875) -> ("X-coord"=w874:dbl, "Y-coord"=w873:dbl)
            n440 = local write "current x"(w874) -> ()
            n441 = local write "current y"(w873) -> ()
          }
          frame "load file manual" {
            # "Update informaiton from mask file to relevant variables"
            n442 = Enqueue Element At Opposite End(queue=w880, element="idle", error in (no error)=w881) -> (queue out=w879:refnum<queue>, error out=w878:errorcluster)  [unwired: 1 in, 1 out]
            n443 = flat-sequence {
              tunnel: [w887] -> w883
              tunnel: w883 -> [w891]
              frame #0 {
                n444 = local write "Status"("Loading mask file" ("Status")) -> ()
                n445 = call "Device Files v1.vi"("Rows"=1200, "Mask file path"="Mask File Manual") -> ("Mask Name"=w888:string, "size(s)"=w887:i32, "Array of Cell Clusters"=w884:T5)  [unwired: 6 in, 1 out]
                n446 = local write "Mask"(w888) -> ()
                n447 = local write "Array of Cell Data Clusters"(w884) -> ()
              }
              frame #1 {
                n448 = for {
                  N: w891 -> [_]
                  tunnel: [w892] -> w890 mode=indexing
                  i -> [w893]
                  n449 = Number To Decimal String(number=w893) -> (decimal integer string=w892:string)  [unwired: 1 in]
                }
                n450 = property on="Die Number" class="Ring (strict)"("Strings []"=w890) -> ()  [unwired: 2 in, 2 out]
              }
              frame #2 {
                n451 = local read "Die Number"() -> (w900:u16)
                n452 = local read "Array of Cell Data Clusters"() -> (w901:T12)
                n453 = Index Array(array=w901, index=w900) -> (element=w899:T17)
                n454 = Unbundle By Name(w899) -> ("Cell Name"=w894:string, "X-coord"=w897:dbl, "Y-coord"=w898:dbl, "Area"=w896:dbl, "Meas Area"=w895:dbl)
                n455 = local write "Device Name"(w894) -> ()
                n456 = local write "x target"(w897) -> ()
                n457 = local write "y target"(w898) -> ()
                n458 = local write "ActiveArea_um2"(w896) -> ()
                n459 = local write "MesaArea_um2"(w895) -> ()
              }
              frame #3 {
                n460 = local read "J set A/cm2"() -> (w907:dbl)
                n461 = local read "Laser Current (mA)"() -> (w904:dbl)
                n462 = Equal To 0?(x=w904) -> (x = 0?=w903:bool)
                n463 = case shown="False" w903 {
                  tunnel: [w909 w910] -> w902
                  frame False {
                    n464 = local read "ActiveArea_um2"() -> (w909:dbl)
                  }
                  frame True {
                    n465 = local read "MesaArea_um2"() -> (w910:dbl)
                  }
                }
                n466 = Divide(x=w902, y=100000000.0) -> (x/y=w906:dbl)
                n467 = Multiply(x=w906, y=w907) -> (x*y=w908:dbl)
                n468 = local write "I set"(w908) -> ()
              }
            }
          }
          frame "Die number picked" {
            # "Update target x and y when a new die is picked in the manual test tab"
            n469 = Enqueue Element At Opposite End(queue=w912, element="idle", error in (no error)=w911) -> (queue out=w913:refnum<queue>, error out=w914:errorcluster)  [unwired: 1 in, 1 out]
            n470 = local write "Status"("Changing Die" ("Status")) -> ()
            n471 = flat-sequence {
              frame #0 {
                n472 = local read "Die Number"() -> (w923:u16)
                n473 = local read "Array of Cell Data Clusters"() -> (w924:T12)
                n474 = Index Array(array=w924, index=w923) -> (element=w922:T17)
                n475 = Unbundle By Name(w922) -> ("Cell Name"=w919:string, "X-coord"=w921:dbl, "Y-coord"=w920:dbl, "Area"=w918:dbl, "Meas Area"=w917:dbl)
                n476 = local write "Device Name"(w919) -> ()
                n477 = local write "x target"(w921) -> ()
                n478 = local write "y target"(w920) -> ()
                n479 = local write "ActiveArea_um2"(w918) -> ()
                n480 = local write "MesaArea_um2"(w917) -> ()
              }
              frame #1 {
                n481 = local read "J set A/cm2"() -> (w930:dbl)
                n482 = local read "Laser Current (mA)"() -> (w927:dbl)
                n483 = Equal To 0?(x=w927) -> (x = 0?=w926:bool)
                n484 = case shown="True" w926 {
                  tunnel: [w932 w933] -> w925
                  frame False {
                    n485 = local read "ActiveArea_um2"() -> (w932:dbl)
                  }
                  frame True {
                    n486 = local read "MesaArea_um2"() -> (w933:dbl)
                  }
                }
                n487 = Divide(x=w925, y=100000000.0) -> (x/y=w929:dbl)
                n488 = Multiply(x=w929, y=w930) -> (x*y=w931:dbl)
                n489 = local write "I set"(w931) -> ()
              }
            }
          }
          frame "Jset change" {
            # "Updates Current setpoint for a desired current density"
            n490 = local read "J set A/cm2"() -> (w940:dbl)
            n491 = Enqueue Element At Opposite End(queue=w937, element="idle", error in (no error)=w934) -> (queue out=w936:refnum<queue>, error out=w935:errorcluster)  [unwired: 1 in, 1 out]
            n492 = local read "ActiveArea_um2"() -> (w943:dbl)
            n493 = Divide(x=w943, y=100000000.0) -> (x/y=w941:dbl)
            n494 = Multiply(x=w941, y=w940) -> (x*y=w939:dbl)
            n495 = local write "I set"(w939) -> ()
          }
          frame "moveto" {
            # "Moves from current xy to target xy, and then changes current xy to match lcation"
            n496 = Enqueue Element At Opposite End(queue=w949, element="idle", error in (no error)=w944) -> (queue out=w948:refnum<queue>, error out=w947:errorcluster)  [unwired: 1 in, 1 out]
            n497 = flat-sequence {
              tunnel: [w954] -> w946
              tunnel: [w953] -> w945
              tunnel: w946 -> [w959]
              tunnel: w945 -> [w958]
              frame #0 {
                n498 = local read "Prober GPIB"() -> (w952:string)
                n499 = local write "Status"("Probe up" ("Status")) -> ()
                n500 = call "EG2001 Move Z Down.vi"("GPIB Address"=w952) -> ("Error Out"=w953:errorcluster, "GPIB Address Out"=w954:string)  [unwired: 9 in]
              }
              frame #1 {
                n501 = local read "current y"() -> (w962:i32)
                n502 = local read "current x"() -> (w964:i32)
                n503 = local read "y target"() -> (w963:i32)
                n504 = local read "x target"() -> (w965:i32)
                n505 = local write "Status"("Moving Probe" ("Status")) -> ()
                n506 = Subtract(x=w963, y=w962) -> (x-y=w960:i32)
                n507 = Subtract(x=w965, y=w964) -> (x-y=w961:i32)
                n508 = call "EG2001 Move Machine Step X-Y.vi"("Flip X Coordinates?"=FALSE, "Y"=w960, "Steps/Microns"=enum32{"Steps", "Microns"}."Microns", "X"=w961, "error in (no error)"=w958, "GPIB Address"=w959) -> ()  [unwired: 4 in, 2 out]
              }
              frame #2 {
                n509 = local read "y target"() -> (w967:i32)
                n510 = local read "x target"() -> (w968:i32)
                n511 = local write "Status"("Done" ("Status")) -> ()
                n512 = local write "current x"(w968) -> ()
                n513 = local write "current y"(w967) -> ()
              }
            }
          }
          frame "manual test" {
            # "Manual Test execution - first runs sweep VI, then measures the two points for the raw test. It doesn NOT save anywhere automatically, just displays results on the graph"
            n514 = Enqueue Element At Opposite End(queue=w972, element="idle", error in (no error)=w975) -> (queue out=w973:refnum<queue>, error out=w974:errorcluster)  [unwired: 1 in, 1 out]
            n515 = flat-sequence {
              tunnel: [w985] -> w983
              tunnel: [w984] -> w982
              tunnel: [w992] -> w981
              tunnel: w983 -> [w992]
              tunnel: [w991] -> w980
              tunnel: w982 -> [w991]
              tunnel: [w1016] -> w979
              tunnel: w981 -> [w1016]
              tunnel: [w1015] -> w978
              tunnel: w980 -> [w1015]
              tunnel: ["Measure 2 Point?"] -> w970
              tunnel: [w1047] -> w977
              tunnel: w979 -> [w1047]
              tunnel: [w1046] -> w976
              tunnel: w978 -> [w1046]
              tunnel: w970 -> [w1045]
              tunnel: [w1045] -> w969
              tunnel: w977 -> [w1083]
              tunnel: w976 -> [w1082]
              tunnel: w969 -> [w1076]
              frame #0 {
                n516 = local read "Prober GPIB"() -> (w986:string)
                n517 = call "EG2001 Move Z Up.vi"("GPIB Address"=w986) -> ("Error Out"=w984:errorcluster, "GPIB Address Out"=w985:string)  [unwired: 1 in, 8 out]
              }
              frame #1 {
                n518 = local read "Channel"() -> (w1001:enum32{"Channel A", "Channel B"})
                n519 = local read "I compliance sweep"() -> (w996:dbl)
                n520 = local read "sweep delay ms"() -> (w995:dbl)
                n521 = local read "Sweep Settings"() -> (w1002:T10)
                n522 = local write "Status"("Sweeping IV Curve") -> ()
                n523 = local read "V start"() -> (w1000:dbl)
                n524 = local read "points"() -> (w998:u16)
                n525 = local read "V end"() -> (w999:dbl)
                n526 = local read "NPLC"() -> (w997:dbl)
                n527 = Bundle By Name(cluster=w1002, "Channel"=w1001, "Vstart"=w1000, "Vend"=w999, "# of points"=w998, "NPLC"=w997, "I compliance"=w996, "Delay ms"=w995) -> (w987:T10)
                n528 = local read "Keysight"() -> (w988:bool)
                n529 = local write "Sweep Settings"(w987) -> ()
                n530 = local read "4-wire"() -> (w989:bool)
                n531 = case shown="False" w988 {
                  tunnel: w987 -> [w1008 w1013]
                  tunnel: [w1005 w1012] -> w994
                  tunnel: [w1004 w1011] -> w993
                  tunnel: w989 -> [w1007 w1009]
                  frame False {
                    n532 = local read "Keysight SMU"() -> (w1006:refnum<visa-resource-name>)
                    n533 = call "IVSweep (SubVI).vi"("SweepSettings"=w1008, "4 wire"=w1007, "VISA Refnum in"=w1006, "Sweep Direction (0: Up)"="Sweep Direction (Keysight)") -> ("V"=w1004:dbl[], "I"=w1005:dbl[])  [unwired: 2 out]
                  }
                  frame True {
                    n534 = local read "Keithley SMU"() -> (w1010:refnum<visa-resource-name>)
                    n535 = call "K2602 Vsweep.vi"("4-wire"=w1009, "Settings"=w1013, "SMU"=w1010) -> ("V"=w1011:dbl[], "I"=w1012:dbl[])  [unwired: 6 in, 1 out]
                  }
                }
                "Varray manual" <- w993
                "Iarray manual" <- w994
              }
              frame #2 {
                n536 = case shown="True" "Measure 2 Point?" {
                  frame False {
                    n537 = local read "Iarray manual"() -> (w1018:dbl[])
                    n538 = Array Max & Min(array=w1018) -> (min value=w1017:dbl)  [unwired: 3 out]
                    n539 = local write "Imeas manual"(w1017) -> ()
                  }
                  frame True {
                    n540 = local read "Keysight"() -> (w1019:bool)
                    n541 = case shown="False" w1019 {
                      tunnel: [w1021 w1043] -> w1020
                      frame False {
                        n542 = local read "Channel Keysight"() -> (w1024:dbl)
                        n543 = local read "Repeat Id"() -> (w1028:u32)
                        n544 = local read "Imeas Settings"() -> (w1032:T11)
                        n545 = local read "I compliance"() -> (w1029:dbl)
                        n546 = local read "Id delay ms"() -> (w1027:dbl)
                        n547 = local write "Status"("Measuring I @ Vset") -> ()
                        n548 = local read "4-wire"() -> (w1025:bool)
                        n549 = local read "NPLC"() -> (w1030:dbl)
                        n550 = local read "V set"() -> (w1031:dbl)
                        n551 = Bundle By Name(cluster=w1032, "Channel"=w1024, "Vset"=w1031, "NPLC"=w1030, "I compliance"=w1029, "Repeat time"=w1028, "Delay ms"=w1027, "4-wire"=w1025) -> (w1023:T11)
                        n552 = local read "Keysight SMU"() -> (w1022:refnum<visa-resource-name>)
                        n553 = local write "Imeas Settings"(w1023) -> ()
                        n554 = call "Agilent B2900 Measure I at Vset.vi"("Imeas Settings"=w1023, "VISA resource name"=w1022) -> ("Avg I"=w1021:dbl)  [unwired: 9 in]
                      }
                      frame True {
                        n555 = local read "Id delay ms"() -> (w1037:dbl)
                        n556 = local read "Repeat Id"() -> (w1038:u32)
                        n557 = local read "Channel"() -> (w1042:enum32{"Channel A", "Channel B"})
                        n558 = local read "Imeas Settings"() -> (w1044:T11)
                        n559 = local read "I compliance"() -> (w1039:dbl)
                        n560 = local read "4-wire"() -> (w1035:bool)
                        n561 = local write "Status"("Measuring I @ Vset") -> ()
                        n562 = local read "NPLC"() -> (w1040:dbl)
                        n563 = local read "V set"() -> (w1041:dbl)
                        n564 = Bundle By Name(cluster=w1044, "Channel"=w1042, "Vset"=w1041, "NPLC"=w1040, "I compliance"=w1039, "Repeat time"=w1038, "Delay ms"=w1037, "4-wire"=w1035) -> (w1034:T11)
                        n565 = local read "Keithley SMU"() -> (w1033:refnum<visa-resource-name>)
                        n566 = local write "Imeas Settings"(w1034) -> ()
                        n567 = call "K2602 setVmeasI.vi"("Settings"=w1034, "SMU"=w1033) -> ("Iavg"=w1043:dbl)  [unwired: 6 in, 3 out]
                      }
                    }
                    n568 = local write "Imeas manual"(w1020) -> ()
                  }
                }
              }
              frame #3 {
                n569 = case shown="True" w1045 {
                  frame False {
                    n570 = local read "Varray manual"() -> (w1048:dbl[])
                    n571 = Array Max & Min(array=w1048) -> (min value=w1049:dbl)  [unwired: 3 out]
                    n572 = local write "Vmeas manual"(w1049) -> ()
                  }
                  frame True {
                    n573 = local read "Keysight"() -> (w1050:bool)
                    n574 = case shown="False" w1050 {
                      tunnel: [w1052 w1065] -> w1051
                      frame False {
                        n575 = local read "Vf delay ms"() -> (w1057:dbl)
                        n576 = local read "Repeat Vf"() -> (w1058:u32)
                        n577 = local read "Channel"() -> (w1062:enum32{"Channel A", "Channel B"})
                        n578 = local read "Vmeas Settings"() -> (w1063:T11)
                        n579 = local read "V compliance"() -> (w1059:dbl)
                        n580 = local read "4-wire"() -> (w1055:bool)
                        n581 = local write "Status"("Measuring V @ Iset") -> ()
                        n582 = local read "NPLC"() -> (w1060:dbl)
                        n583 = local read "I set"() -> (w1061:dbl)
                        n584 = Bundle By Name(cluster=w1063, "Channel"=w1062, "Vset"=w1061, "NPLC"=w1060, "I compliance"=w1059, "Repeat time"=w1058, "Delay ms"=w1057, "4-wire"=w1055) -> (w1054:T11)
                        n585 = local read "Keysight SMU"() -> (w1053:refnum<visa-resource-name>)
                        n586 = local write "Vmeas Settings"(w1054) -> ()
                        n587 = call "Agilent B2900 Measure V at Iset.vi"("Imeas Settings"=w1054, "VISA resource name"=w1053) -> ("Avg V"=w1052:dbl)  [unwired: 9 in]
                      }
                      frame True {
                        n588 = local read "Vf delay ms"() -> (w1069:dbl)
                        n589 = local read "Repeat Vf"() -> (w1070:u32)
                        n590 = local read "Channel"() -> (w1074:enum32{"Channel A", "Channel B"})
                        n591 = local read "Vmeas Settings"() -> (w1075:T11)
                        n592 = local read "V compliance"() -> (w1071:dbl)
                        n593 = local read "4-wire"() -> (w1067:bool)
                        n594 = local write "Status"("Measuring V @ Iset") -> ()
                        n595 = local read "NPLC"() -> (w1072:dbl)
                        n596 = local read "I set"() -> (w1073:dbl)
                        n597 = Bundle By Name(cluster=w1075, "Channel"=w1074, "Vset"=w1073, "NPLC"=w1072, "I compliance"=w1071, "Repeat time"=w1070, "Delay ms"=w1069, "4-wire"=w1067) -> (w1066:T11)
                        n598 = local read "Keithley SMU"() -> (w1064:refnum<visa-resource-name>)
                        n599 = call "K2602 setImeasV.vi"("Settings"=w1066, "SMU"=w1064) -> ("Vavg"=w1065:dbl)  [unwired: 6 in, 3 out]
                        n600 = local write "Vmeas Settings"(w1066) -> ()
                      }
                    }
                    n601 = local write "Vmeas manual"(w1051) -> ()
                  }
                }
              }
              frame #4 {
                n602 = call "EG2001 Move Z Down.vi"("error in (no error)"=w1082, "GPIB Address"=w1083) -> ()  [unwired: 8 in, 2 out]
                n603 = local write "Status"("Done") -> ()
                n604 = case shown="True" w1076 {
                  tunnel: [w1088 w1103] -> w1081
                  tunnel: [w1086 w1102] -> w1078
                  tunnel: [w1087 w1101] -> w1077
                  frame False {
                    n605 = local read "Manual IV Plot settting"() -> (w1088:enum32{"Linear plot", "Log plot"})
                    n606 = local read "Vmeas manual"() -> (w1091:dbl)
                    n607 = local read "Varray manual"() -> (w1092:dbl[])
                    n608 = local read "Imeas manual"() -> (w1090:dbl)
                    n609 = local read "Iarray manual"() -> (w1085:dbl[])
                    n610 = local read "points"() -> (w1093:u16)
                    n611 = local read "V set"() -> (w1089:dbl)
                    n612 = Array Max & Min(array=w1085) -> (min value=w1084:dbl)  [unwired: 3 out]
                    n613 = call "get Plot.vi"("I set"=w1084, "Imeas"=w1090, "V set"=w1089, "Vmeas"=w1091, "Iarray"=w1085, "Varray"=w1092, "points"=w1093) -> ("logplot"=w1086:cluster{"Varray manual":dbl[], dbl[]}[], "Linearplot"=w1087:T18)  [unwired: 3 in]
                  }
                  frame True {
                    n614 = local read "Manual IV Plot settting"() -> (w1103:enum32{"Linear plot", "Log plot"})
                    n615 = local read "Vmeas manual"() -> (w1097:dbl)
                    n616 = local read "Varray manual"() -> (w1099:dbl[])
                    n617 = local read "Imeas manual"() -> (w1096:dbl)
                    n618 = local read "Iarray manual"() -> (w1098:dbl[])
                    n619 = local read "points"() -> (w1100:u16)
                    n620 = local read "V set"() -> (w1095:dbl)
                    n621 = local read "I set"() -> (w1094:dbl)
                    n622 = call "get Plot.vi"("I set"=w1094, "Imeas"=w1096, "V set"=w1095, "Vmeas"=w1097, "Iarray"=w1098, "Varray"=w1099, "points"=w1100) -> ("logplot"=w1102:cluster{"Varray manual":dbl[], dbl[]}[], "Linearplot"=w1101:T18)  [unwired: 3 in]
                  }
                }
                "Manual Plot 0" <- w1077
                "Manaul Plot 1" <- w1078
                n623 = case shown="\"Linear plot\", Default" w1081 {
                  tunnel: w1077 -> [w1106 _]
                  tunnel: [w1106 w1109] -> w1080
                  tunnel: w1078 -> [_ w1109]
                  frame "Linear plot", Default {
                    n624 = property on="Manual IV" class="XYGraph (strict)"("YScale.Mapping Mode"=u8 0 ("Y Scale.Mapping Mode")) -> ()  [unwired: 2 in, 2 out]
                    n625 = property on="Manual IV" class="XYGraph (strict)"("YScale.NameLbl.Text"="Current (A)" ("X Scale.Name Label.Text")) -> ()  [unwired: 2 in, 2 out]
                  }
                  frame "Log plot" {
                    n626 = property on="Manual IV" class="XYGraph (strict)"("YScale.NameLbl.Text"="Abs(I)" ("Y Scale.Name Label.Text")) -> ()  [unwired: 2 in, 2 out]
                    n627 = property on="Manual IV" class="XYGraph (strict)"("YScale.Mapping Mode"=u8 1 ("Y Scale.Mapping Mode")) -> ()  [unwired: 2 in, 2 out]
                  }
                }
                "Manual IV" <- w1080
              }
              frame #5 {
                n628 = Two Button Dialog(message="Save Data?", 1:"Nay" ("F button name (\"Cancel\")"), 2:"Yea" ("T button name (\"OK\")")) -> (T button?=w1113:bool)
                n629 = case shown="True" w1113 {
                  frame False {
                  }
                  frame True {
                    n630 = flat-sequence {
                      tunnel: [w1119] -> w1115
                      tunnel: w1115 -> [w1142]
                      tunnel: [w1142] -> w1114
                      tunnel: w1114 -> [w1160]
                      frame #0 {
                        n631 = local read "Wafer Info 3"() -> (w1118:T2)
                        n632 = Bundle By Name(cluster=w1118, "Comment"="Manual Test Comments") -> (w1117:T2)
                        n633 = local write "Wafer Info 3"(w1117) -> ()
                      }
                      frame #1 {
                        n634 = local read "FineTest save path"() -> (w1126:path)
                        n635 = local read "Lot"() -> (w1127:string)
                        n636 = Build Path(base path=w1126, name or relative path=w1127) -> (appended path=w1128:path)
                        n637 = local read "Wafer Name"() -> (w1129:string)
                        n638 = call "CreateDirectory.vi"("Path to be created"=w1128) -> ()  [unwired: 10 in, 1 out]
                        n639 = Build Path(base path=w1128, name or relative path=w1129) -> (appended path=w1130:path)
                        n640 = local read "Output Power (mW)"() -> (w1121:dbl)
                        n641 = call "CreateDirectory.vi"("Path to be created"=w1130) -> ()  [unwired: 10 in, 1 out]
                        n642 = local read "Device Name"() -> (w1120:string)
                        n643 = Build Path(base path=w1130, name or relative path="IV") -> (appended path=w1132:path)
                        n644 = call "CreateDirectory.vi"("Path to be created"=w1132) -> ()  [unwired: 10 in, 1 out]
                        n645 = Number To Decimal String(number=w1121) -> (decimal integer string=w1123:string)  [unwired: 1 in]
                        n646 = Build Path(base path=w1132, name or relative path=w1120) -> (appended path=w1122:path)
                        n647 = call "CreateDirectory.vi"("Path to be created"=w1122) -> ()  [unwired: 10 in, 1 out]
                        n648 = Concatenate Strings(w1123, " mW" ("string")) -> (w1125:string)
                        n649 = Build Path(base path=w1122, name or relative path=w1125) -> (appended path=w1119:path)
                        n650 = call "CreateDirectory.vi"("Path to be created"=w1119) -> ()  [unwired: 10 in, 1 out]
                      }
                      frame #2 {
                        n651 = local read "I compliance sweep"() -> (w1137:dbl)
                        n652 = local read "sweep delay ms"() -> (w1136:dbl)
                        n653 = local read "Sweep Direction (Keysight)"() -> (w1141:i32)
                        n654 = local read "points"() -> (w1138:u16)
                        n655 = local read "V end"() -> (w1139:dbl)
                        n656 = local read "V start"() -> (w1140:dbl)
                        n657 = call "pho_DBCheck_LIV_meas_recipe.vi"("V start"=w1140, "Sweep Direction (Keysight)"=w1141, "V end"=w1139, "points"=w1138, "I compliance sweep"=w1137, "sweep delay ms"=w1136) -> ("RecipeID"=w1135:string)  [unwired: 8 in, 1 out]
                        n658 = local write "RecipeID"(w1135) -> ()
                        n659 = Equal?(x=w1135, y="") -> (x = y?=w1133:bool)
                        n660 = case shown="True" w1133 {
                          frame False {
                          }
                          frame True {
                            n661 = local read "I compliance sweep"() -> (w1145:dbl)
                            n662 = local read "sweep delay ms"() -> (w1144:dbl)
                            n663 = local read "Sweep Direction (Keysight)"() -> (w1149:i32)
                            n664 = local read "points"() -> (w1146:u16)
                            n665 = local read "V end"() -> (w1147:dbl)
                            n666 = local read "V start"() -> (w1148:dbl)
                            n667 = call "pho_DB_Insert_LIV_meas_recipe.vi"("V start"=w1148, "Sweep Direction (Keysight)"=w1149, "V end"=w1147, "points"=w1146, "I compliance sweep"=w1145, "sweep delay ms"=w1144) -> ("RecipeID"=w1143:string)  [unwired: 9 in]
                            n668 = local write "RecipeID"(w1143) -> ()
                          }
                        }
                      }
                      frame #3 {
                        n669 = local read "current y"() -> (w1166:i32)
                        n670 = local read "current x"() -> (w1165:i32)
                        n671 = local read "Current Session"() -> (w1150:timestamp)
                        n672 = local read "Temp Data"() -> (w1154:T1)
                        n673 = local read "Device Name"() -> (w1162:string)
                        n674 = local read "Wafer Name"() -> (w1161:string)
                        n675 = local read "Varray manual"() -> (w1168:dbl[])
                        n676 = local read "Iarray manual"() -> (w1167:dbl[])
                        n677 = local read "Operator"() -> (w1151:string)
                        n678 = To Double Precision Float(number=w1165) -> (double precision float=w1163:dbl)
                        n679 = To Double Precision Float(number=w1166) -> (double precision float=w1164:dbl)
                        n680 = Get Date/Time In Seconds() -> (seconds since 1Jan1904=w1173:timestamp)
                        n681 = local read "Parameters Flash"() -> (w1156:T4)
                        n682 = local read "RecipeID"() -> (w1155:string)
                        n683 = local read "Wafer Info 3"() -> (w1153:T2)
                        n684 = call "get Flash FileName .vi"("Time"=w1173, "Device Name"=w1162, "Operator"=w1151, "Wafer Name"=w1161, "FineTest save path"=w1160) -> ("appended path"=w1157:path)  [unwired: 6 in]
                        n685 = Build Array(w1168, w1167) -> (w1159:dbl[][])
                        n686 = Bundle(w1163, w1164) -> (w1152:cluster{dbl, dbl})  [unwired: 1 in]
                        n687 = Get Date/Time String(seconds (now)=w1173, want seconds? (F)=TRUE) -> (date string=w1169:string, time string=w1171:string)  [unwired: 1 in]
                        n688 = local read "Mask"() -> (w1158:string)
                        n689 = call <vilib>:"Space Constant.vi"() -> ("String"=w1172:string)
                        n690 = Concatenate Strings(w1169, w1172, w1171) -> ()  [unwired: 1 out]
                        n691 = call "WriteFlashFile NEW.vi"("Input File Path"=w1157, "IV array"=w1159, "Current Session"=w1150, "Parameters"=w1156, "RecipeID"=w1155, "User"=w1151, "Coords"=w1152, "Wafer Info"=w1153, "Mask Name"=w1158, "Temp Data"=w1154) -> ()  [unwired: 17 in, 1 out]
                      }
                    }
                  }
                }
              }
            }
          }
          frame "generate prelim report" {
            n692 = call <vilib>:"System Exec.vi"("wait until completion? (T)"=FALSE, "working directory"=path "C:/Users/Flash/Documents/GitHub/solarjunction", "command line"="C:\\Windows\\system32\\cmd.exe /k python3 generate_prelim_report.py") -> ()  [unwired: 5 in, 4 out]
          }
          frame "update wafer" {
            # "Takes wafer name and pulls info from the database, and updates relevant variables"
            n693 = local read "Wafer Name"() -> (w1181:string)
            n694 = Enqueue Element At Opposite End(queue=w1189, element="idle", error in (no error)=w1183) -> (queue out=w1188:refnum<queue>, error out=w1187:errorcluster)  [unwired: 1 in, 1 out]
            n695 = call "getDB Wafer Info.vi"("Wafer Name"=w1181) -> ("WaferInfo"=w1182:T19)  [unwired: 9 in, 1 out]
            n696 = Unbundle By Name(w1182) -> ("WaferName"=w1179:string, "Scribe"=w1186:string, "Lot"=w1185:string, "Mask"=w1184:string)  [unwired: 1 out]
            n697 = local write "Scribe"(w1186) -> ()
            n698 = local write "Lot"(w1185) -> ()
            n699 = local write "Mask"(w1184) -> ()
            n700 = Equal?(x=w1181, y=w1179) -> (x = y?=w1180:bool)
            n701 = case shown="True" w1180 {
              tunnel: w1179 -> [w1191 _]
              frame False {
                n702 = local write "Wafer Name"(w1191) -> ()
              }
              frame True {
              }
            }
          }
          frame "desired wafer to current wafer" {
            # "This only runs in the lot test. It updates the wafer name from the wafer list. The Wafer counter keeps track of the iteration of the auto test the lot test is currently on. Once the wafer name is updated, the Wafer counter in incremented by one. If the Wafer list has reached its end, the wafer counter is returned to 0"
            n703 = flat-sequence {
              frame #0 {
                n704 = local read "WaferCounter"() -> (w1196:i32)
                n705 = property on="Wafer List" class="LstBox (strict)"() -> ("Item Names"=w1195:string[])  [unwired: 2 in, 2 out]
                n706 = Index Array(array=w1195, index=w1196) -> (element=w1194:string)
                n707 = local write "Wafer Name"(w1194) -> ()
              }
              frame #1 {
                n708 = local read "WaferCounter"() -> (w1198:i32)
                n709 = Increment(x=w1198) -> (x+1=w1197:i32)
                n710 = local write "WaferCounter"(w1197) -> ()
              }
              frame #2 {
                n711 = property on="Wafer List" class="LstBox (strict)"() -> ("Item Names"=w1202:string[])  [unwired: 2 in, 2 out]
                n712 = local read "WaferCounter"() -> (w1200:i32)
                n713 = Array Size(array=w1202) -> (size(s)=w1201:i32)
                n714 = Equal?(x=w1201, y=w1200) -> (x = y?=w1199:bool)
                n715 = case shown="True" w1199 {
                  frame False {
                  }
                  frame True {
                    n716 = local write "WaferCounter"(0 ("WaferCounter")) -> ()
                  }
                }
              }
            }
          }
          frame "idle" {
            n717 = local write "Status"("idle" ("Status")) -> ()
          }
          frame "change plot" {
            # "Switch from linear to logarithmic plot and back on the maual test tab"
            n718 = local read "Manual IV Plot settting"() -> (w1213:enum32{"Linear plot", "Log plot"})
            n719 = Enqueue Element At Opposite End(queue=w1208, element="idle", error in (no error)=w1210) -> (queue out=w1207:refnum<queue>, error out=w1209:errorcluster)  [unwired: 1 in, 1 out]
            n720 = case shown="\"Log plot\"" w1213 {
              tunnel: [w1216 w1219] -> w1212
              frame "Linear plot", Default {
                n721 = property on="Manual IV" class="XYGraph (strict)"("YScale.Mapping Mode"=u8 0 ("Y Scale.Mapping Mode")) -> ()  [unwired: 2 in, 2 out]
                n722 = local read "Manual Plot 0"() -> (w1216:cluster{"V manual":dbl[], "I manual":dbl[]}[])
                n723 = property on="Manual IV" class="XYGraph (strict)"("YScale.NameLbl.Text"="Current (A)" ("Y Scale.Name Label.Text")) -> ()  [unwired: 2 in, 2 out]
              }
              frame "Log plot" {
                n724 = property on="Manual IV" class="XYGraph (strict)"("YScale.Mapping Mode"=u8 1 ("Y Scale.Mapping Mode")) -> ()  [unwired: 2 in, 2 out]
                n725 = property on="Manual IV" class="XYGraph (strict)"("YScale.NameLbl.Text"="Abs(I)" ("Y Scale.Name Label.Text")) -> ()  [unwired: 2 in, 2 out]
                n726 = local read "Manaul Plot 1"() -> (w1219:cluster{"V manual":dbl[], dbl[]}[])
              }
            }
            n727 = local write "Manual IV"(w1212) -> ()
          }
          frame "select" {
            # "Selects Best ten devices (in seperate VI). If less than ten devices are within the voltage and current bounds, it selects all the devices that are within the parameters. If no devices are in the parameters, it still saves the mask file but it will be empty"
            n728 = Enqueue Element At Opposite End(queue=w1223, element="idle", error in (no error)=w1222) -> (queue out=w1225:refnum<queue>, error out=w1224:errorcluster)  [unwired: 1 in, 1 out]
            n729 = local read "Raw Test Skipped"() -> (w1221:bool)
            n730 = Not(x=w1221) -> (.not. x?=w1220:bool)
            n731 = case shown="True" w1220 {
              frame False {
              }
              frame True {
                n732 = local read "I meas"() -> (w1229:dbl[])
                n733 = Array Size(array=w1229) -> (size(s)=w1227:i32)
                n734 = Greater Than 0?(x=w1227) -> (x > 0?=w1228:bool)
                n735 = case shown="True" w1228 {
                  tunnel: w1227 -> [_ w1247]
                  frame False {
                  }
                  frame True {
                    n736 = local read "Laser Current (mA)"() -> (w1232:dbl)
                    n737 = local read "Number Select"() -> (w1253:u16)
                    n738 = local read "new raw data save path"() -> (w1249:path)
                    n739 = local read "V meas"() -> (w1239:dbl[])
                    n740 = local read "I meas"() -> (w1238:dbl[])
                    n741 = local read "Vmax"() -> (w1252:dbl)
                    n742 = local read "Vmin"() -> (w1251:dbl)
                    n743 = Greater Than 0?(x=w1232) -> (x > 0?=w1231:bool)
                    n744 = local read "Mask File Raw"() -> (w1254:path)
                    n745 = local read "RawData file"() -> (w1235:path)
                    n746 = local read "Wafer Name"() -> (w1255:string)
                    n747 = Initialize Array(nan ("element"), w1247) -> (w1243:dbl[])
                    n748 = call "select RawTestData.vi"("Light > 0?"=w1231, "Number Select"=w1253, "Vmax"=w1252, "Vmin"=w1251, "V meas"=w1239, "I meas"=w1238) -> ("Selected V"=w1246:dbl[], "Selected I"=w1244:dbl[], "Selected Index"=w1233:dbl[])  [unwired: 2 in, 1 out]
                    n749 = call "updatedFile RawTestSelect.vi"("Column Number"=u32 21, "Selected Index"=w1233, "Path"=w1235) -> ()  [unwired: 9 in]
                    n750 = Replace Array Subset(array=w1243, new element=w1246, index=0) -> (w1241:dbl[])
                    n751 = Replace Array Subset(array=w1243, new element=w1244, index=0) -> (w1240:dbl[])
                    n752 = call "save FineMask.vi"("Selected Index"=w1233, "RawData Save Path"=w1249, "Text Add"=w1255, "Mask File Raw"=w1254) -> ("Output path"=w1250:path)  [unwired: 7 in]
                    n753 = Bundle("V meas"=w1239, "I meas"=w1238) -> (w1237:cluster{"V meas":dbl[], "I meas":dbl[]})  [unwired: 1 in]
                    n754 = Bundle(w1241, w1240) -> (w1230:cluster{dbl[], dbl[]})  [unwired: 1 in]
                    n755 = local write "Mask File Fine"(w1250) -> ()
                    n756 = Build Array(w1237, w1230) -> (w1236:cluster{"V meas":dbl[], "I meas":dbl[]}[])
                    n757 = local write "Spec Plot"(w1236) -> ()
                  }
                }
              }
            }
          }
          frame "update measurement log" {
            # "Collects measurement parameters (such a test type) and saves them to the measurement log CSV file."
            n758 = flat-sequence {
              tunnel: [w1267] -> w1257
              tunnel: w1257 -> [w1283]
              tunnel: [w1274] -> w1256
              tunnel: w1256 -> [w1295]
              frame #0 {
                n759 = Get Date/Time In Seconds() -> (seconds since 1Jan1904=w1269:timestamp)
                n760 = Get Date/Time String(seconds (now)=w1269) -> (date string=w1263:string, time string=w1268:string)  [unwired: 2 in]
                n761 = local read "Wafer Name"() -> (w1271:string)
                n762 = local read "Test Type"() -> (w1260:string)
                n763 = local read "Operator"() -> (w1270:string)
                n764 = Search and Replace String(replace all?=TRUE ("replace all? (F)"), input string=w1263, search string="/", replace string="_" ("replace string (\"\")")) -> (result string=w1262:string)  [unwired: 4 in, 3 out]
                n765 = Bundle("result string"=w1262, "time string"=w1268, "Wafer Name"=w1271, "Operator"=w1270, "Test description"="Test description", "Test Type"=w1260) -> (w1267:T15)  [unwired: 1 in]
                "Last Measurement" <- w1267
              }
              frame #1 {
                w1272 = ","
                n766 = Unbundle(w1283) -> ("result string"=w1279:string, "time string"=w1278:string, "Wafer Name"=w1277:string, "Operator"=w1276:string, "Test description"=w1275:string, "Test Type"=w1273:string)
                n767 = Concatenate Strings(w1279, w1272, w1278, w1272, w1277, w1272, w1276, w1272, w1275, w1272, w1273) -> (w1280:string)
                n768 = call <vilib>:"Check if File or Folder Exists.vi"("path"=path "C:/Users/Flash/Desktop/Data/Detector test data/MeasurementLog.csv") -> ("file or folder exists?"=w1281:bool, "dup path"=w1274:path)  [unwired: 1 in, 8 out]
                n769 = case shown="True" w1281 {
                  tunnel: w1274 -> [w1288 w1293]
                  tunnel: w1280 -> [w1285 w1290]
                  frame False {
                    n770 = Build Array(w1285) -> (w1284:string[])
                    n771 = call-poly <vilib>:"Write To Spreadsheet File.vi"("delimiter (\\t)"="," ("delimiter (\\t)"), "append to file? (new file:F)"=FALSE, "1D data"=w1284, "file path (dialog if empty)"=w1288) -> ()  [unwired: 4 in, 1 out]
                  }
                  frame True {
                    n772 = Build Array(w1290) -> (w1289:string[])
                    n773 = call-poly <vilib>:"Write To Spreadsheet File.vi"("delimiter (\\t)"="," ("delimiter (\\t)"), "append to file? (new file:F)"=TRUE, "1D data"=w1289, "file path (dialog if empty)"=w1293) -> ()  [unwired: 4 in, 1 out]
                  }
                }
              }
              frame #2 {
                n774 = call-poly <vilib>:"Read From Spreadsheet File.vi"("file path (dialog if empty)"=w1295) -> ("all rows"=w1294:string[][])  [unwired: 6 in, 4 out]
                n775 = property on="Logview" class="MCListbox (strict)"("ItemNames"=w1294) -> ()  [unwired: 2 in, 2 out]
              }
            }
          }
          frame "load raw data" {
            # "Prompts the user to pick a raw data file, and then displays that data on the graphical display  on the raw test tab"
            n776 = local read "RawData Save Path"() -> (w1296:path)
            n777 = Enqueue Element At Opposite End(queue=w1302, element="idle", error in (no error)=w1301) -> (queue out=w1304:refnum<queue>, error out=w1303:errorcluster)  [unwired: 1 in, 1 out]
            n778 = call "File Dialog"("start path"=w1296, "prompt"="Please pick a raw test data file", "pattern (all files)"="*.csv" ("pattern label")) -> ("selected path"=w1297:path, "cancelled"=w1300:bool)  [unwired: 9 in, 2 out]
            n779 = case shown="False" w1300 {
              tunnel: w1297 -> [_ w1307]
              frame True {
              }
              frame False {
                n780 = Strip Path(path=w1307) -> (name=w1308:string)  [unwired: 1 out]
                n781 = Strip Path(path=w1307) -> (stripped path=w1306:path)  [unwired: 1 out]
                n782 = local write "RawData file"(w1307) -> ()
                n783 = call "read Raw.vi"("Path"=w1307) -> ("Session Info"=w1326:T20, "Die Info"=w1335:T21, "Wafer Info"=w1334:T9, "V"=w1312:dbl[], "I"=w1311:dbl[])  [unwired: 6 in]
                n784 = local write "Test FileName"(w1308) -> ()
                n785 = local write "new raw data save path"(w1306) -> ()
                n786 = local write "I meas"(w1311) -> ()
                n787 = Unbundle By Name(w1326) -> ("V set"=w1325:dbl, "I compliance"=w1324:dbl, "J set"=w1323:dbl, "I set"=w1322:dbl, "V compliance"=w1321:dbl, "Laser Power (mW)"=w1319:dbl, "Operator"=w1320:string)
                n788 = local write "V meas"(w1312) -> ()
                n789 = Unbundle By Name(w1335) -> ("Device Name"=w1329:string, "ActiveArea_um2"=w1328:dbl, "MesaArea_um2"=w1327:dbl)
                n790 = Unbundle By Name(w1334) -> ("Wafer Name"=w1333:string, "Scribe"=w1332:string, "Mask"=w1331:string, "Lot"=w1330:string)
                n791 = Array Size(array=w1311) -> (size(s)=w1317:i32)
                n792 = call <vilib>:"Histogram.vi"("X"=w1312) -> ("Histogram Graph"=w1309:T14)  [unwired: 7 in, 3 out]
                n793 = call <vilib>:"Histogram.vi"("X"=w1311) -> ("Histogram Graph"=w1310:T14)  [unwired: 7 in, 3 out]
                n794 = local write "Scribe"(w1332) -> ()
                n795 = local write "Mask"(w1331) -> ()
                n796 = local write "Lot"(w1330) -> ()
                n797 = local write "Device Name"(w1329) -> ()
                n798 = local write "ActiveArea_um2"(w1328) -> ()
                n799 = local write "MesaArea_um2"(w1327) -> ()
                n800 = local write "V set"(w1325) -> ()
                n801 = local write "I set"(w1322) -> ()
                n802 = local write "Vforward hist"(w1309) -> ()
                n803 = local write "Idark hist"(w1310) -> ()
                n804 = Initialize Array(nan ("element"), w1317) -> (w1316:dbl[])
                n805 = local write "Wafer Name"(w1333) -> ()
                n806 = local write "I compliance"(w1324) -> ()
                n807 = local write "J set A/cm2"(w1323) -> ()
                n808 = local write "V compliance"(w1321) -> ()
                n809 = local write "Laser Current (mA)"(w1319) -> ()
                n810 = local write "Operator"(w1320) -> ()
                n811 = Bundle("V"=w1312, "I"=w1311) -> (w1315:cluster{"V":dbl[], "I":dbl[]})  [unwired: 1 in]
                n812 = Bundle(w1316, w1316) -> (w1314:cluster{dbl[], dbl[]})  [unwired: 1 in]
                n813 = local write "Selected Data"(w1314) -> ()
                n814 = Build Array(w1315, w1314) -> (w1313:cluster{"V":dbl[], "I":dbl[]}[])
                n815 = local write "Spec Plot"(w1313) -> ()
              }
            }
          }
          frame "start fine" {
            # "Executes Fine test. If \"no file\" is true, it means that raw test was skipped, but then no previous raw data was found to run the fine test. The fine test will be skipped in this case.\n1) Loads  the fine mask files and updates relevant parameters\n2) Passes the parameters to the data clusters. There are three data clusters due to different versions of the save flash file. It saves the wafer information, time and date, current power, temperature, and other assorted parameters. Many parameters are leftover from the solar cell testing program, and are consequently always left as 0.\n3)The sweep is run using the Keithley sweep sub VI\n4) The directory is found/created to save the IV file (see guide for saving structure)\n5) data is saved and prober is returned to 0  0"
            n816 = Enqueue Element At Opposite End(queue=w1337, element="idle", error in (no error)=w1338) -> (queue out=w1339:refnum<queue>, error out=w1340:errorcluster)  [unwired: 1 in, 1 out]
            n817 = flat-sequence {
              tunnel: w1341 -> [w1344]
              frame #0 {
                n818 = local read "no file"() -> (w1343:bool)
                n819 = Not(x=w1343) -> (.not. x?=w1342:bool)
                n820 = case shown="True" w1342 {
                  tunnel: w1344 -> [_ w1345]
                  frame False {
                  }
                  frame True {
                    n821 = flat-sequence {
                      tunnel: [w1351] -> w1346
                      tunnel: w1345 -> [w1349]
                      tunnel: w1346 -> [w1363]
                      frame #0 {
                        w1352 = u8 0 ("Progress 2")
                        n822 = local write "Progress 2"(w1352) -> ()
                        n823 = local read "points"() -> (w1354:u16)
                        n824 = case shown="True" w1349 {
                          tunnel: "Mask File Fine" -> [w1361 w1362]
                          tunnel: [w1361 w1362] -> w1347
                          frame False {
                          }
                          frame True {
                          }
                        }
                        n825 = Initialize Array(nan ("element"), w1354) -> (w1356:dbl[])
                        n826 = local write "Tab Control"(T16."Fine Test" ("Tab Control")) -> ()
                        n827 = local write "Mask File Fine"(w1347) -> ()
                        n828 = local write "Status"("prepare fine test" ("Status")) -> ()
                        n829 = Bundle(w1356, w1356) -> (w1355:cluster{dbl[], dbl[]})  [unwired: 1 in]
                        n830 = call "Device Files v1.vi"("Rows"=1200, "Mask file path"=w1347) -> ("size(s)"=w1351:i32, "Array of Cell Clusters"=→"Fine Cell Clusters":T5)  [unwired: 6 in, 2 out]
                        "Total Device" <- w1351
                        n831 = Initialize Array(w1355, w1351) -> (→"IV fine linear" →"IV fine log":cluster{dbl[], dbl[]}[])
                        "Current Device" <- w1352
                      }
                      frame #1 {
                        n832 = for {
                          N: w1363 -> [w1393]
                          i -> [w1394]
                          n833 = flat-sequence {
                            tunnel: w1394 -> [w1409]
                            tunnel: [w1417] -> w1388
                            tunnel: [w1416] -> w1387
                            tunnel: [w1413] -> w1386
                            tunnel: [w1412] -> w1385
                            tunnel: [w1411] -> w1384
                            tunnel: [w1410] -> w1383
                            tunnel: [w1409] -> w1375
                            tunnel: w1388 -> [w1432]
                            tunnel: w1387 -> [w1431]
                            tunnel: w1386 -> [w1429]
                            tunnel: w1385 -> [w1428]
                            tunnel: w1384 -> [w1427]
                            tunnel: w1383 -> [w1426]
                            tunnel: [w1425] -> w1382
                            tunnel: [w1424] -> w1381
                            tunnel: [w1423] -> w1376
                            tunnel: w1375 -> [w1423]
                            tunnel: w1382 -> [w1435]
                            tunnel: w1381 -> [w1434]
                            tunnel: [w1433] -> w1377
                            tunnel: w1376 -> [w1433]
                            tunnel: [w1447] -> w1371
                            tunnel: w1377 -> [w1447]
                            tunnel: w1371 -> [w1472]
                            tunnel: [w1472] -> w1370
                            tunnel: w1370 -> [w1487]
                            tunnel: [w1487] -> w1373
                            tunnel: [w1480] -> w1372
                            tunnel: w1373 -> [w1508]
                            tunnel: [w1499] -> w1369
                            tunnel: [w1493] -> w1368
                            tunnel: [w1492] -> w1367
                            tunnel: w1372 -> [w1491]
                            tunnel: [w1521] -> w1366
                            tunnel: [w1522] -> w1365
                            tunnel: [w1523] -> w1364
                            tunnel: w1367 -> [w1523]
                            tunnel: w1368 -> [w1522]
                            tunnel: w1369 -> [w1521]
                            tunnel: w1366 -> [w1548]
                            tunnel: w1365 -> [w1535]
                            tunnel: w1364 -> [w1542]
                            frame #0 {
                              n834 = local read "Fine Cell Clusters"() -> (w1422:T5)
                              n835 = local read "Output Power (mW)"() -> (w1399:dbl)
                              n836 = local read "ActiveArea_um2"() -> (w1401:dbl)
                              n837 = Index Array(array=w1422, index=w1409) -> (element=w1406:T22)
                              n838 = local read "Laser Current (mA)"() -> (w1405:dbl)
                              n839 = Divide(x=w1401, y=100000000.0) -> (x/y=w1396:dbl)
                              n840 = Unbundle By Name(w1406) -> ("Cell Name"=w1421:string, "X-coord"=w1411:dbl, "Y-coord"=w1410:dbl, "Area"=w1420:dbl, "Mesa Area"=w1419:dbl)
                              n841 = Multiply(x=w1399, y=0.001) -> (x*y=w1397:dbl)
                              n842 = local write "Device Name"(w1421) -> ()
                              n843 = local write "ActiveArea_um2"(w1420) -> ()
                              n844 = local write "MesaArea_um2"(w1419) -> ()
                              n845 = call "get Area.vi"("Laser"=w1405, "Cell Data Cluster"=w1406) -> ("Area"=w1407:dbl)  [unwired: 9 in]
                              n846 = Divide(x=w1397, y=w1396) -> (x/y=w1395:dbl)
                              n847 = local read "current y"() -> (w1414:i32)
                              n848 = local read "current x"() -> (w1415:i32)
                              n849 = local read "Output Power (mW)"() -> (w1402:dbl)
                              n850 = local read "Laser Current (mA)"() -> (w1403:dbl)
                              n851 = local read "Parameters Flash 2"() -> (w1408:T4)
                              n852 = Subtract(x=w1410, y=w1414) -> (x-y=w1412:dbl)
                              n853 = Subtract(x=w1411, y=w1415) -> (x-y=w1413:dbl)
                              n854 = Bundle By Name(cluster=w1408, "Cell Area (cm²)"=w1407, "Input Current (mA)"=w1403, "Power Density (W/cm^2)"=w1395, "Incident Power"=w1402) -> (w1404:T4)
                              n855 = local read "Prober GPIB"() -> (w1418:string)
                              n856 = local write "Parameters Flash"(w1404) -> ()
                              n857 = call "EG2001 Move Z Down.vi"("GPIB Address"=w1418) -> ("Error Out"=w1416:errorcluster, "GPIB Address Out"=w1417:string)  [unwired: 9 in]
                            }
                            frame #1 {
                              n858 = local write "current x"(w1427) -> ()
                              n859 = local write "current y"(w1426) -> ()
                              n860 = call "EG2001 Move Machine Step X-Y.vi"("Y"=w1428, "Steps/Microns"=enum32{"Steps", "Microns"}."Microns", "X"=w1429, "error in (no error)"=w1431, "GPIB Address"=w1432) -> ("Error Out"=w1424:errorcluster, "GPIB Address Out"=w1425:string)  [unwired: 5 in]
                            }
                            frame #2 {
                              n861 = call "EG2001 Move Z Up.vi"("error in (no error)"=w1434, "GPIB Address"=w1435) -> ()  [unwired: 10 out]
                            }
                            frame #3 {
                              n862 = local read "I compliance sweep"() -> (w1451:dbl)
                              n863 = local read "Wafer Info Flash 2"() -> (w1446:T3)
                              n864 = local read "sweep delay ms"() -> (w1450:dbl)
                              n865 = local read "Sweep Settings"() -> (w1457:T10)
                              n866 = local read "Temp Setpoint"() -> (w1442:string)
                              n867 = local read "Device Name"() -> (w1445:string)
                              n868 = local read "Channel"() -> (w1456:enum32{"Channel A", "Channel B"})
                              n869 = local read "V start"() -> (w1454:dbl)
                              n870 = local read "points"() -> (w1453:u16)
                              n871 = local read "V end"() -> (w1455:dbl)
                              n872 = local read "NPLC"() -> (w1452:dbl)
                              n873 = Bundle By Name(cluster=w1457, "Channel"=w1456, "Vstart"=w1454, "Vend"=w1455, "# of points"=w1453, "NPLC"=w1452, "I compliance"=w1451, "Delay ms"=w1450) -> (w1436:T10)
                              n874 = Bundle By Name(cluster=w1446, "Cell Name"=w1445) -> (w1444:T3)
                              n875 = Decimal String To Number(string=w1442) -> (number=w1439:i32)  [unwired: 2 in, 1 out]
                              n876 = local write "Wafer Info Flash"(w1444) -> ()
                              n877 = local write "Sweep Settings"(w1436) -> ()
                              n878 = call "DAQ Assistant"() -> ("data"=w1440:dynamicdata)  [unwired: 17 in, 2 out]
                              n879 = local read "Temp Data"() -> (w1443:T1)
                              n880 = local read "Keysight"() -> (w1438:bool)
                              n881 = local read "4-wire"() -> (w1437:bool)
                              n882 = Bundle By Name(cluster=w1443, "Ambient Temperature"=w1440, "Chuck Set Temperature"=w1439) -> (w1441:T1)
                              n883 = case shown="False" w1438 {
                                tunnel: w1436 -> [w1463 w1468]
                                tunnel: [w1460 w1467] -> w1449
                                tunnel: [w1461 w1466] -> w1448
                                tunnel: w1437 -> [w1462 w1465]
                                frame False {
                                n884 = local read "Sweep Direction (Keysight)"() -> (w1458:i32)
                                n885 = call "IVSweep (SubVI).vi"("SweepSettings"=w1463, "4 wire"=w1462, "VISA Refnum in"="Keysight SMU", "Sweep Direction (0: Up)"=w1458) -> ("V"=w1461:dbl[], "I"=w1460:dbl[])  [unwired: 2 out]
                                }
                                frame True {
                                n886 = local read "Keithley SMU"() -> (w1464:refnum<visa-resource-name>)
                                n887 = call "K2602 Vsweep.vi"("4-wire"=w1465, "Settings"=w1468, "SMU"=w1464) -> ("V"=w1466:dbl[], "I"=w1467:dbl[])  [unwired: 6 in, 1 out]
                                }
                              }
                              n888 = local write "Temp Data"(w1441) -> ()
                              n889 = local write "I fine"(w1449) -> ()
                              n890 = local write "V fine"(w1448) -> ()
                            }
                            frame #4 {
                              n891 = local read "Device Name"() -> (w1470:string)
                              n892 = local read "Wafer Info 3"() -> (w1471:T2)
                              n893 = Bundle By Name(cluster=w1471, "Cell Name (Automatic)"=w1470) -> (w1469:T2)
                              n894 = local write "Wafer Info 3"(w1469) -> ()
                            }
                            frame #5 {
                              n895 = local read "FineTest save path"() -> (w1479:path)
                              n896 = local read "Lot"() -> (w1478:string)
                              n897 = Build Path(base path=w1479, name or relative path=w1478) -> (appended path=w1477:path)
                              n898 = call "CreateDirectory.vi"("Path to be created"=w1477) -> ()  [unwired: 10 in, 1 out]
                              n899 = local read "Wafer Name"() -> (w1476:string)
                              n900 = Build Path(base path=w1477, name or relative path=w1476) -> (appended path=w1475:path)
                              n901 = call "CreateDirectory.vi"("Path to be created"=w1475) -> ()  [unwired: 10 in, 1 out]
                              n902 = Build Path(base path=w1475, name or relative path="IV") -> (appended path=w1473:path)
                              n903 = call "CreateDirectory.vi"("Path to be created"=w1473) -> ()  [unwired: 10 in, 1 out]
                              n904 = local read "Output Power (mW)"() -> (w1485:dbl)
                              n905 = local read "Device Name"() -> (w1486:string)
                              n906 = Build Path(base path=w1473, name or relative path=w1486) -> (appended path=w1484:path)
                              n907 = Number To Decimal String(number=w1485) -> (decimal integer string=w1483:string)  [unwired: 1 in]
                              n908 = call "CreateDirectory.vi"("Path to be created"=w1484) -> ()  [unwired: 10 in, 1 out]
                              n909 = Concatenate Strings(w1483, " mW" ("string")) -> (w1481:string)
                              n910 = Build Path(base path=w1484, name or relative path=w1481) -> (appended path=w1480:path)
                              n911 = call "CreateDirectory.vi"("Path to be created"=w1480) -> ()  [unwired: 10 in, 1 out]
                            }
                            frame #6 {
                              n912 = local read "Wafer Info 3"() -> (w1490:T2)
                              n913 = local read "Comments"() -> (w1489:string)
                              n914 = local read "V fine"() -> (w1498:dbl[])
                              n915 = local read "I fine"() -> (w1504:dbl[])
                              n916 = Bundle By Name(cluster=w1490, "Comment"=w1489) -> (w1488:T2)
                              n917 = Bundle("V fine"=w1498, "I fine"=w1504) -> (w1509:cluster{"V fine":dbl[], "I fine":dbl[]})  [unwired: 1 in]
                              n918 = Absolute Value(x=w1504) -> (abs(x)=w1505:dbl[])
                              n919 = local write "Wafer Info 3"(w1488) -> ()
                              n920 = local read "IV fine linear"() -> (w1511:cluster{dbl[], dbl[]}[])
                              n921 = Bundle("V fine"=w1498, w1505) -> (w1503:cluster{"V fine":dbl[], dbl[]})  [unwired: 1 in]
                              n922 = local read "IV fine log"() -> (w1506:cluster{dbl[], dbl[]}[])
                              n923 = local read "current x"() -> (w1495:i32)
                              n924 = local read "current y"() -> (w1494:i32)
                              n925 = Replace Array Subset(array=w1511, new element=w1509, index=w1508) -> (w1510:cluster{dbl[], dbl[]}[])
                              n926 = local read "Device Name"() -> (w1500:string)
                              n927 = local write "IV fine linear"(w1510) -> ()
                              n928 = local read "Wafer Name"() -> (w1502:string)
                              n929 = Replace Array Subset(array=w1506, new element=w1503, index=w1508) -> (w1507:cluster{dbl[], dbl[]}[])
                              n930 = local read "Operator"() -> (w1501:string)
                              n931 = To Double Precision Float(number=w1495) -> (double precision float=w1497:dbl)
                              n932 = To Double Precision Float(number=w1494) -> (double precision float=w1496:dbl)
                              n933 = Get Date/Time In Seconds() -> (seconds since 1Jan1904=w1492:timestamp)
                              n934 = local write "IV fine log"(w1507) -> ()
                              n935 = call "get Flash FileName .vi"("Time"=w1492, "Device Name"=w1500, "Operator"=w1501, "Wafer Name"=w1502, "FineTest save path"=w1491) -> ("appended path"=w1499:path)  [unwired: 6 in]
                              n936 = Bundle(w1497, w1496) -> (w1493:cluster{dbl, dbl})  [unwired: 1 in]
                            }
                            frame #7 {
                              n937 = local read "Sweep Direction (Keysight)"() -> (w1512:i32)
                              n938 = local read "I compliance sweep"() -> (w1516:dbl)
                              n939 = local read "sweep delay ms"() -> (w1517:dbl)
                              n940 = local read "V start"() -> (w1513:dbl)
                              n941 = local read "points"() -> (w1515:u16)
                              n942 = local read "V end"() -> (w1514:dbl)
                              n943 = call "pho_DBCheck_LIV_meas_recipe.vi"("V start"=w1513, "Sweep Direction (Keysight)"=w1512, "V end"=w1514, "points"=w1515, "I compliance sweep"=w1516, "sweep delay ms"=w1517) -> ("RecipeID"=w1518:string)  [unwired: 8 in, 1 out]
                              n944 = local write "RecipeID"(w1518) -> ()
                              n945 = Equal?(x=w1518, y="") -> (x = y?=w1520:bool)
                              n946 = case shown="True" w1520 {
                                frame False {
                                }
                                frame True {
                                n947 = local read "Sweep Direction (Keysight)"() -> (w1530:i32)
                                n948 = local read "I compliance sweep"() -> (w1526:dbl)
                                n949 = local read "sweep delay ms"() -> (w1525:dbl)
                                n950 = local read "V start"() -> (w1529:dbl)
                                n951 = local read "points"() -> (w1527:u16)
                                n952 = local read "V end"() -> (w1528:dbl)
                                n953 = call "pho_DB_Insert_LIV_meas_recipe.vi"("V start"=w1529, "Sweep Direction (Keysight)"=w1530, "V end"=w1528, "points"=w1527, "I compliance sweep"=w1526, "sweep delay ms"=w1525) -> ("RecipeID"=w1524:string)  [unwired: 9 in]
                                n954 = local write "RecipeID"(w1524) -> ()
                                }
                              }
                            }
                            frame #8 {
                              n955 = local read "V fine"() -> (w1545:dbl[])
                              n956 = local read "I fine"() -> (w1546:dbl[])
                              n957 = local read "Current Session"() -> (w1531:timestamp)
                              n958 = Build Array(w1545, w1546) -> (w1544:dbl[][])
                              n959 = Get Date/Time String(seconds (now)=w1542, want seconds? (F)=TRUE) -> (date string=w1541:string, time string=w1539:string)  [unwired: 1 in]
                              n960 = local read "Parameters Flash"() -> (w1543:T4)
                              n961 = local read "Temp Data"() -> (w1536:T1)
                              n962 = local read "Operator"() -> (w1532:string)
                              n963 = local read "RecipeID"() -> (w1533:string)
                              n964 = local read "Mask"() -> (w1547:string)
                              n965 = call <vilib>:"Space Constant.vi"() -> ("String"=w1538:string)
                              n966 = Concatenate Strings(w1541, w1538, w1539) -> (w1537:string)
                              n967 = call "WriteFlashFile NEW.vi"("Input File Path"=w1548, "IV array"=w1544, "Current Session"=w1531, "Parameters"=w1543, "RecipeID"=w1533, "User"=w1532, "Coords"=w1535, "Wafer Info"="Wafer Info 3", "Mask Name"=w1547, "Temp Data"=w1536, "Die Number"=w1537) -> ()  [unwired: 16 in, 1 out]
                            }
                          }
                          n968 = Increment(x=w1394) -> (x+1=w1374:i32)
                          n969 = Divide(x=w1374, y=w1393) -> (x/y=w1392:dbl)
                          n970 = local write "Current Device"(w1374) -> ()
                          n971 = Multiply(x=100.0, y=w1392) -> (x*y=w1390:dbl)
                          n972 = Number To Decimal String(number=w1374) -> (decimal integer string=w1379:string)  [unwired: 1 in]
                          n973 = To Unsigned Byte Integer(number=w1390) -> (unsigned 8bit integer=w1389:u8)
                          n974 = Concatenate Strings("IV test for die number: " ("string"), w1379) -> (w1378:string)
                          n975 = local write "Progress 2"(w1389) -> ()
                          n976 = local write "Status"(w1378) -> ()
                        }
                      }
                      frame #2 {
                        w1553 = -1 ("x")
                        n977 = local read "Prober GPIB"() -> (w1557:string)
                        n978 = local read "current y"() -> (w1554:i32)
                        n979 = local read "current x"() -> (w1555:i32)
                        n980 = Multiply(x=w1554, y=w1553) -> (x*y=w1551:i32)
                        n981 = Multiply(x=w1553, y=w1555) -> (x*y=w1552:i32)
                        n982 = call "EG2001 Move Z Down.vi"("GPIB Address"=w1557) -> ("Error Out"=w1556:errorcluster, "GPIB Address Out"=w1558:string)  [unwired: 9 in]
                        n983 = call "EG2001 Move Machine Step X-Y.vi"("Flip X Coordinates?"=FALSE, "Y"=w1551, "Steps/Microns"=enum32{"Steps", "Microns"}."Microns", "X"=w1552, "error in (no error)"=w1556, "GPIB Address"=w1558) -> ()  [unwired: 4 in, 2 out]
                      }
                      frame #3 {
                        w1559 = 0 ("current x")
                        n984 = local write "current y"(w1559) -> ()
                        n985 = local write "current x"(w1559) -> ()
                      }
                    }
                  }
                }
              }
              frame #1 {
                n986 = local write "no file"(FALSE ("no file")) -> ()
              }
            }
          }
          frame "update temperature" {
            # "Temptronics is communicatied via VISA sreial commands. RS sets the temperature, and ST tells the TEC to set the current temperature on the output pins to be read"
            n987 = local read "Temp Setpoint"() -> (w1568:string)
            n988 = local read "Temptronics VISA"() -> (w1566:refnum<visa-resource-name>)
            n989 = Concatenate Strings("rs" ("string"), w1568) -> (w1567:string)
            n990 = VISA Write(VISA resource name=w1566, write buffer=w1567) -> (VISA resource name out=w1565:refnum<visa-resource-name>)  [unwired: 1 in, 2 out]
            n991 = VISA Write(VISA resource name=w1565, write buffer="st") -> (VISA resource name out=w1563:refnum<visa-resource-name>, return count=w1562:u32)  [unwired: 1 in, 1 out]
            n992 = VISA Read(VISA resource name=w1563, byte count=w1562) -> (read buffer=w1561:string)  [unwired: 1 in, 3 out]
            n993 = local write "Current Temp"(w1561) -> ()
          }
          frame "Update Laser" {
            # "Sets the laser current to the values set in the Laser Current (mA) box. Then uses the calibration file to find the appropriate power and updates that. Finally updates the compliance for the sweeps so illuminated IV curves don't just hit compliance due to photogenerated current"
            n994 = flat-sequence {
              frame #0 {
                n995 = local read "TL4000 In"() -> (w1577:refnum<visa-resource-name>)
                n996 = local read "Laser Current (mA)"() -> (w1574:dbl)
                n997 = Divide(x=w1574, y=1000.0) -> (x/y=w1589:dbl)
                n998 = call <instrlib>:"TL4000 Set Laser Diode Current Setpoint.vi"("Laser Diode Current Setpoint (0.0)"=w1589, "instrument handle"=w1577) -> ()  [unwired: 8 in, 2 out]
                n999 = call-poly <vilib>:"Read From Spreadsheet File.vi"("delimiter (\\t)"="," ("delimiter (\\t)"), "file path (dialog if empty)"="Load Calibration File") -> ("all rows"=w1584:dbl[][])  [unwired: 5 in, 4 out]
                n1000 = Index Array(array=w1584, index (row)=0) -> (element=w1586:dbl[])  [unwired: 1 in]
                n1001 = Index Array(array=w1584, index (row)=1) -> (element=w1576:dbl[])  [unwired: 1 in]
                n1002 = Array Size(array=w1576) -> (size(s)=w1575:i32)
                n1003 = call "Convert to Dynamic Data2"("Array"=w1576) -> ("Dynamic Data Type"=w1588:dynamicdata)  [unwired: 3 in]
                n1004 = call "Convert to Dynamic Data"("Array"=w1586) -> ("Dynamic Data Type"=w1587:dynamicdata)  [unwired: 3 in]
                n1005 = for {
                  N: w1575 -> [_]
                  tunnel: w1586 -> [w1594] mode=indexing
                  tunnel: w1574 -> [w1595]
                  tunnel: w1576 -> [w1593]
                  tunnel: [w1591] -> w1581
                  i -> [w1592]
                  stop <- w1590 stop-if-true
                  n1006 = Equal?(x=w1594, y=w1595) -> (x = y?=w1590:bool)
                  n1007 = case shown="False" w1590 {
                    tunnel: w1593 -> [_ w1598]
                    tunnel: w1592 -> [_ w1597]
                    tunnel: [_ w1596] -> w1591
                    frame False {
                    }
                    frame True {
                      n1008 = Index Array(array=w1598, index=w1597) -> (element=w1596:dbl)
                    }
                  }
                }
                "Output Power (mW)" <- w1581
                n1009 = call "Build XY Graph"("Y Input"=w1588, "X Input"=w1587) -> ("XY Graph"=→"Calibration":cluster{"Y":dbl[], "Y":dbl[]}[])  [unwired: 3 in, 6 out]
              }
              frame #1 {
                n1010 = case shown="True" "Auto Adjust Compliance?" {
                  frame False {
                  }
                  frame True {
                    n1011 = local read "Output Power (mW)"() -> (w1602:dbl)
                    n1012 = Greater Or Equal?(x=w1602, y=0.1) -> (x >= y?=w1600:bool)
                    n1013 = case shown="False" w1600 {
                      frame False {
                        n1014 = local write "I compliance sweep"(0.001 ("I compliance sweep")) -> ()
                      }
                      frame True {
                        n1015 = local read "Output Power (mW)"() -> (w1606:dbl)
                        n1016 = Multiply(x=w1606, y=0.001) -> (x*y=w1604:dbl)
                        n1017 = local write "I compliance sweep"(w1604) -> ()
                      }
                    }
                  }
                }
              }
            }
          }
          frame "Zero Laser" {
            # "Does not actually update laser - just changer the laser current variable to zero."
            n1018 = local write "Laser Current (mA)"(0.0) -> ()
          }
          frame "raw mask updated" {
            # "Asks if the manual mask should be updated to match the new raw mask file"
            n1019 = Enqueue Element At Opposite End(queue=w1616, element="idle", error in (no error)=w1615) -> (queue out=w1618:refnum<queue>, error out=w1617:errorcluster)  [unwired: 1 in, 1 out]
            n1020 = Two Button Dialog(message="Wold you like to update the Manual mask?", 1:"No" ("F button name (\"Cancel\")"), 2:"Yes" ("T button name (\"OK\")")) -> (T button?=w1610:bool)
            n1021 = case shown="True" w1610 {
              frame False {
              }
              frame True {
                n1022 = local read "Mask File Raw"() -> (w1619:path)
                n1023 = local write "Mask File Manual"(w1619) -> ()
              }
            }
          }
          frame "mask manual update" {
            # "asks if the raw test mask should be changed to math manual mask"
            n1024 = Enqueue Element At Opposite End(queue=w1626, element="idle", error in (no error)=w1625) -> (queue out=w1628:refnum<queue>, error out=w1627:errorcluster)  [unwired: 1 in, 1 out]
            n1025 = Two Button Dialog(message="Would you like update mask file for raw test?", 1:"No" ("F button name (\"Cancel\")"), 2:"Yes" ("T button name (\"OK\")")) -> (T button?=w1620:bool)
            n1026 = case shown="True" w1620 {
              frame False {
              }
              frame True {
                n1027 = local read "Mask File Manual"() -> (w1629:path)
                n1028 = local write "Mask File Raw"(w1629) -> ()
              }
            }
          }
          frame "save comment" {
            # "Uses activex to open the measurement log, save the comment to the approprate cell, and attempt to close the file again. As it stands, the file always stays open after this is run."
            n1029 = flat-sequence {
              frame #0 {
                # "6"
                # "5"
                # "4"
                # "3"
                # "2"
                # "1"
                # "This example demonstrates how to close a Worksheet from an Excel Workbook. \n\nThe steps are as follows:\n1) Open Excel\n2) Open the specific workbook\n3) Open a Specific Sheet\n4) Find a range in that sheet to clear \n5) For adding individual data points, you can use the same range refnum to send in coordinates and the new values. \n6) Close all open references"
                n1030 = Path To String(path="Measurement Log Path") -> (string=w1632:string)
                n1031 = Automation Open(Automation Refnum=refnum<k7> refnum ("Excel._Application")) -> (Automation Refnum=w1679:refnum<k7>, error out=w1678:errorcluster)  [unwired: 3 in]
                n1032 = property on="Property Node" class="_Application"(reference=w1679, error in=w1678, "Visible"=TRUE) -> (reference out=w1675:refnum<k7>, error out=w1674:errorcluster, "Workbooks"=w1676:refnum<k7>)
                n1033 = invoke on="Invoke Node" class="Workbooks" method="Open"(reference=w1676, error in=w1674, "Filename"=w1632, "ReadOnly"=FALSE, "Editable"=TRUE) -> (error out=w1673:errorcluster, "Open"=w1644:refnum<k7>)  [unwired: 13 in, 16 out]
                n1034 = property on="Property Node" class="_Workbook"(reference=w1644, error in=w1673) -> (reference out=w1641:refnum<k7>, error out=w1672:errorcluster, "Worksheets"=w1667:refnum<k7>)
                n1035 = invoke on="Invoke Node" class="Sheets" method="Item"(reference=w1667, error in=w1672, "Index"="MeasurementLog") -> (reference out=w1661:refnum<k7>, error out=w1666:errorcluster, "Item"=w1669:variant)  [unwired: 1 in, 1 out]
                n1036 = local read "Logview"() -> (w1680:i32)
                n1037 = Variant To Data(error in=w1666, type=refnum<k7> refnum ("reference"), Variant=w1669) -> (data=w1639:refnum<k7>, error out=w1654:errorcluster)
                n1038 = Build Array(w1680) -> (w1650:i32[])
                n1039 = To Variant(anything="A1") -> (Variant=w1662:variant)
                n1040 = To Variant(anything="A1") -> (Variant=w1663:variant)
                n1041 = local read "Add Comments"() -> (w1651:string)
                n1042 = invoke on="Invoke Node" class="_Worksheet" method="Range"(reference=w1639, error in=w1654, "Cell1"=w1662, "Cell2"=w1663) -> (error out=w1653:errorcluster, "Range"=w1656:refnum<k7>)  [unwired: 1 in, 3 out]
                n1043 = Index Array(array=w1650, index=0) -> (element=w1647:i32)
                n1044 = Add(x=w1647, y=1) -> (x+y=w1645:i32)
                n1045 = invoke on="Invoke Node" class="Range" method="ListNames"(reference=w1656, error in=w1653) -> (reference out=w1655:refnum<k7>, error out=w1652:errorcluster)  [unwired: 1 in, 1 out]
                n1046 = To Variant(anything=w1651) -> (Variant=w1659:variant)
                n1047 = invoke on="Invoke Node" class="Range" method="Item"(reference=w1655, error in=w1652, "RowIndex"=w1645, "ColumnIndex"=7, "newValue"=w1659) -> (reference out=w1657:refnum<k7>, error out=w1640:errorcluster)  [unwired: 1 in, 4 out]
                n1048 = invoke class="_Worksheet" method="SaveAs"(reference=w1639, error in=w1640, "Filename"=w1632) -> (reference out=w1635:refnum<k7>, error out=w1634:errorcluster)  [unwired: 10 in, 11 out]
                n1049 = Close Reference(reference=w1657, error in (no error)=w1634) -> (error out=w1668:errorcluster)
                n1050 = Close Reference(reference=w1661, error in (no error)=w1668) -> (error out=w1642:errorcluster)
                n1051 = Close Reference(reference=w1641, error in (no error)=w1642) -> (error out=w1643:errorcluster)
                n1052 = Close Reference(reference=w1675, error in (no error)=w1643) -> (error out=w1637:errorcluster)
                n1053 = Close Reference(reference=w1635, error in (no error)=w1637) -> (error out=w1636:errorcluster)
                n1054 = call <vilib>:"Simple Error Handler.vi"("error in (no error)"=w1636) -> ()  [unwired: 4 in, 5 out]
              }
            }
          }
          frame "update viewer" {
            # "Makes the logview table match the measurements log csv"
            n1055 = call-poly <vilib>:"Read From Spreadsheet File.vi"("file path (dialog if empty)"=path "C:/Users/Flash/Desktop/Data/Detector test data/MeasurementLog.csv") -> ("all rows"=w1683:string[][])  [unwired: 6 in, 4 out]
            n1056 = property on="Logview" class="MCListbox (strict)"("ItemNames"=w1683) -> ()  [unwired: 2 in, 2 out]
          }
          frame "refresh device names" {
            # "Ideally populates device nam elist for auto test with devices from the appropriate mask file. Isnt woking at this time, the user needs to manually type in device names"
            n1057 = Enqueue Element At Opposite End(queue=w1694, element="idle", error in (no error)=w1693) -> (queue out=w1695:refnum<queue>, error out=w1690:errorcluster)  [unwired: 1 in, 1 out]
            n1058 = call "getDB unique Device.vi"("error in (no error)"=w1690, "Mask"="Mask Name") -> ("NameList"=w1686:string[])  [unwired: 8 in, 1 out]
            "NameList" <- w1686
            n1059 = Equal?(x=w1686, y=string[] []) -> (x = y?=w1688:bool[])
            n1060 = And Array Elements(Boolean array=w1688) -> (logical AND=w1687:bool)
            n1061 = case shown="True" w1687 {
              tunnel: w1686 -> [w1696 w1698]
              tunnel: [w1696 w1697] -> w1685
              frame False {
              }
              frame True {
                n1062 = call "Prompt User for Input"() -> ("YES"=w1699:bool)  [unwired: 18 in, 1 out]
                n1063 = case shown="True" w1699 {
                  tunnel: w1698 -> [w1700 _]
                  tunnel: [w1700 w1701] -> w1697
                  frame False {
                  }
                  frame True {
                    # "GET DEVICES FROM FILE"
                    n1064 = local read "Mask File all"() -> (w1702:path)
                    n1065 = call "Select unique devices from File.vi"("MaskFile"=w1702) -> ("Device Array"=w1701:string[])  [unwired: 10 in]
                  }
                }
              }
            }
            n1066 = property on="Available Device Name" class="CmbBox"("Strings[]"=w1685) -> ()  [unwired: 2 in, 2 out]
          }
          frame "add to list" {
            # "Adds available device name to test list. If Skip Raw Test Is selected, it appends (skip) on the device name, which the auto test uses to know when to skip the raw test."
            n1067 = Enqueue Element At Opposite End(queue=w1706, element="idle", error in (no error)=w1704) -> (queue out=w1708:refnum<queue>, error out=w1707:errorcluster)  [unwired: 1 in, 1 out]
            n1068 = case shown="False" "Skip Raw Test?" {
              frame False {
                n1069 = local read "Available Device Name"() -> (w1710:string)
                n1070 = property on="Test List" class="LstBox (strict)"() -> ("Item Names"=w1709:string[])  [unwired: 2 in, 2 out]
                n1071 = Build Array (concatenate)(w1709, w1710) -> (w1711:string[])
                n1072 = property on="Test List" class="LstBox (strict)"("Item Names"=w1711) -> ()  [unwired: 2 in, 2 out]
              }
              frame True {
                n1073 = local read "Available Device Name"() -> (w1714:string)
                n1074 = property on="Test List" class="LstBox (strict)"() -> ("Item Names"=w1715:string[])  [unwired: 2 in, 2 out]
                n1075 = Concatenate Strings(w1714, "(skip)" ("string")) -> (w1712:string)
                n1076 = Build Array (concatenate)(w1715, w1712) -> (w1716:string[])
                n1077 = property on="Test List" class="LstBox (strict)"("Item Names"=w1716) -> ()  [unwired: 2 in, 2 out]
              }
            }
          }
          frame "skip raw?" {
            # "First checks to see of (skip) is appended on the current device name. If it isnt, it sets \"raw test skipped\" to false. It (skip) is appended on the end, then it removes it and sets \"raw test skipped\" to true."
            n1078 = property on="Test List" class="LstBox (strict)"() -> ("Item Names"=w1725:string[])  [unwired: 2 in, 2 out]
            n1079 = local read "Counter"() -> (w1724:i32)
            n1080 = Index Array(array=w1725, index=w1724) -> (element=w1723:string)
            "device name w skip" <- w1723
            n1081 = Search/Split String(string=w1723, search string/char (-)="(skip)") -> (match + rest of string=w1721:string)  [unwired: 1 in, 2 out]
            n1082 = Equal?(x=w1721, y="") -> (x = y?=w1719:bool)
            n1083 = local write "no file"(FALSE ("no file")) -> ()
            n1084 = Not(x=w1719) -> (.not. x?=w1718:bool)
            n1085 = case shown="False" w1718 {
              frame False {
                n1086 = local write "Raw Test Skipped"(FALSE ("Skipped")) -> ()
              }
              frame True {
                n1087 = flat-sequence {
                  tunnel: [w1734] -> w1731
                  tunnel: [w1733] -> w1730
                  tunnel: [w1732] -> w1729
                  tunnel: w1731 -> [w1742]
                  tunnel: w1730 -> [w1741]
                  tunnel: w1729 -> [w1740]
                  frame #0 {
                    n1088 = property on="Test List" class="LstBox (strict)"() -> ("Item Names"=w1734:string[])  [unwired: 2 in, 2 out]
                    n1089 = local read "Counter"() -> (w1733:i32)
                    n1090 = Index Array(array=w1734, index=w1733) -> (element=w1736:string)
                    n1091 = Search/Split String(string=w1736, search string/char (-)="(skip)") -> (substring before match=w1732:string)  [unwired: 1 in, 2 out]
                  }
                  frame #1 {
                    n1092 = Delete From Array(array=w1742, index=w1741) -> (array with subset deleted=w1739:string[])  [unwired: 1 in, 1 out]
                    n1093 = Insert Into Array(array=w1739, index=w1741, new element=w1740) -> (w1738:string[])
                    n1094 = property on="Test List" class="LstBox (strict)"("Item Names"=w1738) -> ()  [unwired: 2 in, 2 out]
                    "Raw Test Skipped" <- TRUE ("Skipped")
                  }
                }
              }
            }
          }
          frame "add to laser list" {
            # "Adds \"desired current\" value to current list"
            n1095 = property on="Laser List" class="LstBox (strict)"() -> ("Item Names"=w1747:string[])  [unwired: 2 in, 2 out]
            n1096 = local read "Desired Current (mA)"() -> (w1744:dbl)
            n1097 = Format Into String(format string="%08.4f", w1744) -> (resulting string=w1743:string)  [unwired: 2 in, 1 out]
            n1098 = Build Array (concatenate)(w1747, w1743) -> (w1746:string[])
            n1099 = property on="Laser List" class="LstBox (strict)"("Item Names"=w1746) -> ()  [unwired: 2 in, 2 out]
          }
          frame "remove from laser list" {
            # "removes highlighted value from laser list"
            n1100 = local read "Laser List"() -> (w1754:i32)
            n1101 = property on="Laser List" class="LstBox (strict)"() -> ("Item Names"=w1753:string[])  [unwired: 2 in, 2 out]
            n1102 = Delete From Array(array=w1753, index=w1754) -> (array with subset deleted=w1752:string[])  [unwired: 1 in, 1 out]
            n1103 = property on="Laser List" class="LstBox (strict)"("Item Names"=w1752) -> ()  [unwired: 2 in, 2 out]
          }
          frame "clear laser list" {
            # "removes all values from laser list"
            n1104 = property on="Laser List" class="LstBox (strict)"("Item Names"=string[] []) -> ()  [unwired: 2 in, 2 out]
          }
          frame "remove from list" {
            # "removes highlighted value from test list"
            n1105 = property on="Test List" class="LstBox (strict)"() -> ("Item Names"=w1760:string[])  [unwired: 2 in, 2 out]
            n1106 = local read "Test List"() -> (w1758:i32)
            n1107 = Enqueue Element At Opposite End(queue=w1762, element="idle", error in (no error)=w1761) -> (queue out=w1764:refnum<queue>, error out=w1763:errorcluster)  [unwired: 1 in, 1 out]
            n1108 = Delete From Array(array=w1760, index=w1758) -> (array with subset deleted=w1759:string[])  [unwired: 1 in, 1 out]
            n1109 = property on="Test List" class="LstBox (strict)"("Item Names"=w1759) -> ()  [unwired: 2 in, 2 out]
          }
          frame "clear list" {
            # "removes all values from test list"
            n1110 = property on="Test List" class="LstBox (strict)"("Item Names"=string[] []) -> ()  [unwired: 2 in, 2 out]
            n1111 = Enqueue Element(queue=w1769, element="idle", error in (no error)=w1767) -> (queue out=w1771:refnum<queue>, error out=w1770:errorcluster)  [unwired: 1 in, 1 out]
          }
          frame "add to temp list" {
            # "Adds \"desired temperature\" valiue to temp list"
            n1112 = local read "Desired Temperature"() -> (w1775:dbl)
            n1113 = property on="Single Device Temperature List" class="LstBox (strict)"() -> ("Item Names"=w1774:string[])  [unwired: 2 in, 2 out]
            n1114 = Format Into String(format string="%08.4f", w1775) -> (resulting string=w1773:string)  [unwired: 2 in, 1 out]
            n1115 = Build Array (concatenate)(w1774, w1773) -> (w1772:string[])
            n1116 = property on="Single Device Temperature List" class="LstBox (strict)"("Item Names"=w1772) -> ()  [unwired: 2 in, 2 out]
          }
          frame "remove from temp list" {
            # "Removes highlighted value from temperatre list"
            n1117 = property on="Single Device Temperature List" class="LstBox (strict)"() -> ("Item Names"=w1781:string[])  [unwired: 2 in, 2 out]
            n1118 = local read "Single Device Temperature List"() -> (w1780:i32)
            n1119 = Delete From Array(array=w1781, index=w1780) -> (array with subset deleted=w1779:string[])  [unwired: 1 in, 1 out]
            n1120 = property on="Single Device Temperature List" class="LstBox (strict)"("Item Names"=w1779) -> ()  [unwired: 2 in, 2 out]
          }
          frame "clear temp list" {
            # "Removes all values from temp list"
            n1121 = property on="Single Device Temperature List" class="LstBox (strict)"("Item Names"=string[] []) -> ()  [unwired: 2 in, 2 out]
          }
          frame "pick device" {
            # "Takes the device for the current iteration of the auto test and updates the test name. The Counter keeps track of which iteration of the auto test the program is running. After the device name is updated, the counter is incremented by one. If th elast device is reached, the counter is reset to zero for the next test."
            n1122 = Enqueue Element(queue=w1791, element="idle", error in (no error)=w1789) -> (queue out=w1790:refnum<queue>, error out=w1788:errorcluster)  [unwired: 1 in, 1 out]
            n1123 = flat-sequence {
              frame #0 {
                n1124 = local read "Mask File all"() -> (w1794:path)
                n1125 = property on="Test List" class="LstBox (strict)"() -> ("Item Names"=w1796:string[])  [unwired: 2 in, 2 out]
                n1126 = local read "Counter"() -> (w1795:i32)
                n1127 = Index Array(array=w1796, index=w1795) -> (element=w1792:string)
                n1128 = local write "Device Name"(w1792) -> ()
                n1129 = call "Mask file select device.vi"("Device"=w1792, "MaskFile"=w1794) -> ("RawMask"=w1793:path)  [unwired: 9 in]
                n1130 = local write "Mask File Raw"(w1793) -> ()
              }
              frame #1 {
                n1131 = local read "Counter"() -> (w1798:i32)
                n1132 = Increment(x=w1798) -> (x+1=w1797:i32)
                n1133 = local write "Counter"(w1797) -> ()
              }
              frame #2 {
                n1134 = property on="Test List" class="LstBox (strict)"() -> ("Item Names"=w1801:string[])  [unwired: 2 in, 2 out]
                n1135 = local read "Counter"() -> (w1802:i32)
                n1136 = Array Size(array=w1801) -> (size(s)=w1800:i32)
                n1137 = Equal?(x=w1802, y=w1800) -> (x = y?=w1799:bool)
                n1138 = case shown="False" w1799 {
                  frame False {
                  }
                  frame True {
                    n1139 = local write "Counter"(0 ("Counter")) -> ()
                  }
                }
              }
            }
          }
          frame "pick laser" {
            # "See pick device. Mechanics are exactly the same, except for laser instead of device name"
            n1140 = flat-sequence {
              frame #0 {
                n1141 = property on="Laser List" class="LstBox (strict)"() -> ("Item Names"=w1808:string[])  [unwired: 2 in, 2 out]
                n1142 = local read "Laser Counter"() -> (w1809:i32)
                n1143 = Index Array(array=w1808, index=w1809) -> (element=w1807:string)
                n1144 = Fract/Exp String To Number(string=w1807) -> (number=w1806:dbl)  [unwired: 3 in, 1 out]
                n1145 = local write "Laser Current (mA)"(w1806) -> ()
              }
              frame #1 {
                n1146 = local read "Laser Counter"() -> (w1811:i32)
                n1147 = Increment(x=w1811) -> (x+1=w1810:i32)
                n1148 = local write "Laser Counter"(w1810) -> ()
              }
              frame #2 {
                n1149 = property on="Laser List" class="LstBox (strict)"() -> ("Item Names"=w1812:string[])  [unwired: 2 in, 2 out]
                n1150 = local read "Laser Counter"() -> (w1815:i32)
                n1151 = Array Size(array=w1812) -> (size(s)=w1814:i32)
                n1152 = Equal?(x=w1815, y=w1814) -> (x = y?=w1813:bool)
                n1153 = case shown="True" w1813 {
                  frame False {
                  }
                  frame True {
                    n1154 = local write "Laser Counter"(0 ("Counter")) -> ()
                  }
                }
              }
            }
          }
          frame "reset skip" {
            # "If the raw test was skipped, during the auto test the (skip) tag was removed from the device mane during testing. This replaces the (skip)tag so the user can run another test"
            n1155 = local read "Counter"() -> (w1819:i32)
            n1156 = property on="Test List" class="LstBox (strict)"() -> ("Item Names"=w1821:string[])  [unwired: 2 in, 2 out]
            n1157 = Not Equal?(x=w1819, y=0) -> (x != y?=w1817:bool)
            n1158 = case shown="False" w1817 {
              tunnel: w1821 -> [w1826 w1835]
              tunnel: [w1827 w1831] -> w1820
              frame False {
                n1159 = Array Size(array=w1826) -> (size(s)=w1825:i32)
                n1160 = local read "device name w skip"() -> (w1829:string)
                n1161 = Decrement(x=w1825) -> (x-1=w1824:i32)
                n1162 = Delete From Array(array=w1826, index=w1824) -> (array with subset deleted=w1828:string[])  [unwired: 1 in, 1 out]
                n1163 = Insert Into Array(array=w1828, index=w1824, new element=w1829) -> (w1827:string[])
              }
              frame True {
                n1164 = local read "Counter"() -> (w1832:i32)
                n1165 = local read "device name w skip"() -> (w1834:string)
                n1166 = Subtract(x=w1832, y=1) -> (x-y=w1830:i32)
                n1167 = Delete From Array(array=w1835, index=w1830) -> (array with subset deleted=w1833:string[])  [unwired: 1 in, 1 out]
                n1168 = Insert Into Array(array=w1833, index=w1830, new element=w1834) -> (w1831:string[])
              }
            }
            n1169 = property on="Test List" class="LstBox (strict)"("Item Names"=w1820) -> ()  [unwired: 2 in, 2 out]
          }
          frame "load wafer" {
            # "tells probe station to load wafer"
            n1170 = flat-sequence {
              frame #0 {
                n1171 = local read "Prober GPIB"() -> (w1843:string)
                n1172 = local write "Status"("loading..." ("Status")) -> ()
                n1173 = call "EG2001 Load Wafer.vi"("Enable Error Message"=FALSE, "error in (no error)"=errorcluster {"status"=FALSE, "code"=0, "source"=""}, "Characters to Write"="LO", "GPIB Address"=w1843) -> ()  [unwired: 5 in, 3 out]
              }
              frame #1 {
                n1174 = local write "Status"("load complete" ("Status")) -> ()
              }
            }
          }
          frame "profile z" {
            # "tells pobe station to run \"profile z\" program"
            n1175 = local read "Prober GPIB"() -> (w1846:string)
            n1176 = call "EG2001 Profile Wafer Only.vi"("GPIB Address"=w1846) -> ("Error Out"=→"Error Out":errorcluster)  [unwired: 9 in, 1 out]
          }
          frame "auto align" {
            # "tells prober to run \"auto align\" feature. Only works if ref is already stored, if find target needs to be run, that needs to be done manually, (see prober guide for details)."
            n1177 = flat-sequence {
              frame #0 {
                n1178 = local read "Prober GPIB"() -> (w1852:string)
                n1179 = local write "Status"("aligning" ("Status")) -> ()
                n1180 = call "EG2001 Auto Align Wafer.vi"("GPIB Address"=w1852) -> ()  [unwired: 8 in, 3 out]
              }
              frame #1 {
                n1181 = local write "Status"("idle" ("Status")) -> ()
              }
            }
          }
          frame "wait" {
            # "delays for a certain number of seconds, determined by the \"wait after load\" parameter"
            n1182 = Multiply(x="Wait after load", y=u32 1000) -> (x*y=w1854:u32)
            n1183 = Wait (ms)(milliseconds to wait=w1854) -> ()  [unwired: 1 out]
          }
          frame "add to wafer list" {
            # "adds \"desired wafer name\" to wafer list"
            n1184 = property on="Wafer List" class="LstBox (strict)"() -> ("Item Names"=w1860:string[])  [unwired: 2 in, 2 out]
            n1185 = local read "Desired Wafer Name"() -> (w1861:string)
            n1186 = Build Array (concatenate)(w1860, w1861) -> (w1859:string[])
            n1187 = property on="Wafer List" class="LstBox (strict)"("Item Names"=w1859) -> ()  [unwired: 2 in, 2 out]
          }
          frame "remove from wafer list" {
            # "Removes highlighted value from wafer list"
            n1188 = property on="Wafer List" class="LstBox (strict)"() -> ("Item Names"=w1865:string[])  [unwired: 2 in, 2 out]
            n1189 = local read "Wafer List"() -> (w1866:i32)
            n1190 = Delete From Array(array=w1865, index=w1866) -> (array with subset deleted=w1864:string[])  [unwired: 1 in, 1 out]
            n1191 = property on="Wafer List" class="LstBox (strict)"("Item Names"=w1864) -> ()  [unwired: 2 in, 2 out]
          }
          frame "clear wafer list" {
            # "Deletes all values in wafer list"
            n1192 = property on="Wafer List" class="LstBox (strict)"("Item Names"=string[] []) -> ()  [unwired: 2 in, 2 out]
          }
          frame "desired device change" {
            # "works the same as \"die number changed\" but in the temperature tab"
            n1193 = flat-sequence {
              frame #0 {
                n1194 = local read "Desired Device"() -> (w1881:u16)
                n1195 = local read "Array of Cell Data Clusters"() -> (w1882:T12)
                n1196 = Index Array(array=w1882, index=w1881) -> (element=w1880:T17)
                n1197 = Unbundle By Name(w1880) -> ("Cell Name"=w1879:string, "X-coord"=w1876:dbl, "Y-coord"=w1875:dbl, "Area"=w1878:dbl, "Meas Area"=w1877:dbl)
                "X" <- w1876
                "Y" <- w1875
                n1198 = local write "Device Name"(w1879) -> ()
                n1199 = local write "x target"(w1876) -> ()
                n1200 = local write "y target"(w1875) -> ()
                n1201 = local write "ActiveArea_um2"(w1878) -> ()
                n1202 = local write "MesaArea_um2"(w1877) -> ()
              }
              frame #1 {
                n1203 = local read "J set A/cm2"() -> (w1888:dbl)
                n1204 = local read "Laser Current (mA)"() -> (w1885:dbl)
                n1205 = Equal To 0?(x=w1885) -> (x = 0?=w1884:bool)
                n1206 = case shown="True" w1884 {
                  tunnel: [w1890 w1891] -> w1883
                  frame False {
                    n1207 = local read "ActiveArea_um2"() -> (w1890:dbl)
                  }
                  frame True {
                    n1208 = local read "MesaArea_um2"() -> (w1891:dbl)
                  }
                }
                n1209 = Divide(x=w1883, y=100000000.0) -> (x/y=w1887:dbl)
                n1210 = Multiply(x=w1887, y=w1888) -> (x*y=w1889:dbl)
                n1211 = local write "I set"(w1889) -> ()
              }
            }
            n1212 = local write "Status"("Changing Die" ("Status")) -> ()
          }
          frame "select temperature" {
            # "Updates the current temperature from the temperature list, and updates the counter, which operates the same as laser, wafer, and auto test counters"
            n1213 = flat-sequence {
              frame #0 {
                n1214 = local read "Auto Temp Counter"() -> (w1897:i32)
                n1215 = property on="Auto Temperature List" class="LstBox (strict)"() -> ("Item Names"=w1894:string[])  [unwired: 2 in, 2 out]
                n1216 = local write "Status"("selecting temperature" ("Status")) -> ()
                n1217 = Index Array(array=w1894, index=w1897) -> (element=w1895:string)
                n1218 = local write "Temp Setpoint"(w1895) -> ()
              }
              frame #1 {
                n1219 = local read "Auto Temp Counter"() -> (w1899:i32)
                n1220 = Increment(x=w1899) -> (x+1=w1898:i32)
                n1221 = local write "Auto Temp Counter"(w1898) -> ()
              }
              frame #2 {
                n1222 = property on="Auto Temperature List" class="LstBox (strict)"() -> ("Item Names"=w1900:string[])  [unwired: 2 in, 2 out]
                n1223 = local read "Auto Temp Counter"() -> (w1903:i32)
                n1224 = Array Size(array=w1900) -> (size(s)=w1902:i32)
                n1225 = Equal?(x=w1903, y=w1902) -> (x = y?=w1901:bool)
                n1226 = case shown="True" w1901 {
                  frame False {
                  }
                  frame True {
                    n1227 = local write "Auto Temp Counter"(0 ("Counter")) -> ()
                  }
                }
              }
            }
          }
          frame "wait for temperature" {
            # "This while loop checks every five seconds whether the temperature has reached the setpoint, and if it has it exits the while loop and allows the program to continue"
            n1228 = local read "Temp Controller Found"() -> (w1905:bool)
            n1229 = case shown="True" w1905 {
              frame False {
              }
              frame True {
                n1230 = while {
                  i -> [w1911]
                  stop <- w1908 stop-if-true
                  n1231 = flat-sequence {
                    tunnel: [w1917] -> w1910
                    tunnel: w1911 -> [w1925]
                    tunnel: [w1924] -> w1909
                    frame #0 {
                      n1232 = local read "Temptronics VISA"() -> (w1921:refnum<visa-resource-name>)
                      n1233 = Wait (ms)(milliseconds to wait=u32 500) -> ()  [unwired: 1 out]
                      n1234 = VISA Write(VISA resource name=w1921, write buffer="st") -> (VISA resource name out=w1920:refnum<visa-resource-name>, return count=w1919:u32)  [unwired: 1 in, 1 out]
                      n1235 = local read "Temp Setpoint"() -> (w1913:string)
                      n1236 = local write "Status"("waiting for temperature..." ("Status")) -> ()
                      n1237 = VISA Read(VISA resource name=w1920, byte count=w1919) -> (read buffer=w1915:string)  [unwired: 1 in, 3 out]
                      n1238 = Decimal String To Number(string=w1915) -> (number=w1914:i32)  [unwired: 2 in, 1 out]
                      n1239 = Decimal String To Number(string=w1913) -> (number=w1912:i32)  [unwired: 2 in, 1 out]
                      n1240 = Equal?(x=w1914, y=w1912) -> (x = y?=w1917:bool)
                    }
                    frame #1 {
                      n1241 = Equal?(x=w1925, y=500) -> ()  [unwired: 1 out]
                      n1242 = case shown="False" FALSE {
                        tunnel: [_ w1927] -> w1924
                        frame False {
                        }
                        frame True {
                          n1243 = One Button Dialog(message="Temperature Timeout") -> (true=w1927:bool)  [unwired: 1 in]
                        }
                      }
                    }
                  }
                  n1244 = Or(x=w1909, y=w1910) -> (x .or. y?=w1908:bool)
                }
              }
            }
          }
          frame "temp to 25" {
            n1245 = local write "Temp Setpoint"("25" ("Temp Setpoint")) -> ()
          }
          frame "load file for temp" {
            # "same as load manual mask file, but in the temperature tab"
            n1246 = flat-sequence {
              tunnel: [w1942] -> w1937
              tunnel: w1937 -> [w1945]
              frame #0 {
                n1247 = local read "Mask File Temperature"() -> (w1938:path)
                n1248 = local write "Status"("Loading mask file" ("Status")) -> ()
                n1249 = call "Device Files v1.vi"("Rows"=1200, "Mask file path"=w1938) -> ("Mask Name"=w1943:string, "size(s)"=w1942:i32, "Array of Cell Clusters"=w1939:T5)  [unwired: 6 in, 1 out]
                n1250 = local write "Mask"(w1943) -> ()
                n1251 = local write "Array of Cell Data Clusters"(w1939) -> ()
              }
              frame #1 {
                n1252 = for {
                  N: w1945 -> [_]
                  tunnel: [w1946] -> w1944 mode=indexing
                  i -> [w1947]
                  n1253 = Number To Decimal String(number=w1947) -> (decimal integer string=w1946:string)  [unwired: 1 in]
                }
                n1254 = property on="Desired Device" class="Ring (strict)"("Strings []"=w1944) -> ()  [unwired: 2 in, 2 out]
              }
              frame #2 {
                n1255 = local read "Array of Cell Data Clusters"() -> (w1955:T12)
                n1256 = local read "Desired Device"() -> (w1954:u16)
                n1257 = Index Array(array=w1955, index=w1954) -> (element=w1953:T17)
                n1258 = Unbundle By Name(w1953) -> ("Cell Name"=w1948:string, "X-coord"=w1951:dbl, "Y-coord"=w1952:dbl, "Area"=w1950:dbl, "Meas Area"=w1949:dbl)
                n1259 = local write "Device Name"(w1948) -> ()
                n1260 = local write "x target"(w1951) -> ()
                n1261 = local write "y target"(w1952) -> ()
                n1262 = local write "ActiveArea_um2"(w1950) -> ()
                n1263 = local write "MesaArea_um2"(w1949) -> ()
              }
              frame #3 {
                n1264 = local read "Laser Current (mA)"() -> (w1958:dbl)
                n1265 = Equal To 0?(x=w1958) -> (x = 0?=w1957:bool)
                n1266 = case shown="False" w1957 {
                  tunnel: [w1963 w1964] -> w1956
                  frame False {
                    n1267 = local read "ActiveArea_um2"() -> (w1963:dbl)
                  }
                  frame True {
                    n1268 = local read "MesaArea_um2"() -> (w1964:dbl)
                  }
                }
                n1269 = local read "J set A/cm2"() -> (w1961:dbl)
                n1270 = Divide(x=w1956, y=100000000.0) -> (x/y=w1960:dbl)
                n1271 = Multiply(x=w1960, y=w1961) -> (x*y=w1962:dbl)
                n1272 = local write "I set"(w1962) -> ()
              }
            }
            n1273 = Enqueue Element(queue=w1936, element="idle", error in (no error)=w1934) -> (queue out=w1935:refnum<queue>, error out=w1933:errorcluster)  [unwired: 1 in, 1 out]
          }
          frame "begin temperature series" {
            # "In Progress"
            n1274 = flat-sequence {
              frame #0 {
                n1275 = local read "Mask File Temperature"() -> (w1970:path)
                n1276 = local write "Status"("prepare temperature test" ("Status")) -> ()
                n1277 = local write "Mask File Temperature"(w1970) -> ()
                n1278 = local write "Tab Control"(T16."Temperature Series Single Device" ("Tab Control")) -> ()
                n1279 = local read "points"() -> (w1972:u16)
                n1280 = Initialize Array(nan ("element"), w1972) -> (w1974:dbl[])
                n1281 = call "Device Files v1.vi"("Rows"=1200, "Mask file path"=w1970) -> ("size(s)"=w1969:i32, "Array of Cell Clusters"=w1968:T5)  [unwired: 6 in, 2 out]
                n1282 = local write "Fine Cell Clusters"(w1968) -> ()
                n1283 = local write "Total Device"(w1969) -> ()
                n1284 = Bundle(w1974, w1974) -> (w1973:cluster{dbl[], dbl[]})  [unwired: 1 in]
                n1285 = Initialize Array(w1973, w1969) -> (w1967:cluster{dbl[], dbl[]}[])
                n1286 = local write "IV temp linear"(w1967) -> ()
                n1287 = local write "IV temp log"(w1967) -> ()
              }
              frame #1 {
                n1288 = property on="Single Device Temperature List" class="LstBox (strict)"() -> ("Item Names"=w1978:string[])  [unwired: 2 in, 2 out]
                n1289 = for {
                  tunnel: w1978 -> [_] mode=indexing
                  i -> [w1979]
                  n1290 = flat-sequence {
                    frame #0 {
                      n1291 = stacked-sequence {
                        frame #0 {
                          n1292 = property on="Single Device Temperature List" class="LstBox (strict)"() -> ("Item Names"=w1982:string[])  [unwired: 2 in, 2 out]
                          n1293 = local read "TempCounter"() -> (w1983:i32)
                          n1294 = local write "Status"("selecting temperature" ("Status")) -> ()
                          n1295 = Index Array(array=w1982, index=w1983) -> (element=w1980:string)
                          n1296 = local write "Temp Setpoint"(w1980) -> ()
                        }
                        frame #1 {
                          n1297 = local read "Temp Setpoint"() -> (w1991:string)
                          n1298 = local read "Temptronics VISA"() -> (w1989:refnum<visa-resource-name>)
                          n1299 = Concatenate Strings("rs" ("string"), w1991) -> (w1990:string)
                          n1300 = VISA Write(VISA resource name=w1989, write buffer=w1990) -> (VISA resource name out=w1988:refnum<visa-resource-name>)  [unwired: 1 in, 2 out]
                          n1301 = VISA Write(VISA resource name=w1988, write buffer="st") -> (VISA resource name out=w1986:refnum<visa-resource-name>, return count=w1985:u32)  [unwired: 1 in, 1 out]
                          n1302 = VISA Read(VISA resource name=w1986, byte count=w1985) -> (read buffer=w1984:string)  [unwired: 1 in, 3 out]
                          n1303 = local write "Current Temp"(w1984) -> ()
                        }
                        frame #2 {
                          n1304 = local read "TempCounter"() -> (w1994:i32)
                          n1305 = Increment(x=w1994) -> (x+1=w1993:i32)
                          n1306 = local write "TempCounter"(w1993) -> ()
                        }
                        frame #3 {
                          n1307 = property on="Single Device Temperature List" class="LstBox (strict)"() -> ("Item Names"=w1995:string[])  [unwired: 2 in, 2 out]
                          n1308 = local read "TempCounter"() -> (w1998:i32)
                          n1309 = Array Size(array=w1995) -> (size(s)=w1997:i32)
                          n1310 = Equal?(x=w1998, y=w1997) -> (x = y?=w1996:bool)
                          n1311 = case shown="False" w1996 {
                            frame False {
                            }
                            frame True {
                              n1312 = local write "TempCounter"(0 ("Counter")) -> ()
                            }
                          }
                        }
                      }
                    }
                    frame #1 {
                      n1313 = while {
                        i -> [w2003]
                        stop <- w2000 stop-if-true
                        n1314 = flat-sequence {
                          tunnel: [w2009] -> w2002
                          tunnel: w2003 -> [w2016]
                          tunnel: [w2015] -> w2001
                          frame #0 {
                            n1315 = local read "Temptronics VISA"() -> (w2013:refnum<visa-resource-name>)
                            n1316 = Wait (ms)(milliseconds to wait=u32 500) -> ()  [unwired: 1 out]
                            n1317 = VISA Write(VISA resource name=w2013, write buffer="st") -> (VISA resource name out=w2012:refnum<visa-resource-name>, return count=w2011:u32)  [unwired: 1 in, 1 out]
                            n1318 = local read "Temp Setpoint"() -> (w2005:string)
                            n1319 = local write "Status"("waiting for temperature..." ("Status")) -> ()
                            n1320 = VISA Read(VISA resource name=w2012, byte count=w2011) -> (read buffer=w2007:string)  [unwired: 1 in, 3 out]
                            n1321 = Decimal String To Number(string=w2007) -> (number=w2006:i32)  [unwired: 2 in, 1 out]
                            n1322 = Decimal String To Number(string=w2005) -> (number=w2004:i32)  [unwired: 2 in, 1 out]
                            n1323 = Equal?(x=w2006, y=w2004) -> (x = y?=w2009:bool)
                          }
                          frame #1 {
                            n1324 = Equal?(x=w2016, y=1000) -> (x = y?=w2018:bool)
                            n1325 = case shown="False" w2018 {
                              tunnel: [_ w2019] -> w2015
                              frame False {
                              }
                              frame True {
                                n1326 = One Button Dialog(message="Temperature Timeout") -> (true=w2019:bool)  [unwired: 1 in]
                              }
                            }
                          }
                        }
                        n1327 = Or(x=w2001, y=w2002) -> (x .or. y?=w2000:bool)
                      }
                    }
                    frame #2 {
                      n1328 = local read "Desired Device"() -> (w2033:u16)
                      n1329 = local write "Status"("IV test running..." ("string")) -> ()
                      n1330 = flat-sequence {
                        tunnel: [w2069] -> w2046
                        tunnel: [w2068] -> w2045
                        tunnel: [w2065] -> w2044
                        tunnel: [w2064] -> w2043
                        tunnel: [w2063] -> w2042
                        tunnel: [w2062] -> w2041
                        tunnel: [w2047] -> w2040
                        tunnel: w2033 -> [w2047]
                        tunnel: w2046 -> [w2085]
                        tunnel: w2045 -> [w2084]
                        tunnel: w2044 -> [w2082]
                        tunnel: w2043 -> [w2081]
                        tunnel: w2042 -> [w2080]
                        tunnel: w2041 -> [w2079]
                        tunnel: [w2078] -> w2039
                        tunnel: [w2077] -> w2038
                        tunnel: [w2076] -> w2037
                        tunnel: w2040 -> [w2076]
                        tunnel: w2039 -> [w2095]
                        tunnel: w2038 -> [w2094]
                        tunnel: [w2093] -> w2036
                        tunnel: w2037 -> [w2093]
                        tunnel: [w2107] -> w2035
                        tunnel: w2036 -> [w2107]
                        tunnel: [w2145] -> w2024
                        tunnel: [w2138] -> w2022
                        tunnel: w2035 -> [w2145]
                        tunnel: w2024 -> [w2156]
                        tunnel: [w2156] -> w2023
                        tunnel: w2022 -> [w2155]
                        tunnel: [w2155] -> w2021
                        tunnel: w2023 -> [_]
                        tunnel: [w2181] -> w2032
                        tunnel: [w2175] -> w2030
                        tunnel: [w2174] -> w2028
                        tunnel: w2021 -> [w2173]
                        tunnel: [w2169] -> w2026
                        tunnel: [w2167] -> w2025
                        tunnel: w2032 -> [w2198]
                        tunnel: [w2198] -> w2031
                        tunnel: w2030 -> [w2197]
                        tunnel: [w2197] -> w2029
                        tunnel: w2028 -> [w2196]
                        tunnel: [w2196] -> w2027
                        tunnel: w2026 -> [w2194]
                        tunnel: w2025 -> [w2195]
                        tunnel: w2031 -> [w2216]
                        tunnel: w2029 -> [w2210]
                        tunnel: w2027 -> [w2209]
                        frame #0 {
                          n1331 = local read "Output Power (mW)"() -> (w2052:dbl)
                          n1332 = local read "Fine Cell Clusters"() -> (w2074:T5)
                          n1333 = local read "ActiveArea_um2"() -> (w2054:dbl)
                          n1334 = local read "Laser Current (mA)"() -> (w2058:dbl)
                          n1335 = Multiply(x=w2052, y=0.001) -> (x*y=w2050:dbl)
                          n1336 = Divide(x=w2054, y=100000000.0) -> (x/y=w2049:dbl)
                          n1337 = local read "Output Power (mW)"() -> (w2055:dbl)
                          n1338 = Index Array(array=w2074, index=w2047) -> (element=w2059:T22)
                          n1339 = local read "Laser Current (mA)"() -> (w2056:dbl)
                          n1340 = local read "Parameters Flash 2"() -> (w2061:T4)
                          n1341 = Unbundle By Name(w2059) -> ("Cell Name"=w2073:string, "X-coord"=w2063:dbl, "Y-coord"=w2062:dbl, "Area"=w2072:dbl, "Mesa Area"=w2071:dbl)
                          n1342 = local read "current y"() -> (w2066:i32)
                          n1343 = local read "current x"() -> (w2067:i32)
                          n1344 = call "get Area.vi"("Laser"=w2058, "Cell Data Cluster"=w2059) -> ("Area"=w2060:dbl)  [unwired: 9 in]
                          n1345 = Divide(x=w2050, y=w2049) -> (x/y=w2048:dbl)
                          n1346 = local write "Device Name"(w2073) -> ()
                          n1347 = local write "ActiveArea_um2"(w2072) -> ()
                          n1348 = local write "MesaArea_um2"(w2071) -> ()
                          n1349 = Bundle By Name(cluster=w2061, "Cell Area (cm²)"=w2060, "Input Current (mA)"=w2056, "Power Density (W/cm^2)"=w2048, "Incident Power"=w2055) -> (w2057:T4)
                          n1350 = Subtract(x=w2062, y=w2066) -> (x-y=w2064:dbl)
                          n1351 = Subtract(x=w2063, y=w2067) -> (x-y=w2065:dbl)
                          n1352 = local write "Parameters Flash"(w2057) -> ()
                          n1353 = local read "Prober GPIB"() -> (w2070:string)
                          n1354 = call "EG2001 Move Z Down.vi"("GPIB Address"=w2070) -> ("Error Out"=w2068:errorcluster, "GPIB Address Out"=w2069:string)  [unwired: 9 in]
                        }
                        frame #1 {
                          n1355 = local write "current x"(w2080) -> ()
                          n1356 = local write "current y"(w2079) -> ()
                          n1357 = case shown="False" FALSE {
                            tunnel: w2085 -> [_ w2092]
                            tunnel: w2084 -> [_ w2091]
                            tunnel: enum32{"Steps", "Microns"}."Microns" ("Steps/Microns") -> [_ w2090]
                            tunnel: w2082 -> [_ w2089]
                            tunnel: w2081 -> [_ w2088]
                            tunnel: [_ w2087] -> w2078
                            tunnel: [_ w2086] -> w2077
                            frame False {
                            }
                            frame True {
                              n1358 = call "EG2001 Move Machine Step X-Y.vi"("Y"=w2088, "Steps/Microns"=w2090, "X"=w2089, "error in (no error)"=w2091, "GPIB Address"=w2092) -> ("Error Out"=w2086:errorcluster, "GPIB Address Out"=w2087:string)  [unwired: 5 in]
                            }
                          }
                        }
                        frame #2 {
                          n1359 = call "EG2001 Move Z Up.vi"("error in (no error)"=w2094, "GPIB Address"=w2095) -> ()  [unwired: 10 out]
                        }
                        frame #3 {
                          n1360 = local read "I compliance sweep"() -> (w2111:dbl)
                          n1361 = local read "Wafer Info Flash 2"() -> (w2106:T3)
                          n1362 = local read "sweep delay ms"() -> (w2110:dbl)
                          n1363 = local read "Sweep Settings"() -> (w2117:T10)
                          n1364 = local read "Temp Setpoint"() -> (w2101:string)
                          n1365 = local read "Device Name"() -> (w2105:string)
                          n1366 = local read "Channel"() -> (w2116:enum32{"Channel A", "Channel B"})
                          n1367 = call "DAQ Assistant2"() -> ("data"=w2099:dynamicdata)  [unwired: 17 in, 2 out]
                          n1368 = local read "Temp Data"() -> (w2102:T1)
                          n1369 = Bundle By Name(cluster=w2106, "Cell Name"=w2105) -> (w2104:T3)
                          n1370 = Decimal String To Number(string=w2101) -> (number=w2098:i32)  [unwired: 2 in, 1 out]
                          n1371 = local read "V start"() -> (w2114:dbl)
                          n1372 = local read "points"() -> (w2113:u16)
                          n1373 = local read "V end"() -> (w2115:dbl)
                          n1374 = local read "NPLC"() -> (w2112:dbl)
                          n1375 = Bundle By Name(cluster=w2102, "Ambient Temperature"=w2099, "Chuck Set Temperature"=w2098) -> (w2100:T1)
                          n1376 = local write "Wafer Info Flash"(w2104) -> ()
                          n1377 = Bundle By Name(cluster=w2117, "Channel"=w2116, "Vstart"=w2114, "Vend"=w2115, "# of points"=w2113, "NPLC"=w2112, "I compliance"=w2111, "Delay ms"=w2110) -> (w2096:T10)
                          n1378 = local read "Keysight"() -> (w2097:bool)
                          n1379 = local write "Temp Data"(w2100) -> ()
                          n1380 = local read "4-wire"() -> (w2103:bool)
                          n1381 = local write "Sweep Settings"(w2096) -> ()
                          n1382 = case shown="False" w2097 {
                            tunnel: w2096 -> [w2122 w2127]
                            tunnel: [w2120 w2125] -> w2109
                            tunnel: [w2119 w2124] -> w2108
                            tunnel: w2103 -> [w2118 w2126]
                            frame False {
                              n1383 = local read "Keithley SMU"() -> (w2121:refnum<visa-resource-name>)
                              n1384 = call "K2602 Vsweep.vi"("4-wire"=w2118, "Settings"=w2122, "SMU"=w2121) -> ("V"=w2119:dbl[], "I"=w2120:dbl[])  [unwired: 6 in, 1 out]
                            }
                            frame True {
                              n1385 = local read "Keysight SMU"() -> (w2123:refnum<visa-resource-name>)
                              n1386 = call "IVSweep (SubVI).vi"("SweepSettings"=w2127, "4 wire"=w2126, "VISA Refnum in"=w2123) -> ("V"=w2124:dbl[], "I"=w2125:dbl[])  [unwired: 1 in, 2 out]
                            }
                          }
                          n1387 = local write "I fine"(w2109) -> ()
                          n1388 = local write "V fine"(w2108) -> ()
                        }
                        frame #4 {
                          n1389 = local read "Temperature Series save path"() -> (w2137:path)
                          n1390 = local read "Device Name"() -> (w2129:string)
                          n1391 = local read "Wafer Info 3"() -> (w2128:T2)
                          n1392 = local read "Lot"() -> (w2136:string)
                          n1393 = Build Path(base path=w2137, name or relative path=w2136) -> (appended path=w2135:path)
                          n1394 = local read "Wafer Name"() -> (w2134:string)
                          n1395 = Bundle By Name(cluster=w2128, "Cell Name (Automatic)"=w2129) -> (w2130:T2)
                          n1396 = call "CreateDirectory.vi"("Path to be created"=w2135) -> ()  [unwired: 10 in, 1 out]
                          n1397 = local read "Output Power (mW)"() -> (w2143:dbl)
                          n1398 = Build Path(base path=w2135, name or relative path=w2134) -> (appended path=w2133:path)
                          n1399 = call "CreateDirectory.vi"("Path to be created"=w2133) -> ()  [unwired: 10 in, 1 out]
                          n1400 = local read "Device Name"() -> (w2144:string)
                          n1401 = local write "Wafer Info 3"(w2130) -> ()
                          n1402 = Build Path(base path=w2133, name or relative path="Temperature Series") -> (appended path=w2131:path)
                          n1403 = Number To Decimal String(number=w2143) -> (decimal integer string=w2141:string)  [unwired: 1 in]
                          n1404 = call "CreateDirectory.vi"("Path to be created"=w2131) -> ()  [unwired: 10 in, 1 out]
                          n1405 = Build Path(base path=w2131, name or relative path=w2144) -> (appended path=w2142:path)
                          n1406 = Concatenate Strings(w2141, " mW" ("string")) -> (w2139:string)
                          n1407 = call "CreateDirectory.vi"("Path to be created"=w2142) -> ()  [unwired: 10 in, 1 out]
                          n1408 = Build Path(base path=w2142, name or relative path=w2139) -> (appended path=w2138:path)
                          n1409 = call "CreateDirectory.vi"("Path to be created"=w2138) -> ()  [unwired: 10 in, 1 out]
                        }
                        frame #5 {
                          n1410 = local read "Sweep Direction (Keysight)"() -> (w2154:i32)
                          n1411 = local read "I compliance sweep"() -> (w2150:dbl)
                          n1412 = local read "sweep delay ms"() -> (w2149:dbl)
                          n1413 = local read "V start"() -> (w2153:dbl)
                          n1414 = local read "points"() -> (w2151:u16)
                          n1415 = local read "V end"() -> (w2152:dbl)
                          n1416 = call "pho_DBCheck_LIV_meas_recipe.vi"("V start"=w2153, "Sweep Direction (Keysight)"=w2154, "V end"=w2152, "points"=w2151, "I compliance sweep"=w2150, "sweep delay ms"=w2149) -> ("RecipeID"=w2148:string)  [unwired: 8 in, 1 out]
                          n1417 = local write "RecipeID"(w2148) -> ()
                          n1418 = Equal?(x=w2148, y="") -> (x = y?=w2146:bool)
                          n1419 = case shown="True" w2146 {
                            frame False {
                            }
                            frame True {
                              n1420 = local read "Sweep Direction (Keysight)"() -> (w2163:i32)
                              n1421 = local read "I compliance sweep"() -> (w2159:dbl)
                              n1422 = local read "sweep delay ms"() -> (w2158:dbl)
                              n1423 = local read "V start"() -> (w2162:dbl)
                              n1424 = local read "points"() -> (w2160:u16)
                              n1425 = local read "V end"() -> (w2161:dbl)
                              n1426 = call "pho_DB_Insert_LIV_meas_recipe.vi"("V start"=w2162, "Sweep Direction (Keysight)"=w2163, "V end"=w2161, "points"=w2160, "I compliance sweep"=w2159, "sweep delay ms"=w2158) -> ("RecipeID"=w2157:string)  [unwired: 9 in]
                              n1427 = local write "RecipeID"(w2157) -> ()
                            }
                          }
                        }
                        frame #6 {
                          n1428 = local read "I fine"() -> (w2186:dbl[])
                          n1429 = local read "Wafer Info 3"() -> (w2172:T2)
                          n1430 = local read "Comments"() -> (w2171:string)
                          n1431 = local read "V fine"() -> (w2180:dbl[])
                          n1432 = Absolute Value(x=w2186) -> (abs(x)=w2187:dbl[])
                          n1433 = local read "Temp Setpoint"() -> (w2166:string)
                          n1434 = local read "IV temp linear"() -> (w2192:cluster{dbl[], dbl[]}[])
                          n1435 = local read "IV temp log"() -> (w2188:cluster{dbl[], dbl[]}[])
                          n1436 = Bundle By Name(cluster=w2172, "Comment"=w2171) -> (w2170:T2)
                          n1437 = local read "iteration"() -> (w2169:i32)
                          n1438 = Bundle("V fine"=w2180, w2187) -> (w2185:cluster{"V fine":dbl[], dbl[]})  [unwired: 1 in]
                          n1439 = Bundle("V fine"=w2180, "I fine"=w2186) -> (w2190:cluster{"V fine":dbl[], "I fine":dbl[]})  [unwired: 1 in]
                          n1440 = local write "Wafer Info 3"(w2170) -> ()
                          n1441 = Replace Array Subset(array=w2188, new element=w2185, index=w2169) -> (w2189:cluster{dbl[], dbl[]}[])
                          n1442 = Replace Array Subset(array=w2192, new element=w2190, index=w2169) -> (w2191:cluster{dbl[], dbl[]}[])
                          n1443 = Decimal String To Number(string=w2166) -> (number=w2165:i32)  [unwired: 2 in, 1 out]
                          n1444 = local read "current y"() -> (w2176:i32)
                          n1445 = local read "current x"() -> (w2177:i32)
                          n1446 = local write "IV temp log"(w2189) -> ()
                          n1447 = local write "IV temp linear"(w2191) -> ()
                          n1448 = Number To Decimal String(number=w2165) -> (decimal integer string=w2164:string)  [unwired: 1 in]
                          n1449 = local read "Device Name"() -> (w2182:string)
                          n1450 = local read "Wafer Name"() -> (w2184:string)
                          n1451 = local read "Operator"() -> (w2183:string)
                          n1452 = To Double Precision Float(number=w2177) -> (double precision float=w2179:dbl)
                          n1453 = To Double Precision Float(number=w2176) -> (double precision float=w2178:dbl)
                          n1454 = Get Date/Time In Seconds() -> (seconds since 1Jan1904=w2174:timestamp)
                          n1455 = Concatenate Strings(w2164, " C" ("string")) -> (w2167:string)
                          n1456 = call "get Flash FileName .vi"("Time"=w2174, "Device Name"=w2182, "Operator"=w2183, "Wafer Name"=w2184, "FineTest save path"=w2173) -> ("appended path"=w2181:path)  [unwired: 6 in]
                          n1457 = Bundle(w2179, w2178) -> (w2175:cluster{dbl, dbl})  [unwired: 1 in]
                        }
                        frame #7 {
                          n1458 = Increment(x=w2194) -> (x+1=w2193:i32)
                          n1459 = property on="IV temp linear" class="XYGraph (strict)"("Active Plot"=w2194, "Plot.Plot Name"=w2195, "LegNumRows"=w2193) -> ()  [unwired: 2 in, 2 out]
                          n1460 = property on="IV temp log" class="XYGraph (strict)"("Active Plot"=w2194, "Plot.Plot Name"=w2195, "LegNumRows"=w2193) -> ()  [unwired: 2 in, 2 out]
                        }
                        frame #8 {
                          n1461 = local read "V fine"() -> (w2213:dbl[])
                          n1462 = local read "I fine"() -> (w2214:dbl[])
                          n1463 = local read "Parameters Flash"() -> (w2211:T4)
                          n1464 = local read "Wafer Info 3"() -> (w2202:T2)
                          n1465 = local read "Temp Data"() -> (w2203:T1)
                          n1466 = local read "Current Session"() -> (w2199:timestamp)
                          n1467 = local read "Operator"() -> (w2200:string)
                          n1468 = local read "RecipeID"() -> (w2201:string)
                          n1469 = Build Array(w2213, w2214) -> (w2212:dbl[][])
                          n1470 = Get Date/Time String(seconds (now)=w2209, want seconds? (F)=TRUE) -> (date string=w2208:string, time string=w2206:string)  [unwired: 1 in]
                          n1471 = local read "Mask"() -> (w2215:string)
                          n1472 = call <vilib>:"Space Constant.vi"() -> ("String"=w2205:string)
                          n1473 = Concatenate Strings(w2208, w2205, w2206) -> (w2204:string)
                          n1474 = call "WriteFlashFile NEW.vi"("Input File Path"=w2216, "IV array"=w2212, "Current Session"=w2199, "Parameters"=w2211, "RecipeID"=w2201, "User"=w2200, "Coords"=w2210, "Wafer Info"=w2202, "Mask Name"=w2215, "Temp Data"=w2203, "Die Number"=w2204) -> ()  [unwired: 16 in, 1 out]
                        }
                      }
                    }
                  }
                  "iteration" <- w1979
                }
              }
              frame #2 {
                w2229 = -1 ("x")
                n1475 = local read "Temptronics VISA"() -> (w2218:refnum<visa-resource-name>)
                n1476 = local read "Prober GPIB"() -> (w2225:string)
                n1477 = local read "current y"() -> (w2228:i32)
                n1478 = local read "current x"() -> (w2227:i32)
                n1479 = Multiply(x=w2228, y=w2229) -> (x*y=w2231:i32)
                n1480 = Multiply(x=w2229, y=w2227) -> (x*y=w2230:i32)
                n1481 = call "EG2001 Move Z Down.vi"("GPIB Address"=w2225) -> ("Error Out"=w2226:errorcluster, "GPIB Address Out"=w2224:string)  [unwired: 9 in]
                n1482 = VISA Write(VISA resource name=w2218, write buffer="rs25" ("string")) -> (VISA resource name out=w2219:refnum<visa-resource-name>)  [unwired: 1 in, 2 out]
                n1483 = VISA Write(VISA resource name=w2219, write buffer="st") -> (VISA resource name out=w2221:refnum<visa-resource-name>, return count=w2222:u32)  [unwired: 1 in, 1 out]
                n1484 = call "EG2001 Move Machine Step X-Y.vi"("Flip X Coordinates?"=FALSE, "Y"=w2231, "Steps/Microns"=enum32{"Steps", "Microns"}."Microns", "X"=w2230, "error in (no error)"=w2226, "GPIB Address"=w2224) -> ()  [unwired: 4 in, 2 out]
                n1485 = VISA Read(VISA resource name=w2221, byte count=w2222) -> (read buffer=w2223:string)  [unwired: 1 in, 3 out]
                n1486 = local write "Current Temp"(w2223) -> ()
              }
              frame #3 {
                w2235 = 0 ("current x")
                n1487 = local write "current y"(w2235) -> ()
                n1488 = local write "current x"(w2235) -> ()
                n1489 = local write "Status"("idle" ("Status")) -> ()
              }
            }
          }
          frame "add temp auto" {
            n1490 = local read "Auto Temp Set"() -> (w2240:dbl)
            n1491 = property on="Auto Temperature List" class="LstBox (strict)"() -> ("Item Names"=w2238:string[])  [unwired: 2 in, 2 out]
            n1492 = Format Into String(format string="%08.4f", w2240) -> (resulting string=w2237:string)  [unwired: 2 in, 1 out]
            n1493 = Build Array (concatenate)(w2238, w2237) -> (w2236:string[])
            n1494 = property on="Auto Temperature List" class="LstBox (strict)"("Item Names"=w2236) -> ()  [unwired: 2 in, 2 out]
          }
          frame "remove temp auto" {
            n1495 = local read "Auto Temperature List"() -> (w2243:i32)
            n1496 = property on="Auto Temperature List" class="LstBox (strict)"() -> ("Item Names"=w2245:string[])  [unwired: 2 in, 2 out]
            n1497 = Delete From Array(array=w2245, index=w2243) -> (array with subset deleted=w2244:string[])  [unwired: 1 in, 1 out]
            n1498 = property on="Auto Temperature List" class="LstBox (strict)"("Item Names"=w2244) -> ()  [unwired: 2 in, 2 out]
          }
          frame "clear temp auto" {
            n1499 = property on="Auto Temperature List" class="LstBox (strict)"("Item Names"=string[] []) -> ()  [unwired: 2 in, 2 out]
          }
          frame "explore data" {
          }
          frame "new session" {
            n1500 = Get Date/Time In Seconds() -> (seconds since 1Jan1904=w2254:timestamp)
            n1501 = local write "Current Session"(w2254) -> ()
            n1502 = local read "Session Info"() -> (w2255:T7)
            n1503 = Bundle By Name(cluster=w2255, "Session Time"=w2254) -> (w2253:T7)
            n1504 = local write "Session Info"(w2253) -> ()
          }
        }
      }
      n1505 = Release Queue(queue=w36, force destroy? (F)=TRUE, error in (no error)=w27) -> (error out=→"error out":errorcluster)  [unwired: 2 out]
    }
  }
